vi "Volume Sievert_auto_RLC-CRZPhi.vi"() -> ()   [LabVIEW 2011]
uses:
  <vilib>/Utility/error.llb/DialogType.ctl
  <vilib>/DAQmx/write.llb/DAQmx Write (Digital Bool 1Line 1Point).vi
  <vilib>/DAQmx/create/channels.llb/DAQmx Create Channel (DO-Digital Output).vi
  <vilib>/DAQmx/miscellaneous.llb/DAQmx Fill In Error Info.vi
  <vilib>/Analysis/Matrix/Numeric/Conversions/Array To Matrix - RA.vi
  <vilib>/Analysis/Matrix/Numeric/Conversions/Matrix To Array - RM.vi
  <vilib>/Analysis/NI_AALPro.lvlib
  <vilib>/Analysis/Matrix/NI_Matrix.lvlib
  <vilib>/Analysis/NI_AALBase.lvlib
panel:
  out "S#1_auto":dbl
  out "S#01":dbl
  out "output array 3":u32[](array[numeric])
  out "PCh1 2":dbl[](array[numeric])
  out "tempo carga 2":dbl[](array[numeric])
  out "path RLC_mean 2":path
  out "MEASURE R [Ohm ]":dbl
  out "tempo carga":dbl[](array[numeric])
  out "PCh1":dbl[](array[numeric])
  out "output array 2":u32[](array[numeric])
  out "MEASURE C [F ]":dbl
  out "Automatico 2":dynamicdata(graph)
  out "termopar K 2":dbl format="%.3g"
  out "termopar K":string
  out "output NTC":dbl
  out "termopar K":dbl format="%.3g"
  out "path RLC_mean":path
  out "estagio 5":i32
  out "FIM":bool=TRUE
  out "limpo":i32
  in  "N fit":i32=5
  in  "ATM wait":u32
  in  "SET":i32
  in  "time subarray":dbl[](array[numeric])
  out "P cinetica mean 2":dbl format="%0.2f"
  out "T cinetica mean 3":dbl format="%0.2f"
  out "Time cinetica":dbl format="%0.2f"
  in  "T subarray 3":dbl[](array[numeric])
  in  "P T  index 2":i32
  in  "P subarray 2":dbl[](array[numeric])
  in  "Numeric":dbl=4.0
  in  "T subarray 2":dbl[](array[numeric])
  out "T cinetica mean 2":dbl format="%0.2f"
  out "P cinetica mean":dbl format="%0.2f"
  in  "P subarray":dbl[](array[numeric])
  in  "P T  index":i32
  out "T string":string
  out "P string":string
  out "path 2_cinetica":path
  out "Polynomial Coefficients 2":dbl[](array[numeric])
  out "Polynomial Coefficients":dbl[](array[numeric])
  in  "Count SET":i32=-1
  out "Set atual":i32
  out "mean pressure":dbl format="%.4p"
  out "Set number":i32
  in  "Tab Control":T1(tab)
  out "T":bool
  out "ZPf2":bool
  out "Pf2":bool
  out "Pit":bool
  out "ZPit":bool
  out "Camara":dbl(slide) scale=0.0..59.5 scale format="%#_3g"
  in  "Save manual":bool
  in  "Open Button":bool
  out "String 2":string
  in  "ATM":bool
  in  "Câmara":bool
  in  "Vácuo":bool
  in  "Entrada Gás":bool
  in  "Manual Ctrl":bool
  in  "stop":bool
  out "P-manual":dynamicdata(graph)
  in  "Clear":bool
  out "path":path
  in  "Nota":string
  in  "Sample name":string
  in  "File name":string
  out "Linear Model Graph":dbl[][](graph)
  out "Linear Model Graph 2":dbl[][](graph)
  in  "N to fit":i32=60
  out "N":i32
  out "Vácuo":bool
  out "Atm":bool
  out "Câmara":bool
  out "String_cinetica":string
  out "Vol Ref":dbl(slide) scale=0.0..60.0 scale format="%#_4f"
  out "Entrada gás":bool
  in  "Guardar\nCinetica":bool
  out "p fit":dbl format="%#_4g"
  out "T fit":dbl format="%#_4g"
  in  "Open Button 2":bool
  out "x >= y?":bool
  in  "seconds":dbl
  out "Elapsed Time (sec)":dbl format="%.1f"
  out "bar/N":dbl format="%#_4p"
  in  "correção NTC":dbl
  out "mean H2 sensor (V)":dbl format="%#_4p"
  out "Boolean 3":bool
  out "String 3":string
  out "T 2":bool
  out "ZPit 2":bool
  out "Pit 2":bool
  out "Pf2 2":bool
  out "ZPf2 2":bool
  out "Camara 2":dbl(slide) scale=0.0..18.0 scale format="%#_3g"
  out "Vácuo 2":bool
  out "Atm 2":bool
  out "Câmara 2":bool
  out "Vol Ref 3":dbl(slide) scale=0.0..50.0 scale format="%#_4f"
  out "Entrada gás 2":bool
  in  "Auto Ctrl":bool
  in  "Play Button":bool
  out "time stamp":timestamp format="%<%.2X>T"
  out "Time (sec)":dbl format="%.1f"
  in  "clear":bool
  out "Automatico":dynamicdata(graph)
  out "Linear P":T2(graph)
  out "Linear T":T2(graph)
  out "Contador":i32
  in  "STOP (bar/s)":dbl format="%#_5p"
  out "P (bar/s)":dbl format="%#_5p"
  out "bar/s":dbl format="%#_4p"
  out "P fit":dbl format="%#_4g"
  out "T fit":dbl format="%#_4g"
  out "x = y?":bool
  out "teste slope":i32
  in  "Set P auto":dbl
  in  "Step P":dbl=2.0
  in  "P_max":dbl=2.0
  in  "P_max camara":dbl=2.0
  out "Carga":bool=TRUE
  out "Descarga":bool
  out "String":string
  in  "P_min descarga":dbl
  in  "Boolean":bool
  in  "Array":dbl[](array[numeric])
  out "Boolean 2":bool
  out "Desc SET":i32
  in  "ZPf2 time":dbl=24.0
  in  "Ciclos":dbl
  out "Efetuados":dbl
  in  "patamar milliseconds to wait":u32=500
  in  "N fit patamar":i32=100
  in  "Step ZPit":dbl
  out "Read ZPit":bool
  in  "Estagio auto":i32
  out "mean H2 sensor":dbl format="%#_4p"
  in  "Ntest":i32=5
  in  "N fit 2":i32=100
  out "mean 18":dbl format="%.3p"
  out "mean 17":dbl format="%.3p"
  in  "C50L":bool
  in  "C50N":bool
  in  "C100L":bool
  in  "C100N":bool
  in  "C1KL":bool
  in  "C1KN":bool
  in  "C10KL":bool
  in  "C10KN":bool
  out "String 4":string
  in  "Combo Box":string(combo)
  in  "Refresh Button":bool
  in  "Close RLC 2":bool
  in  "RLC on/off":bool
  out "mean 16":dbl format="%.3p"
  out "mean 15":dbl format="%.3p"
  out "mean 14":dbl format="%.3p"
  out "mean 13":dbl format="%.3p"
  out "mean 12":dbl format="%.3p"
  out "mean 11":dbl format="%.3p"
  out "mean 10":dbl format="%.3p"
  out "mean 9":dbl format="%.3p"
  out "mean 8":dbl format="%.3p"
  out "mean 7":dbl format="%.3p"
  out "mean 6":dbl format="%.3p"
  out "mean 5":dbl format="%.3p"
  out "mean 4":dbl format="%.3p"
  out "mean 3":dbl format="%.3p"
  out "mean 2":dbl format="%.3p"
  out "mean":dbl format="%.3p"
  out "SET 2":dbl
  out "C-50-L":bool
  out "MEASURE B":dbl
  out "MEASURE A":dbl
  out "C-50-N":bool
  out "MEASURE B 2":dbl
  out "MEASURE A 2":dbl
  out "C-100-L":bool
  out "MEASURE B 3":dbl
  out "MEASURE A 3":dbl
  out "C-100-N":bool
  out "MEASURE B 4":dbl
  out "MEASURE A 4":dbl
  out "C-1K-L":bool
  out "MEASURE B 5":dbl
  out "MEASURE A 5":dbl
  out "C-1K-N":bool
  out "MEASURE B 6":dbl
  out "MEASURE A 6":dbl
  out "C-10K-L":bool
  out "MEASURE B 7":dbl
  out "MEASURE A 7":dbl
  out "C-10K-N":bool
  out "MEASURE B 8":dbl
  out "MEASURE A 8":dbl
  out "Z-50-L":bool
  out "MEASURE B 9":dbl
  out "MEASURE A 9":dbl
  out "Z-50-N":bool
  out "MEASURE B 10":dbl
  out "MEASURE A 10":dbl
  out "Z-100-L":bool
  out "MEASURE B 11":dbl
  out "MEASURE A 11":dbl
  out "Z-100-N":bool
  out "MEASURE B 12":dbl
  out "MEASURE A 12":dbl
  out "Z-1K-L":bool
  out "MEASURE B 13":dbl
  out "MEASURE A 13":dbl
  out "Z-1K-N":bool
  out "MEASURE B 14":dbl
  out "MEASURE A 14":dbl
  out "Z-10K-L":bool
  out "MEASURE B 15":dbl
  out "MEASURE A 15":dbl
  out "Z-10K-N":bool
  out "MEASURE B 16":dbl
  out "MEASURE A 16":dbl
  out "RLC300 - digimess":string
  in  "Time RLC":u32=5000
  in  "Ligar RLC":bool
  out "path RLC_completo":path
  out "Waveform Chart P 2":dbl[][](graph)
  out "Waveform Chart":dynamicdata(graph)
  in  "graph RLC":bool
  in  "Refresh Button 2":bool
  in  "Z50L":bool
  in  "Z50N":bool
  in  "Z100L":bool
  in  "Z100N":bool
  in  "Z1KL":bool
  in  "Z1KN":bool
  in  "Z10KL":bool
  in  "Z10KN":bool
  out "T(º) FIT":dbl
  out "Waveform Chart 2":dynamicdata(graph)
  out "XY Graph 2":cluster{"Value":dbl[], "Value":dbl[]}[](graph)
  in  "t-sivert01(s)":dbl
  out "dP/dt (bar/s)":dbl format="%#_5p"
  in  "Save - Sievert 01":bool
  in  "File name 2":string
  in  "Nota 01":string
  in  "Sample name 2":string
  in  "Save S#1":bool
  out "path 2":path
  out "Boolean 4":bool
  out "P(bar) FIT":dbl
  in  "ON/OFF":bool
  in  "Refresh Button 3":bool
  # "P vol ref"
  # "P Câmara"
  # "P vol ref"
  # "P Câmara"
  # "C ( F )"
  # "R ( Ohm )"
  # "Z ( Ohm )"
  # "Phase ( deg)"
types:
  T1 = enum32{"Manual", "Automatico", "RLC - CDH2", "Sievert 01"}
  T2 = cluster{"Real 2D Array":dbl[], "Best Linear Fit":dbl[]}[]
  T3 = enum16{"open", "replace", "create", "open or create", "replace or create", "replace or create with confirmation"}
  T4 = typedef "DialogType.ctl" = u16
  T5 = cluster{"Value":dbl[], "Best Polynomial Fit":dbl[]}
  T6 = cluster{"Value":dbl[], "Best Polynomial Fit":dbl[]}[]
  T7 = typedef "NI_Matrix.lvlib/RealMatrix.ctl" = dbl[][]
  T8 = cluster{"Real 2D Array":dbl[], "Real 2D Array":dbl[]}
  T9 = cluster{"Real 2D Array":dbl[], "Best Linear Fit":dbl[]}
  T10 = cluster{"Real 2D Array":dbl[], "Best Polynomial Fit":dbl[]}
  T11 = cluster{"Real 2D Array":dbl[], "Best Polynomial Fit":dbl[]}[]
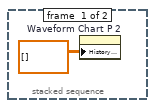
[diagram p7: hidden frame]
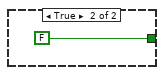
[diagram p12: hidden frame]
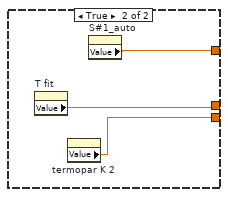
[diagram p15: hidden frame]
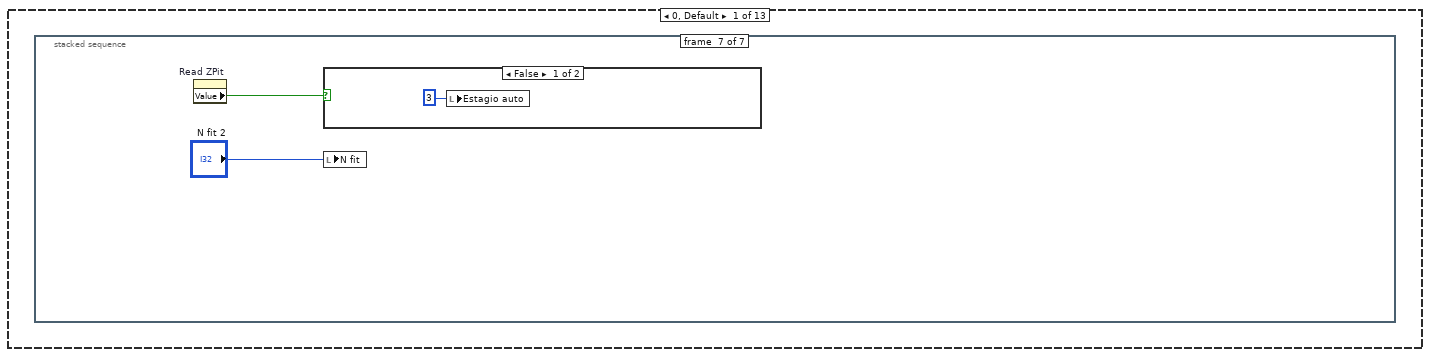
[diagram p20: hidden frame]
diagram:
  w2 = TRUE ("C1KN")
  (unwired) dbl[] [0.5, 1.0, 2.0, 3.0, 4.0, 5.0, 6.0, 7.0, 8.0, 9.0, 10.0, 11.0, 12.0, 13.0, 14.0, 15.0, 16.0, 17.0, 18.0, 19.0, 20.0, 30.0, 40.0, 50.0, 60.0, 70.0] ("Array")
  n1 = local write "N to fit"(5 ("Numeric")) -> ()
  n2 = local write "Step ZPit"(5.0 ("Step ZPit")) -> ()
  n3 = local write "Time RLC"(u32 5 ("Time RLC")) -> ()
  n4 = local write "Ciclos"(0.0 ("Ciclos")) -> ()
  n5 = local write "Desc SET"(0 ("Desc SET")) -> ()
  n6 = local write "Efetuados"(0.0 ("Efetuados")) -> ()
  n7 = local write "estagio 5"(0 ("estagio 5")) -> ()
  n8 = local write "teste slope"(0 ("teste slope")) -> ()
  n9 = local write "SET"(0 ("SET auto")) -> ()
  n10 = local write "limpo"(0 ("limpo")) -> ()
  n11 = local write "N fit"(5 ("N fit")) -> ()
  n12 = local write "ATM wait"(u32 4 ("ATM wait")) -> ()
  n13 = local write "Estagio auto"(0 ("Estagio auto")) -> ()
  n14 = local write "P T  index"(0 ("index")) -> ()
  n15 = local write "seconds"(2.0 ("seconds")) -> ()
  n16 = local write "C1KN"(w2) -> ()
  n17 = local write "Z1KN"(w2) -> ()
  n18 = local write "Read ZPit"(TRUE ("Read ZPit")) -> ()
  n19 = local write "Descarga"(FALSE ("Descarga")) -> ()
  n20 = local write "Carga"(TRUE ("Carga")) -> ()
  n21 = local write "FIM"(FALSE ("FIM")) -> ()
  n22 = local write "t-sivert01(s)"(10.0 ("t-sivert01(s)")) -> ()
  n23 = local write "P_max"(50.0 ("P_max")) -> ()
  n24 = local write "P_max camara"(25.0 ("P_max camara")) -> ()
  n25 = local write "correção NTC"(0.5 ("correção NTC")) -> ()
  n26 = local write "Set P auto"(0.5 ("Set P auto")) -> ()
  n27 = local write "P_min descarga"(0.025 ("P_min descarga")) -> ()
  n28 = local write "Array"(dbl[] [0.5, 1.0, 2.0, 3.0, 4.0, 4.0, 4.0, 4.0, 4.0, 4.0, 4.0, 5.0, 5.0, 5.0, 7.0, 10.0, 15.0, 20.0, 25.0, 25.0, 25.0, 30.0, 40.0, 50.0, 60.0, 70.0] ("Array")) -> ()
  n29 = local write "P subarray"(dbl[] [0.0, 1.0] ("subarray")) -> ()
  n30 = local write "T subarray 2"(dbl[] [0.0, 1.0] ("subarray")) -> ()
  n31 = local write "Combo Box"("rlc_read_cCN.py" ("Combo Box")) -> ()
  n32 = while {
    tunnel: path "C:/H2_Painel/painel_auto/RLC_CDH" ("Path") -> [w40]
    stop <- w52 stop-if-true
    n33 = property on="FIM" class="Bool (strict)"() -> ("Value"=w50:bool)  [unwired: 2 in, 2 out]
    n34 = property on="path" class="Path"() -> ("Value"=w47:path)  [unwired: 2 in, 2 out]
    n35 = case shown="True" "Ligar RLC" {
      tunnel: w40 -> [_ w231]
      frame False {
      }
      frame True {
        n36 = call "RLC_open.vi"("Path"=w231) -> ("String 2"=w232:string)  [unwired: 9 in, 1 out]
        n37 = local write "RLC300 - digimess"(w232) -> ()
      }
    }
    n38 = case shown="True" "RLC on/off" {
      tunnel: w40 -> [_ _]
      frame False {
      }
      frame True {
        n39 = call "RLC READ DINAMICO.vi"("Boolean"="graph RLC") -> ("MEASURE R [Ohm ]"=w66:dbl, "MEASURE C [F ]"=w65:dbl)  [unwired: 9 in]
        "MEASURE C [F ]" <- w65
        "MEASURE R [Ohm ]" <- w66
        n40 = Merge Signals(w65, w66) -> (→"Waveform Chart":dynamicdata)
        "String 4" <- "Combo Box"
      }
    }
    n41 = case shown="True" "Manual Ctrl" {
      tunnel: w40 -> [_ w1841]
      tunnel: "RLC on/off" -> [_ w1840]
      tunnel: [FALSE w1843] -> w42
      frame False {
      }
      frame True {
        w1855 = 0 ("polynomial order")
        n42 = case shown="True" "Save manual" {
          selector: "Save manual" -> [_ w2457]
          frame False {
          }
          frame True {
            n43 = feedback #1() -> (w2453:dbl)  [unwired: 1 in]
            n44 = Equal To 0?(x=w2453) -> (x = 0?=w2459:bool)
            n45 = stacked-sequence {
              tunnel: w2459 -> [_ w2475 _]
              tunnel: [_ w2474 _] -> w2455
              frame #0 {
                w2468 = i16 3 ("precision (6)")
                n46 = property on="T fit" class="DigNum (strict)"() -> ("Value"=w2470:dbl)  [unwired: 2 in, 2 out]
                n47 = property on="p fit" class="DigNum (strict)"() -> ("Value"=w2471:dbl)  [unwired: 2 in, 2 out]
                n48 = property on="termopar K" class="DigNum (strict)"() -> ("Value"=w2469:dbl)  [unwired: 2 in, 2 out]
                n49 = Number To Fractional String(number=w2470, precision (6)=w2468) -> (F-format string=→"T string":string)  [unwired: 2 in]
                n50 = Number To Fractional String(number=w2471, precision (6)=w2468) -> (F-format string=→"P string":string)  [unwired: 2 in]
                n51 = Number To Fractional String(number=w2469, precision (6)=w2468) -> (F-format string=→"termopar K":string)  [unwired: 2 in]
              }
              frame #1 {
                n52 = case shown="True" w2475 {
                  tunnel: [TRUE ("y") FALSE ("y")] -> w2474
                  frame False {
                    n53 = property on="path" class="Path"() -> ("Value"=w2479:path)  [unwired: 2 in, 2 out]
                    n54 = property on="P string" class="Str"() -> ("Value"=w2478:string)  [unwired: 2 in, 2 out]
                    n55 = Concatenate Strings(w2478, "\t") -> (w2476:string)
                    n56 = Open/Create/Replace File(file path (use dialog)=w2479, operation (0:open)=T3."open") -> (refnum out=w2483:refnum<file>, error out=w2482:errorcluster)  [unwired: 2 in, 3 out]
                    n57 = Set File Position(refnum=w2483, from (0:start)=enum16{"start", "end", "current"}."end", error in=w2482) -> (refnum out=w2485:refnum<file>, error out=w2486:errorcluster)  [unwired: 1 in]
                    n58 = Write to Text File(file (use dialog)=w2485, text=w2476, error in=w2486) -> (refnum out=w2481:refnum<file>, error out=w2480:errorcluster)  [unwired: 2 out]
                    n59 = Close File(refnum=w2481, error in=w2480) -> (error out=w2488:errorcluster)  [unwired: 1 out]
                    n60 = call <vilib>:"Simple Error Handler.vi"("error in (no error)"=w2488) -> ()  [unwired: 1 in, 8 out]
                  }
                  frame True {
                    w2491 = "\t"
                    n61 = property on="path" class="Path"() -> ("Value"=w2498:path)  [unwired: 2 in, 2 out]
                    n62 = property on="Count SET" class="DigNum (strict)"() -> ("Value"=w2494:i32)  [unwired: 2 in, 2 out]
                    n63 = Open/Create/Replace File(file path (use dialog)=w2498, operation (0:open)=T3."open") -> (refnum out=w2497:refnum<file>, error out=w2496:errorcluster)  [unwired: 2 in, 3 out]
                    n64 = Increment(x=w2494) -> (x+1=w2495:i32)
                    "Set atual" <- w2495
                    n65 = Set File Position(refnum=w2497, from (0:start)=enum16{"start", "end", "current"}."end", error in=w2496) -> (refnum out=w2506:refnum<file>, error out=w2507:errorcluster)  [unwired: 1 in]
                    n66 = Number To Decimal String(number=w2495) -> (decimal integer string=w2499:string)  [unwired: 1 in]
                    n67 = property on="termopar K" class="Str"() -> ("Value"=w2490:string)  [unwired: 2 in, 2 out]
                    n68 = property on="T string" class="Str"() -> ("Value"=w2492:string)  [unwired: 2 in, 2 out]
                    n69 = Concatenate Strings(w2492, w2491, w2490, "\r\n", w2499, w2491) -> (w2501:string)
                    n70 = Write to Text File(file (use dialog)=w2506, text=w2501, error in=w2507) -> (refnum out=w2504:refnum<file>, error out=w2503:errorcluster)  [unwired: 2 out]
                    n71 = Close File(refnum=w2504, error in=w2503) -> (error out=w2509:errorcluster)  [unwired: 1 out]
                    n72 = call <vilib>:"Simple Error Handler.vi"("error in (no error)"=w2509) -> ()  [unwired: 1 in, 8 out]
                    "T" <- TRUE ("T")
                  }
                }
              }
              frame #2 {
                n73 = property on="path" class="Path"() -> ("Value"=w2511:path)  [unwired: 2 in, 2 out]
                n74 = property on="Set atual" class="DigNum (strict)"() -> ("Value"=w2510:i32)  [unwired: 2 in, 2 out]
                n75 = local write "Count SET"(w2510) -> ()
                n76 = Read from Text File(file (use dialog)=w2511, count=-1 ("Count  3")) -> (refnum out=w2513:refnum<file>, text=w2512:string, error out=w2514:errorcluster)  [unwired: 2 in, 1 out]
                n77 = property on="String 2" class="Str"("Value"=w2512) -> ()  [unwired: 2 in, 2 out]
                n78 = Close File(refnum=w2513, error in=w2514) -> (error out=w2516:errorcluster)  [unwired: 1 out]
                n79 = call <vilib>:"Simple Error Handler.vi"("error in (no error)"=w2516) -> ()  [unwired: 1 in, 8 out]
              }
            }
            n80 = Implies(1:w2455, 2:w2457) -> (0:w2456:bool)
            n81 = Select(t=w2453, s=w2456, f=5.0 ("t")) -> (s? t:f=w2454:dbl)
            n82 = case shown="1" w2454 {
              frame 0, Default {
              }
              frame 1 {
                "ZPf2" <- TRUE ("ZPf2")
              }
              frame 2 {
                "Pf2" <- TRUE ("Pf2")
              }
              frame 3 {
                "Pit" <- TRUE ("Pit")
              }
              frame 4 {
                n83 = local write "T"(FALSE ("T")) -> ()
                "ZPit" <- TRUE ("ZPit")
              }
              frame 5 {
                w2466 = FALSE
                n84 = local write "Pit"(w2466) -> ()
                n85 = local write "ZPf2"(w2466) -> ()
                n86 = local write "ZPit"(w2466) -> ()
                n87 = local write "Pf2"(w2466) -> ()
              }
            }
            n88 = Decrement(x=w2454) -> (x-1=w2460:dbl)
            n89 = feedback-in #1(w2460) -> ()
          }
        }
        n90 = case shown="True" w1840 {
          tunnel: [FALSE ("Save manual") w2452] -> w1842
          tunnel: "Save manual" -> [_ w2452]
          frame False {
          }
          frame True {
          }
        }
        n91 = case shown="True" w1840 {
          tunnel: [FALSE w1860] -> w1843
          tunnel: w1842 -> [_ w1859]
          tunnel: w1841 -> [_ w1858]
          frame False {
          }
          frame True {
            n92 = flat-sequence {
              tunnel: w1858 -> [w1881]
              tunnel: w1859 -> [w1882]
              tunnel: [w1882] -> w1879
              tunnel: [w1881] -> w1878
              tunnel: [w1889] -> w1877
              tunnel: [w1890] -> w1876
              tunnel: [w1891] -> w1875
              tunnel: [w1892] -> w1874
              tunnel: [w1893] -> w1873
              tunnel: [w1894] -> w1872
              tunnel: [w1895] -> w1871
              tunnel: [w1897] -> w1870
              tunnel: [w1898] -> w1869
              tunnel: [w1899] -> w1868
              tunnel: [w1900] -> w1867
              tunnel: [w1901] -> w1866
              tunnel: [w1896] -> w1865
              tunnel: [w1888] -> w1864
              tunnel: [w1887] -> w1863
              tunnel: [w1886] -> w1862
              tunnel: [w1885] -> w1861
              tunnel: w1879 -> [w1884]
              tunnel: w1878 -> [w1883]
              tunnel: w1877 -> [w2399]
              tunnel: w1876 -> [w2398]
              tunnel: w1875 -> [w2397]
              tunnel: w1874 -> [w2396]
              tunnel: w1873 -> [w2395]
              tunnel: w1872 -> [w2394]
              tunnel: w1871 -> [w2393]
              tunnel: w1870 -> [w2392]
              tunnel: w1869 -> [w2391]
              tunnel: w1868 -> [w2390]
              tunnel: w1867 -> [w2389]
              tunnel: w1866 -> [w2388]
              tunnel: w1865 -> [w2387]
              tunnel: w1864 -> [w2400]
              tunnel: w1863 -> [w2401]
              tunnel: w1862 -> [w2402]
              tunnel: [w2385] -> w1860
              tunnel: w1861 -> [w2385]
              tunnel: [TRUE] -> w1857
              frame #0 {
                n93 = local write "graph RLC"(FALSE) -> ()
              }
              frame #1 {
                n94 = case shown="True" w1884 {
                  tunnel: [_ w1936] -> w1885
                  tunnel: w1883 -> [_ w1918]
                  tunnel: [_ w1917] -> w1886
                  tunnel: [_ w1916] -> w1887
                  tunnel: [_ w1915] -> w1888
                  tunnel: [_ w1914] -> w1889
                  tunnel: [_ w1913] -> w1890
                  tunnel: [_ w1912] -> w1891
                  tunnel: [_ w1911] -> w1892
                  tunnel: [_ w1910] -> w1893
                  tunnel: [_ w1909] -> w1894
                  tunnel: [_ w1908] -> w1895
                  tunnel: [_ w1907] -> w1896
                  tunnel: [_ w1906] -> w1897
                  tunnel: [_ w1905] -> w1898
                  tunnel: [_ w1904] -> w1899
                  tunnel: [_ w1903] -> w1900
                  tunnel: [_ w1902] -> w1901
                  frame False {
                  }
                  frame True {
                    n95 = for {
                      N: 5 -> [_]
                      tunnel: TRUE -> [w1959]
                      tunnel: FALSE -> [w1958]
                      tunnel: [w1957] -> w1936
                      tunnel: [w1956] -> w1934 mode=indexing
                      tunnel: [w1955] -> w1933 mode=indexing
                      tunnel: [w1954] -> w1932 mode=indexing
                      tunnel: [w1953] -> w1931 mode=indexing
                      tunnel: [w1952] -> w1930 mode=indexing
                      tunnel: [w1951] -> w1929 mode=indexing
                      tunnel: [w1950] -> w1928 mode=indexing
                      tunnel: [w1949] -> w1927 mode=indexing
                      tunnel: [w1948] -> w1926 mode=indexing
                      tunnel: [w1947] -> w1925 mode=indexing
                      tunnel: [w1946] -> w1924 mode=indexing
                      tunnel: [w1945] -> w1923 mode=indexing
                      tunnel: [w1944] -> w1922 mode=indexing
                      tunnel: [w1943] -> w1921 mode=indexing
                      tunnel: [w1942] -> w1920 mode=indexing
                      tunnel: [w1941] -> w1919 mode=indexing
                      tunnel: w1918 -> [w1940]
                      n96 = property on="path RLC_completo" class="Path"() -> ("Value"=w1939:path)  [unwired: 2 in, 2 out]
                      n97 = stacked-sequence {
                        tunnel: w1959 -> [_ w1984 w2009 w2034 w2059 w2084 w2109 w2134 w2157 w2182 w2209 w2232 w2259 w2284 w2309 w2332 w2359 _]
                        tunnel: w1958 -> [w1960 _ _ _ _ _ _ _ _ _ _ _ _ _ _ _ _ w2383]
                        tunnel: [_ _ _ _ _ _ _ _ _ _ _ _ _ _ _ _ _ TRUE] -> w1957
                        tunnel: [_ w1983 _ _ _ _ _ _ _ _ _ _ _ _ _ _ _ _] -> w1956
                        tunnel: [_ _ w2008 _ _ _ _ _ _ _ _ _ _ _ _ _ _ _] -> w1955
                        tunnel: [_ _ _ w2033 _ _ _ _ _ _ _ _ _ _ _ _ _ _] -> w1954
                        tunnel: [_ _ _ _ w2058 _ _ _ _ _ _ _ _ _ _ _ _ _] -> w1953
                        tunnel: [_ _ _ _ _ w2083 _ _ _ _ _ _ _ _ _ _ _ _] -> w1952
                        tunnel: [_ _ _ _ _ _ w2108 _ _ _ _ _ _ _ _ _ _ _] -> w1951
                        tunnel: [_ _ _ _ _ _ _ w2133 _ _ _ _ _ _ _ _ _ _] -> w1950
                        tunnel: [_ _ _ _ _ _ _ _ w2159 _ _ _ _ _ _ _ _ _] -> w1949
                        tunnel: [_ _ _ _ _ _ _ _ _ w2184 _ _ _ _ _ _ _ _] -> w1948
                        tunnel: [_ _ _ _ _ _ _ _ _ _ w2208 _ _ _ _ _ _ _] -> w1947
                        tunnel: [_ _ _ _ _ _ _ _ _ _ _ w2234 _ _ _ _ _ _] -> w1946
                        tunnel: [_ _ _ _ _ _ _ _ _ _ _ _ w2258 _ _ _ _ _] -> w1945
                        tunnel: [_ _ _ _ _ _ _ _ _ _ _ _ _ w2283 _ _ _ _] -> w1944
                        tunnel: [_ _ _ _ _ _ _ _ _ _ _ _ _ _ w2308 _ _ _] -> w1943
                        tunnel: [_ _ _ _ _ _ _ _ _ _ _ _ _ _ _ w2334 _ _] -> w1942
                        tunnel: [_ _ _ _ _ _ _ _ _ _ _ _ _ _ _ _ w2358 _] -> w1941
                        tunnel: w1940 -> [_ w1986 w2012 w2036 w2061 w2086 w2111 w2136 w2161 w2186 w2211 w2236 w2261 w2286 w2311 w2336 w2361 _]
                        tunnel: w1939 -> [w1962 w1985 w2011 w2035 w2060 w2085 w2110 w2135 w2160 w2185 w2210 w2235 w2260 w2285 w2310 w2335 w2360 _]
                        frame #0 {
                          w1963 = "\t"
                          n98 = local write "C-50-L"(w1960) -> ()
                          n99 = local write "C-50-N"(w1960) -> ()
                          n100 = local write "Z-50-L"(w1960) -> ()
                          n101 = local write "Z-50-N"(w1960) -> ()
                          n102 = local write "C-1K-L"(w1960) -> ()
                          n103 = local write "C-1K-N"(w1960) -> ()
                          n104 = local write "Z-1K-N"(w1960) -> ()
                          n105 = local write "Z-1K-L"(w1960) -> ()
                          n106 = local write "Z-100-L"(w1960) -> ()
                          n107 = local write "C-10K-L"(w1960) -> ()
                          n108 = local write "C-100-N"(w1960) -> ()
                          n109 = local write "C-10K-N"(w1960) -> ()
                          n110 = local write "Z-10K-N"(w1960) -> ()
                          n111 = local write "Z-10K-L"(w1960) -> ()
                          n112 = local write "Z-100-N"(w1960) -> ()
                          n113 = local write "C-100-L"(w1960) -> ()
                          n114 = Open/Create/Replace File(file path (use dialog)=w1962, operation (0:open)=T3."open") -> (refnum out=w1976:refnum<file>, error out=w1975:errorcluster)  [unwired: 2 in, 3 out]
                          n115 = Get Date/Time String(date format (0)=enum16{"short", "long", "abbreviated"}."short", want seconds? (F)=TRUE) -> (date string=w1968:string, time string=w1967:string)  [unwired: 1 in]
                          n116 = feedback #2() -> (w1961:dbl)  [unwired: 1 in]
                          n117 = local write "SET 2"(w1961) -> ()
                          n118 = Set File Position(refnum=w1976, from (0:start)=enum16{"start", "end", "current"}."end", error in=w1975) -> (refnum out=w1978:refnum<file>, error out=w1979:errorcluster)  [unwired: 1 in]
                          n119 = Number To Fractional String(number=w1961, precision (6)=i16 2) -> (F-format string=w1966:string)  [unwired: 2 in]
                          n120 = Add(x=w1961, y=0.2) -> (x+y=w1972:dbl)
                          n121 = feedback-in #2(w1972) -> ()
                          n122 = Concatenate Strings(w1966, w1963, w1968, w1963, w1967, w1963) -> (w1965:string)
                          n123 = Write to Text File(file (use dialog)=w1978, text=w1965, error in=w1979) -> (refnum out=w1974:refnum<file>, error out=w1973:errorcluster)  [unwired: 1 in, 1 out]
                          n124 = Close File(refnum=w1974, error in=w1973) -> (error out=w1981:errorcluster)  [unwired: 1 out]
                          n125 = call <vilib>:"Simple Error Handler.vi"("error in (no error)"=w1981) -> ()  [unwired: 1 in, 8 out]
                        }
                        frame #1 {
                          w1987 = "\t"
                          w2004 = i16 4 ("width (-)")
                          n126 = local write "C-50-L"(w1984) -> ()
                          n127 = Wait (ms)(milliseconds to wait=u32 5000) -> ()  [unwired: 1 out]
                          n128 = Open/Create/Replace File(file path (use dialog)=w1985, operation (0:open)=T3."open") -> (refnum out=w1996:refnum<file>, error out=w1995:errorcluster)  [unwired: 2 in, 3 out]
                          n129 = Set File Position(refnum=w1996, from (0:start)=enum16{"start", "end", "current"}."end", error in=w1995) -> (refnum out=w1998:refnum<file>, error out=w1999:errorcluster)  [unwired: 1 in]
                          n130 = call "RLC_read.vi"("Path"=w1986, "String"="cmd /c rlc_read_cAL.py") -> ("MEASURE A"=w1983:dbl, "MEASURE V [V]"=w2003:dbl, "MEASURE B"=w1982:dbl, "MEASURE I [A]"=w2002:dbl)  [unwired: 2 out]
                          n131 = Number To Engineering String(2:w2004, 4:w2002) -> (0:w1988:string)  [unwired: 2 in]
                          n132 = local write "MEASURE A"(w1983) -> ()
                          n133 = local write "MEASURE B"(w1982) -> ()
                          n134 = Number To Engineering String(2:w2004, 4:w2003) -> (0:w1989:string)  [unwired: 2 in]
                          n135 = Number To Engineering String(2:w2004, 4:w1983) -> (0:w1991:string)  [unwired: 2 in]
                          n136 = Number To Engineering String(2:w2004, 4:w1982) -> (0:w1990:string)  [unwired: 2 in]
                          n137 = Concatenate Strings(w1991, w1987, w1990, w1987, w1989, w1987, w1988, w1987) -> (w1992:string)
                          n138 = Write to Text File(file (use dialog)=w1998, text=w1992, error in=w1999) -> (refnum out=w1994:refnum<file>, error out=w1993:errorcluster)  [unwired: 1 in, 1 out]
                          n139 = Close File(refnum=w1994, error in=w1993) -> (error out=w2001:errorcluster)  [unwired: 1 out]
                          n140 = call <vilib>:"Simple Error Handler.vi"("error in (no error)"=w2001) -> ()  [unwired: 1 in, 8 out]
                        }
                        frame #2 {
                          w2015 = "\t"
                          w2029 = i16 4 ("width (-)")
                          n141 = local write "C-50-N"(w2009) -> ()
                          n142 = Wait (ms)(milliseconds to wait=u32 5000) -> ()  [unwired: 1 out]
                          n143 = Open/Create/Replace File(file path (use dialog)=w2011, operation (0:open)=T3."open") -> (refnum out=w2023:refnum<file>, error out=w2022:errorcluster)  [unwired: 2 in, 3 out]
                          n144 = Set File Position(refnum=w2023, from (0:start)=enum16{"start", "end", "current"}."end", error in=w2022) -> (refnum out=w2025:refnum<file>, error out=w2026:errorcluster)  [unwired: 1 in]
                          n145 = call "RLC_read.vi"("Path"=w2012, "String"="cmd /c rlc_read_cAN.py") -> ("MEASURE A"=w2008:dbl, "MEASURE V [V]"=w2014:dbl, "MEASURE B"=w2007:dbl, "MEASURE I [A]"=w2013:dbl)  [unwired: 2 out]
                          n146 = Number To Engineering String(2:w2029, 4:w2013) -> (0:w2016:string)  [unwired: 2 in]
                          n147 = local write "MEASURE A 2"(w2008) -> ()
                          n148 = local write "MEASURE B 2"(w2007) -> ()
                          n149 = Number To Engineering String(2:w2029, 4:w2014) -> (0:w2017:string)  [unwired: 2 in]
                          n150 = Number To Engineering String(2:w2029, 4:w2008) -> (0:w2019:string)  [unwired: 2 in]
                          n151 = Number To Engineering String(2:w2029, 4:w2007) -> (0:w2018:string)  [unwired: 2 in]
                          n152 = Concatenate Strings(w2019, w2015, w2018, w2015, w2017, w2015, w2016, w2015) -> (w2010:string)
                          n153 = Write to Text File(file (use dialog)=w2025, text=w2010, error in=w2026) -> (refnum out=w2021:refnum<file>, error out=w2020:errorcluster)  [unwired: 1 in, 1 out]
                          n154 = Close File(refnum=w2021, error in=w2020) -> (error out=w2028:errorcluster)  [unwired: 1 out]
                          n155 = call <vilib>:"Simple Error Handler.vi"("error in (no error)"=w2028) -> ()  [unwired: 1 in, 8 out]
                        }
                        frame #3 {
                          w2039 = "\t"
                          w2054 = i16 4 ("width (-)")
                          n156 = Wait (ms)(milliseconds to wait=u32 5000) -> ()  [unwired: 1 out]
                          n157 = local write "C-100-L"(w2034) -> ()
                          n158 = Open/Create/Replace File(file path (use dialog)=w2035, operation (0:open)=T3."open") -> (refnum out=w2048:refnum<file>, error out=w2047:errorcluster)  [unwired: 2 in, 3 out]
                          n159 = Set File Position(refnum=w2048, from (0:start)=enum16{"start", "end", "current"}."end", error in=w2047) -> (refnum out=w2050:refnum<file>, error out=w2051:errorcluster)  [unwired: 1 in]
                          n160 = call "RLC_read.vi"("Path"=w2036, "String"="cmd /c rlc_read_cBL.py") -> ("MEASURE A"=w2033:dbl, "MEASURE V [V]"=w2038:dbl, "MEASURE B"=w2032:dbl, "MEASURE I [A]"=w2037:dbl)  [unwired: 2 out]
                          n161 = Number To Engineering String(2:w2054, 4:w2037) -> (0:w2040:string)  [unwired: 2 in]
                          n162 = local write "MEASURE A 3"(w2033) -> ()
                          n163 = local write "MEASURE B 3"(w2032) -> ()
                          n164 = Number To Engineering String(2:w2054, 4:w2038) -> (0:w2041:string)  [unwired: 2 in]
                          n165 = Number To Engineering String(2:w2054, 4:w2033) -> (0:w2043:string)  [unwired: 2 in]
                          n166 = Number To Engineering String(2:w2054, 4:w2032) -> (0:w2042:string)  [unwired: 2 in]
                          n167 = Concatenate Strings(w2043, w2039, w2042, w2039, w2041, w2039, w2040, w2039) -> (w2044:string)
                          n168 = Write to Text File(file (use dialog)=w2050, text=w2044, error in=w2051) -> (refnum out=w2046:refnum<file>, error out=w2045:errorcluster)  [unwired: 1 in, 1 out]
                          n169 = Close File(refnum=w2046, error in=w2045) -> (error out=w2053:errorcluster)  [unwired: 1 out]
                          n170 = call <vilib>:"Simple Error Handler.vi"("error in (no error)"=w2053) -> ()  [unwired: 1 in, 8 out]
                        }
                        frame #4 {
                          w2064 = "\t"
                          w2079 = i16 4 ("width (-)")
                          n171 = Wait (ms)(milliseconds to wait=u32 5000) -> ()  [unwired: 1 out]
                          n172 = local write "C-100-N"(w2059) -> ()
                          n173 = Open/Create/Replace File(file path (use dialog)=w2060, operation (0:open)=T3."open") -> (refnum out=w2073:refnum<file>, error out=w2072:errorcluster)  [unwired: 2 in, 3 out]
                          n174 = Set File Position(refnum=w2073, from (0:start)=enum16{"start", "end", "current"}."end", error in=w2072) -> (refnum out=w2075:refnum<file>, error out=w2076:errorcluster)  [unwired: 1 in]
                          n175 = call "RLC_read.vi"("Path"=w2061, "String"="cmd /c rlc_read_cBN.py") -> ("MEASURE A"=w2058:dbl, "MEASURE V [V]"=w2063:dbl, "MEASURE B"=w2057:dbl, "MEASURE I [A]"=w2062:dbl)  [unwired: 2 out]
                          n176 = Number To Engineering String(2:w2079, 4:w2062) -> (0:w2065:string)  [unwired: 2 in]
                          n177 = local write "MEASURE A 4"(w2058) -> ()
                          n178 = local write "MEASURE B 4"(w2057) -> ()
                          n179 = Number To Engineering String(2:w2079, 4:w2063) -> (0:w2066:string)  [unwired: 2 in]
                          n180 = Number To Engineering String(2:w2079, 4:w2058) -> (0:w2068:string)  [unwired: 2 in]
                          n181 = Number To Engineering String(2:w2079, 4:w2057) -> (0:w2067:string)  [unwired: 2 in]
                          n182 = Concatenate Strings(w2068, w2064, w2067, w2064, w2066, w2064, w2065, w2064) -> (w2069:string)
                          n183 = Write to Text File(file (use dialog)=w2075, text=w2069, error in=w2076) -> (refnum out=w2071:refnum<file>, error out=w2070:errorcluster)  [unwired: 1 in, 1 out]
                          n184 = Close File(refnum=w2071, error in=w2070) -> (error out=w2078:errorcluster)  [unwired: 1 out]
                          n185 = call <vilib>:"Simple Error Handler.vi"("error in (no error)"=w2078) -> ()  [unwired: 1 in, 8 out]
                        }
                        frame #5 {
                          w2104 = "\t"
                          w2089 = i16 4 ("width (-)")
                          n186 = local write "C-1K-L"(w2084) -> ()
                          n187 = Wait (ms)(milliseconds to wait=u32 5000) -> ()  [unwired: 1 out]
                          n188 = Open/Create/Replace File(file path (use dialog)=w2085, operation (0:open)=T3."open") -> (refnum out=w2095:refnum<file>, error out=w2096:errorcluster)  [unwired: 2 in, 3 out]
                          n189 = Set File Position(refnum=w2095, from (0:start)=enum16{"start", "end", "current"}."end", error in=w2096) -> (refnum out=w2093:refnum<file>, error out=w2092:errorcluster)  [unwired: 1 in]
                          n190 = call "RLC_read.vi"("Path"=w2086, "String"="cmd /c rlc_read_cCL.py") -> ("MEASURE A"=w2083:dbl, "MEASURE V [V]"=w2088:dbl, "MEASURE B"=w2082:dbl, "MEASURE I [A]"=w2087:dbl)  [unwired: 2 out]
                          n191 = Number To Engineering String(2:w2089, 4:w2087) -> (0:w2103:string)  [unwired: 2 in]
                          n192 = local write "MEASURE A 5"(w2083) -> ()
                          n193 = local write "MEASURE B 5"(w2082) -> ()
                          n194 = Number To Engineering String(2:w2089, 4:w2088) -> (0:w2102:string)  [unwired: 2 in]
                          n195 = Number To Engineering String(2:w2089, 4:w2083) -> (0:w2100:string)  [unwired: 2 in]
                          n196 = Number To Engineering String(2:w2089, 4:w2082) -> (0:w2101:string)  [unwired: 2 in]
                          n197 = Concatenate Strings(w2100, w2104, w2101, w2104, w2102, w2104, w2103, w2104) -> (w2099:string)
                          n198 = Write to Text File(file (use dialog)=w2093, text=w2099, error in=w2092) -> (refnum out=w2097:refnum<file>, error out=w2098:errorcluster)  [unwired: 1 in, 1 out]
                          n199 = Close File(refnum=w2097, error in=w2098) -> (error out=w2090:errorcluster)  [unwired: 1 out]
                          n200 = call <vilib>:"Simple Error Handler.vi"("error in (no error)"=w2090) -> ()  [unwired: 1 in, 8 out]
                        }
                        frame #6 {
                          w2129 = "\t"
                          w2114 = i16 4 ("width (-)")
                          n201 = local write "C-1K-N"(w2109) -> ()
                          n202 = Wait (ms)(milliseconds to wait=u32 5000) -> ()  [unwired: 1 out]
                          n203 = Open/Create/Replace File(file path (use dialog)=w2110, operation (0:open)=T3."open") -> (refnum out=w2120:refnum<file>, error out=w2121:errorcluster)  [unwired: 2 in, 3 out]
                          n204 = Set File Position(refnum=w2120, from (0:start)=enum16{"start", "end", "current"}."end", error in=w2121) -> (refnum out=w2118:refnum<file>, error out=w2117:errorcluster)  [unwired: 1 in]
                          n205 = call "RLC_read.vi"("Path"=w2111, "String"="cmd /c rlc_read_cCN.py") -> ("MEASURE A"=w2108:dbl, "MEASURE V [V]"=w2113:dbl, "MEASURE B"=w2107:dbl, "MEASURE I [A]"=w2112:dbl)  [unwired: 2 out]
                          n206 = Number To Engineering String(2:w2114, 4:w2112) -> (0:w2128:string)  [unwired: 2 in]
                          n207 = local write "MEASURE A 6"(w2108) -> ()
                          n208 = local write "MEASURE B 6"(w2107) -> ()
                          n209 = Number To Engineering String(2:w2114, 4:w2113) -> (0:w2127:string)  [unwired: 2 in]
                          n210 = Number To Engineering String(2:w2114, 4:w2108) -> (0:w2125:string)  [unwired: 2 in]
                          n211 = Number To Engineering String(2:w2114, 4:w2107) -> (0:w2126:string)  [unwired: 2 in]
                          n212 = Concatenate Strings(w2125, w2129, w2126, w2129, w2127, w2129, w2128, w2129) -> (w2124:string)
                          n213 = Write to Text File(file (use dialog)=w2118, text=w2124, error in=w2117) -> (refnum out=w2122:refnum<file>, error out=w2123:errorcluster)  [unwired: 1 in, 1 out]
                          n214 = Close File(refnum=w2122, error in=w2123) -> (error out=w2115:errorcluster)  [unwired: 1 out]
                          n215 = call <vilib>:"Simple Error Handler.vi"("error in (no error)"=w2115) -> ()  [unwired: 1 in, 8 out]
                        }
                        frame #7 {
                          w2139 = "\t"
                          w2154 = i16 4 ("width (-)")
                          n216 = Wait (ms)(milliseconds to wait=u32 5000) -> ()  [unwired: 1 out]
                          n217 = local write "C-10K-L"(w2134) -> ()
                          n218 = Open/Create/Replace File(file path (use dialog)=w2135, operation (0:open)=T3."open") -> (refnum out=w2148:refnum<file>, error out=w2147:errorcluster)  [unwired: 2 in, 3 out]
                          n219 = Set File Position(refnum=w2148, from (0:start)=enum16{"start", "end", "current"}."end", error in=w2147) -> (refnum out=w2150:refnum<file>, error out=w2151:errorcluster)  [unwired: 1 in]
                          n220 = call "RLC_read.vi"("Path"=w2136, "String"="cmd /c rlc_read_cDL.py") -> ("MEASURE A"=w2133:dbl, "MEASURE V [V]"=w2138:dbl, "MEASURE B"=w2132:dbl, "MEASURE I [A]"=w2137:dbl)  [unwired: 2 out]
                          n221 = Number To Engineering String(2:w2154, 4:w2137) -> (0:w2140:string)  [unwired: 2 in]
                          n222 = local write "MEASURE A 7"(w2133) -> ()
                          n223 = local write "MEASURE B 7"(w2132) -> ()
                          n224 = Number To Engineering String(2:w2154, 4:w2138) -> (0:w2141:string)  [unwired: 2 in]
                          n225 = Number To Engineering String(2:w2154, 4:w2133) -> (0:w2143:string)  [unwired: 2 in]
                          n226 = Number To Engineering String(2:w2154, 4:w2132) -> (0:w2142:string)  [unwired: 2 in]
                          n227 = Concatenate Strings(w2143, w2139, w2142, w2139, w2141, w2139, w2140, w2139) -> (w2144:string)
                          n228 = Write to Text File(file (use dialog)=w2150, text=w2144, error in=w2151) -> (refnum out=w2146:refnum<file>, error out=w2145:errorcluster)  [unwired: 1 in, 1 out]
                          n229 = Close File(refnum=w2146, error in=w2145) -> (error out=w2153:errorcluster)  [unwired: 1 out]
                          n230 = call <vilib>:"Simple Error Handler.vi"("error in (no error)"=w2153) -> ()  [unwired: 1 in, 8 out]
                        }
                        frame #8 {
                          w2164 = "\t"
                          w2179 = i16 4 ("width (-)")
                          n231 = Wait (ms)(milliseconds to wait=u32 5000) -> ()  [unwired: 1 out]
                          n232 = local write "C-10K-N"(w2157) -> ()
                          n233 = Open/Create/Replace File(file path (use dialog)=w2160, operation (0:open)=T3."open") -> (refnum out=w2173:refnum<file>, error out=w2172:errorcluster)  [unwired: 2 in, 3 out]
                          n234 = Set File Position(refnum=w2173, from (0:start)=enum16{"start", "end", "current"}."end", error in=w2172) -> (refnum out=w2175:refnum<file>, error out=w2176:errorcluster)  [unwired: 1 in]
                          n235 = call "RLC_read.vi"("Path"=w2161, "String"="cmd /c rlc_read_cDN.py") -> ("MEASURE A"=w2159:dbl, "MEASURE V [V]"=w2163:dbl, "MEASURE B"=w2158:dbl, "MEASURE I [A]"=w2162:dbl)  [unwired: 2 out]
                          n236 = Number To Engineering String(2:w2179, 4:w2162) -> (0:w2165:string)  [unwired: 2 in]
                          n237 = local write "MEASURE A 8"(w2159) -> ()
                          n238 = local write "MEASURE B 8"(w2158) -> ()
                          n239 = Number To Engineering String(2:w2179, 4:w2163) -> (0:w2166:string)  [unwired: 2 in]
                          n240 = Number To Engineering String(2:w2179, 4:w2159) -> (0:w2168:string)  [unwired: 2 in]
                          n241 = Number To Engineering String(2:w2179, 4:w2158) -> (0:w2167:string)  [unwired: 2 in]
                          n242 = Concatenate Strings(w2168, w2164, w2167, w2164, w2166, w2164, w2165, w2164) -> (w2169:string)
                          n243 = Write to Text File(file (use dialog)=w2175, text=w2169, error in=w2176) -> (refnum out=w2171:refnum<file>, error out=w2170:errorcluster)  [unwired: 1 in, 1 out]
                          n244 = Close File(refnum=w2171, error in=w2170) -> (error out=w2178:errorcluster)  [unwired: 1 out]
                          n245 = call <vilib>:"Simple Error Handler.vi"("error in (no error)"=w2178) -> ()  [unwired: 1 in, 8 out]
                        }
                        frame #9 {
                          w2189 = "\t"
                          w2204 = i16 4 ("width (-)")
                          n246 = local write "Z-50-L"(w2182) -> ()
                          n247 = Wait (ms)(milliseconds to wait=u32 5000) -> ()  [unwired: 1 out]
                          n248 = Open/Create/Replace File(file path (use dialog)=w2185, operation (0:open)=T3."open") -> (refnum out=w2198:refnum<file>, error out=w2197:errorcluster)  [unwired: 2 in, 3 out]
                          n249 = Set File Position(refnum=w2198, from (0:start)=enum16{"start", "end", "current"}."end", error in=w2197) -> (refnum out=w2200:refnum<file>, error out=w2201:errorcluster)  [unwired: 1 in]
                          n250 = call "RLC_read.vi"("Path"=w2186, "String"="cmd /c rlc_read_ZAL.py") -> ("MEASURE A"=w2184:dbl, "MEASURE V [V]"=w2188:dbl, "MEASURE B"=w2183:dbl, "MEASURE I [A]"=w2187:dbl)  [unwired: 2 out]
                          n251 = Number To Engineering String(2:w2204, 4:w2187) -> (0:w2190:string)  [unwired: 2 in]
                          n252 = local write "MEASURE A 9"(w2184) -> ()
                          n253 = local write "MEASURE B 9"(w2183) -> ()
                          n254 = Number To Engineering String(2:w2204, 4:w2188) -> (0:w2191:string)  [unwired: 2 in]
                          n255 = Number To Engineering String(2:w2204, 4:w2184) -> (0:w2193:string)  [unwired: 2 in]
                          n256 = Number To Engineering String(2:w2204, 4:w2183) -> (0:w2192:string)  [unwired: 2 in]
                          n257 = Concatenate Strings(w2193, w2189, w2192, w2189, w2191, w2189, w2190, w2189) -> (w2194:string)
                          n258 = Write to Text File(file (use dialog)=w2200, text=w2194, error in=w2201) -> (refnum out=w2196:refnum<file>, error out=w2195:errorcluster)  [unwired: 1 in, 1 out]
                          n259 = Close File(refnum=w2196, error in=w2195) -> (error out=w2203:errorcluster)  [unwired: 1 out]
                          n260 = call <vilib>:"Simple Error Handler.vi"("error in (no error)"=w2203) -> ()  [unwired: 1 in, 8 out]
                        }
                        frame #10 {
                          w2214 = "\t"
                          w2229 = i16 4 ("width (-)")
                          n261 = local write "Z-50-N"(w2209) -> ()
                          n262 = Wait (ms)(milliseconds to wait=u32 5000) -> ()  [unwired: 1 out]
                          n263 = Open/Create/Replace File(file path (use dialog)=w2210, operation (0:open)=T3."open") -> (refnum out=w2223:refnum<file>, error out=w2222:errorcluster)  [unwired: 2 in, 3 out]
                          n264 = Set File Position(refnum=w2223, from (0:start)=enum16{"start", "end", "current"}."end", error in=w2222) -> (refnum out=w2225:refnum<file>, error out=w2226:errorcluster)  [unwired: 1 in]
                          n265 = call "RLC_read.vi"("Path"=w2211, "String"="cmd /c rlc_read_ZAN.py") -> ("MEASURE A"=w2208:dbl, "MEASURE V [V]"=w2213:dbl, "MEASURE B"=w2207:dbl, "MEASURE I [A]"=w2212:dbl)  [unwired: 2 out]
                          n266 = Number To Engineering String(2:w2229, 4:w2212) -> (0:w2215:string)  [unwired: 2 in]
                          n267 = local write "MEASURE A 10"(w2208) -> ()
                          n268 = local write "MEASURE B 10"(w2207) -> ()
                          n269 = Number To Engineering String(2:w2229, 4:w2213) -> (0:w2216:string)  [unwired: 2 in]
                          n270 = Number To Engineering String(2:w2229, 4:w2208) -> (0:w2218:string)  [unwired: 2 in]
                          n271 = Number To Engineering String(2:w2229, 4:w2207) -> (0:w2217:string)  [unwired: 2 in]
                          n272 = Concatenate Strings(w2218, w2214, w2217, w2214, w2216, w2214, w2215, w2214) -> (w2219:string)
                          n273 = Write to Text File(file (use dialog)=w2225, text=w2219, error in=w2226) -> (refnum out=w2221:refnum<file>, error out=w2220:errorcluster)  [unwired: 1 in, 1 out]
                          n274 = Close File(refnum=w2221, error in=w2220) -> (error out=w2228:errorcluster)  [unwired: 1 out]
                          n275 = call <vilib>:"Simple Error Handler.vi"("error in (no error)"=w2228) -> ()  [unwired: 1 in, 8 out]
                        }
                        frame #11 {
                          w2239 = "\t"
                          w2254 = i16 4 ("width (-)")
                          n276 = Wait (ms)(milliseconds to wait=u32 5000) -> ()  [unwired: 1 out]
                          n277 = local write "Z-100-L"(w2232) -> ()
                          n278 = Open/Create/Replace File(file path (use dialog)=w2235, operation (0:open)=T3."open") -> (refnum out=w2248:refnum<file>, error out=w2247:errorcluster)  [unwired: 2 in, 3 out]
                          n279 = Set File Position(refnum=w2248, from (0:start)=enum16{"start", "end", "current"}."end", error in=w2247) -> (refnum out=w2250:refnum<file>, error out=w2251:errorcluster)  [unwired: 1 in]
                          n280 = call "RLC_read.vi"("Path"=w2236, "String"="cmd /c rlc_read_ZBL.py") -> ("MEASURE A"=w2234:dbl, "MEASURE V [V]"=w2238:dbl, "MEASURE B"=w2233:dbl, "MEASURE I [A]"=w2237:dbl)  [unwired: 2 out]
                          n281 = Number To Engineering String(2:w2254, 4:w2237) -> (0:w2240:string)  [unwired: 2 in]
                          n282 = local write "MEASURE A 11"(w2234) -> ()
                          n283 = local write "MEASURE B 11"(w2233) -> ()
                          n284 = Number To Engineering String(2:w2254, 4:w2238) -> (0:w2241:string)  [unwired: 2 in]
                          n285 = Number To Engineering String(2:w2254, 4:w2234) -> (0:w2243:string)  [unwired: 2 in]
                          n286 = Number To Engineering String(2:w2254, 4:w2233) -> (0:w2242:string)  [unwired: 2 in]
                          n287 = Concatenate Strings(w2243, w2239, w2242, w2239, w2241, w2239, w2240, w2239) -> (w2244:string)
                          n288 = Write to Text File(file (use dialog)=w2250, text=w2244, error in=w2251) -> (refnum out=w2246:refnum<file>, error out=w2245:errorcluster)  [unwired: 1 in, 1 out]
                          n289 = Close File(refnum=w2246, error in=w2245) -> (error out=w2253:errorcluster)  [unwired: 1 out]
                          n290 = call <vilib>:"Simple Error Handler.vi"("error in (no error)"=w2253) -> ()  [unwired: 1 in, 8 out]
                        }
                        frame #12 {
                          w2264 = "\t"
                          w2279 = i16 4 ("width (-)")
                          n291 = Wait (ms)(milliseconds to wait=u32 5000) -> ()  [unwired: 1 out]
                          n292 = local write "Z-100-N"(w2259) -> ()
                          n293 = Open/Create/Replace File(file path (use dialog)=w2260, operation (0:open)=T3."open") -> (refnum out=w2273:refnum<file>, error out=w2272:errorcluster)  [unwired: 2 in, 3 out]
                          n294 = Set File Position(refnum=w2273, from (0:start)=enum16{"start", "end", "current"}."end", error in=w2272) -> (refnum out=w2275:refnum<file>, error out=w2276:errorcluster)  [unwired: 1 in]
                          n295 = call "RLC_read.vi"("Path"=w2261, "String"="cmd /c rlc_read_ZBN.py") -> ("MEASURE A"=w2258:dbl, "MEASURE V [V]"=w2263:dbl, "MEASURE B"=w2257:dbl, "MEASURE I [A]"=w2262:dbl)  [unwired: 2 out]
                          n296 = Number To Engineering String(2:w2279, 4:w2262) -> (0:w2265:string)  [unwired: 2 in]
                          n297 = local write "MEASURE A 12"(w2258) -> ()
                          n298 = local write "MEASURE B 12"(w2257) -> ()
                          n299 = Number To Engineering String(2:w2279, 4:w2263) -> (0:w2266:string)  [unwired: 2 in]
                          n300 = Number To Engineering String(2:w2279, 4:w2258) -> (0:w2268:string)  [unwired: 2 in]
                          n301 = Number To Engineering String(2:w2279, 4:w2257) -> (0:w2267:string)  [unwired: 2 in]
                          n302 = Concatenate Strings(w2268, w2264, w2267, w2264, w2266, w2264, w2265, w2264) -> (w2269:string)
                          n303 = Write to Text File(file (use dialog)=w2275, text=w2269, error in=w2276) -> (refnum out=w2271:refnum<file>, error out=w2270:errorcluster)  [unwired: 1 in, 1 out]
                          n304 = Close File(refnum=w2271, error in=w2270) -> (error out=w2278:errorcluster)  [unwired: 1 out]
                          n305 = call <vilib>:"Simple Error Handler.vi"("error in (no error)"=w2278) -> ()  [unwired: 1 in, 8 out]
                        }
                        frame #13 {
                          w2289 = "\t"
                          w2304 = i16 4 ("width (-)")
                          n306 = local write "Z-1K-L"(w2284) -> ()
                          n307 = Wait (ms)(milliseconds to wait=u32 5000) -> ()  [unwired: 1 out]
                          n308 = Open/Create/Replace File(file path (use dialog)=w2285, operation (0:open)=T3."open") -> (refnum out=w2298:refnum<file>, error out=w2297:errorcluster)  [unwired: 2 in, 3 out]
                          n309 = Set File Position(refnum=w2298, from (0:start)=enum16{"start", "end", "current"}."end", error in=w2297) -> (refnum out=w2300:refnum<file>, error out=w2301:errorcluster)  [unwired: 1 in]
                          n310 = call "RLC_read.vi"("Path"=w2286, "String"="cmd /c rlc_read_ZCL.py") -> ("MEASURE A"=w2283:dbl, "MEASURE V [V]"=w2288:dbl, "MEASURE B"=w2282:dbl, "MEASURE I [A]"=w2287:dbl)  [unwired: 2 out]
                          n311 = Number To Engineering String(2:w2304, 4:w2287) -> (0:w2290:string)  [unwired: 2 in]
                          n312 = local write "MEASURE A 13"(w2283) -> ()
                          n313 = local write "MEASURE B 13"(w2282) -> ()
                          n314 = Number To Engineering String(2:w2304, 4:w2288) -> (0:w2291:string)  [unwired: 2 in]
                          n315 = Number To Engineering String(2:w2304, 4:w2283) -> (0:w2293:string)  [unwired: 2 in]
                          n316 = Number To Engineering String(2:w2304, 4:w2282) -> (0:w2292:string)  [unwired: 2 in]
                          n317 = Concatenate Strings(w2293, w2289, w2292, w2289, w2291, w2289, w2290, w2289) -> (w2294:string)
                          n318 = Write to Text File(file (use dialog)=w2300, text=w2294, error in=w2301) -> (refnum out=w2296:refnum<file>, error out=w2295:errorcluster)  [unwired: 1 in, 1 out]
                          n319 = Close File(refnum=w2296, error in=w2295) -> (error out=w2303:errorcluster)  [unwired: 1 out]
                          n320 = call <vilib>:"Simple Error Handler.vi"("error in (no error)"=w2303) -> ()  [unwired: 1 in, 8 out]
                        }
                        frame #14 {
                          w2314 = "\t"
                          w2329 = i16 4 ("width (-)")
                          n321 = local write "Z-1K-N"(w2309) -> ()
                          n322 = Wait (ms)(milliseconds to wait=u32 5000) -> ()  [unwired: 1 out]
                          n323 = Open/Create/Replace File(file path (use dialog)=w2310, operation (0:open)=T3."open") -> (refnum out=w2323:refnum<file>, error out=w2322:errorcluster)  [unwired: 2 in, 3 out]
                          n324 = Set File Position(refnum=w2323, from (0:start)=enum16{"start", "end", "current"}."end", error in=w2322) -> (refnum out=w2325:refnum<file>, error out=w2326:errorcluster)  [unwired: 1 in]
                          n325 = call "RLC_read.vi"("Path"=w2311, "String"="cmd /c rlc_read_ZCN.py") -> ("MEASURE A"=w2308:dbl, "MEASURE V [V]"=w2313:dbl, "MEASURE B"=w2307:dbl, "MEASURE I [A]"=w2312:dbl)  [unwired: 2 out]
                          n326 = Number To Engineering String(2:w2329, 4:w2312) -> (0:w2315:string)  [unwired: 2 in]
                          n327 = local write "MEASURE A 14"(w2308) -> ()
                          n328 = local write "MEASURE B 14"(w2307) -> ()
                          n329 = Number To Engineering String(2:w2329, 4:w2313) -> (0:w2316:string)  [unwired: 2 in]
                          n330 = Number To Engineering String(2:w2329, 4:w2308) -> (0:w2318:string)  [unwired: 2 in]
                          n331 = Number To Engineering String(2:w2329, 4:w2307) -> (0:w2317:string)  [unwired: 2 in]
                          n332 = Concatenate Strings(w2318, w2314, w2317, w2314, w2316, w2314, w2315, w2314) -> (w2319:string)
                          n333 = Write to Text File(file (use dialog)=w2325, text=w2319, error in=w2326) -> (refnum out=w2321:refnum<file>, error out=w2320:errorcluster)  [unwired: 1 in, 1 out]
                          n334 = Close File(refnum=w2321, error in=w2320) -> (error out=w2328:errorcluster)  [unwired: 1 out]
                          n335 = call <vilib>:"Simple Error Handler.vi"("error in (no error)"=w2328) -> ()  [unwired: 1 in, 8 out]
                        }
                        frame #15 {
                          w2339 = "\t"
                          w2354 = i16 4 ("width (-)")
                          n336 = Wait (ms)(milliseconds to wait=u32 5000) -> ()  [unwired: 1 out]
                          n337 = local write "Z-10K-L"(w2332) -> ()
                          n338 = Open/Create/Replace File(file path (use dialog)=w2335, operation (0:open)=T3."open") -> (refnum out=w2348:refnum<file>, error out=w2347:errorcluster)  [unwired: 2 in, 3 out]
                          n339 = Set File Position(refnum=w2348, from (0:start)=enum16{"start", "end", "current"}."end", error in=w2347) -> (refnum out=w2350:refnum<file>, error out=w2351:errorcluster)  [unwired: 1 in]
                          n340 = call "RLC_read.vi"("Path"=w2336, "String"="cmd /c rlc_read_ZDL.py") -> ("MEASURE A"=w2334:dbl, "MEASURE V [V]"=w2338:dbl, "MEASURE B"=w2333:dbl, "MEASURE I [A]"=w2337:dbl)  [unwired: 2 out]
                          n341 = Number To Engineering String(2:w2354, 4:w2337) -> (0:w2340:string)  [unwired: 2 in]
                          n342 = local write "MEASURE A 15"(w2334) -> ()
                          n343 = local write "MEASURE B 15"(w2333) -> ()
                          n344 = Number To Engineering String(2:w2354, 4:w2338) -> (0:w2341:string)  [unwired: 2 in]
                          n345 = Number To Engineering String(2:w2354, 4:w2334) -> (0:w2343:string)  [unwired: 2 in]
                          n346 = Number To Engineering String(2:w2354, 4:w2333) -> (0:w2342:string)  [unwired: 2 in]
                          n347 = Concatenate Strings(w2343, w2339, w2342, w2339, w2341, w2339, w2340, w2339) -> (w2344:string)
                          n348 = Write to Text File(file (use dialog)=w2350, text=w2344, error in=w2351) -> (refnum out=w2346:refnum<file>, error out=w2345:errorcluster)  [unwired: 1 in, 1 out]
                          n349 = Close File(refnum=w2346, error in=w2345) -> (error out=w2353:errorcluster)  [unwired: 1 out]
                          n350 = call <vilib>:"Simple Error Handler.vi"("error in (no error)"=w2353) -> ()  [unwired: 1 in, 8 out]
                        }
                        frame #16 {
                          w2365 = "\t"
                          w2380 = i16 4 ("width (-)")
                          n351 = Wait (ms)(milliseconds to wait=u32 5000) -> ()  [unwired: 1 out]
                          n352 = local write "Z-10K-N"(w2359) -> ()
                          n353 = Open/Create/Replace File(file path (use dialog)=w2360, operation (0:open)=T3."open") -> (refnum out=w2374:refnum<file>, error out=w2373:errorcluster)  [unwired: 2 in, 3 out]
                          n354 = Set File Position(refnum=w2374, from (0:start)=enum16{"start", "end", "current"}."end", error in=w2373) -> (refnum out=w2376:refnum<file>, error out=w2377:errorcluster)  [unwired: 1 in]
                          n355 = call "RLC_read.vi"("Path"=w2361, "String"="cmd /c rlc_read_ZDN.py") -> ("MEASURE A"=w2358:dbl, "MEASURE V [V]"=w2364:dbl, "MEASURE B"=w2357:dbl, "MEASURE I [A]"=w2363:dbl)  [unwired: 2 out]
                          n356 = Number To Engineering String(2:w2380, 4:w2363) -> (0:w2366:string)  [unwired: 2 in]
                          n357 = local write "MEASURE A 16"(w2358) -> ()
                          n358 = local write "MEASURE B 16"(w2357) -> ()
                          n359 = Number To Engineering String(2:w2380, 4:w2364) -> (0:w2367:string)  [unwired: 2 in]
                          n360 = Number To Engineering String(2:w2380, 4:w2358) -> (0:w2369:string)  [unwired: 2 in]
                          n361 = Number To Engineering String(2:w2380, 4:w2357) -> (0:w2368:string)  [unwired: 2 in]
                          n362 = Concatenate Strings(w2369, w2365, w2368, w2365, w2367, w2365, w2366, w2365, "\r\n") -> (w2370:string)
                          n363 = Write to Text File(file (use dialog)=w2376, text=w2370, error in=w2377) -> (refnum out=w2372:refnum<file>, error out=w2371:errorcluster)  [unwired: 1 in, 1 out]
                          n364 = Close File(refnum=w2372, error in=w2371) -> (error out=w2379:errorcluster)  [unwired: 1 out]
                          n365 = call <vilib>:"Simple Error Handler.vi"("error in (no error)"=w2379) -> ()  [unwired: 1 in, 8 out]
                        }
                        frame #17 {
                          n366 = local write "Z-50-N"(w2383) -> ()
                          n367 = local write "Z-50-L"(w2383) -> ()
                          n368 = local write "C-1K-N"(w2383) -> ()
                          n369 = local write "C-50-N"(w2383) -> ()
                          n370 = local write "C-50-L"(w2383) -> ()
                          n371 = local write "Z-1K-N"(w2383) -> ()
                          n372 = local write "C-1K-L"(w2383) -> ()
                          n373 = local write "Z-1K-L"(w2383) -> ()
                          n374 = local write "Z-100-L"(w2383) -> ()
                          n375 = local write "C-10K-L"(w2383) -> ()
                          n376 = local write "Z-10K-L"(w2383) -> ()
                          n377 = local write "C-10K-N"(w2383) -> ()
                          n378 = local write "Z-10K-N"(w2383) -> ()
                          n379 = local write "C-100-N"(w2383) -> ()
                          n380 = local write "C-100-L"(w2383) -> ()
                          n381 = local write "Z-100-N"(w2383) -> ()
                        }
                      }
                    }
                    n382 = call <vilib>:"Mean.vi"("X"=w1934) -> ("mean"=w1917:dbl)  [unwired: 1 out]
                    n383 = call <vilib>:"Mean.vi"("X"=w1933) -> ("mean"=w1916:dbl)  [unwired: 1 out]
                    n384 = call <vilib>:"Mean.vi"("X"=w1932) -> ("mean"=w1915:dbl)  [unwired: 1 out]
                    n385 = call <vilib>:"Mean.vi"("X"=w1931) -> ("mean"=w1914:dbl)  [unwired: 1 out]
                    n386 = call <vilib>:"Mean.vi"("X"=w1930) -> ("mean"=w1913:dbl)  [unwired: 1 out]
                    n387 = call <vilib>:"Mean.vi"("X"=w1929) -> ("mean"=w1912:dbl)  [unwired: 1 out]
                    n388 = call <vilib>:"Mean.vi"("X"=w1928) -> ("mean"=w1911:dbl)  [unwired: 1 out]
                    n389 = call <vilib>:"Mean.vi"("X"=w1927) -> ("mean"=w1910:dbl)  [unwired: 1 out]
                    n390 = call <vilib>:"Mean.vi"("X"=w1926) -> ("mean"=w1909:dbl)  [unwired: 1 out]
                    n391 = call <vilib>:"Mean.vi"("X"=w1925) -> ("mean"=w1908:dbl)  [unwired: 1 out]
                    n392 = call <vilib>:"Mean.vi"("X"=w1924) -> ("mean"=w1907:dbl)  [unwired: 1 out]
                    n393 = call <vilib>:"Mean.vi"("X"=w1923) -> ("mean"=w1906:dbl)  [unwired: 1 out]
                    n394 = call <vilib>:"Mean.vi"("X"=w1922) -> ("mean"=w1905:dbl)  [unwired: 1 out]
                    n395 = call <vilib>:"Mean.vi"("X"=w1921) -> ("mean"=w1904:dbl)  [unwired: 1 out]
                    n396 = call <vilib>:"Mean.vi"("X"=w1920) -> ("mean"=w1903:dbl)  [unwired: 1 out]
                    n397 = call <vilib>:"Mean.vi"("X"=w1919) -> ("mean"=w1902:dbl)  [unwired: 1 out]
                    n398 = local write "mean"(w1917) -> ()
                    n399 = local write "mean 2"(w1916) -> ()
                    n400 = local write "mean 3"(w1915) -> ()
                    n401 = local write "mean 4"(w1914) -> ()
                    n402 = local write "mean 5"(w1913) -> ()
                    n403 = local write "mean 6"(w1912) -> ()
                    n404 = local write "mean 7"(w1911) -> ()
                    n405 = local write "mean 8"(w1910) -> ()
                    n406 = local write "mean 9"(w1909) -> ()
                    n407 = local write "mean 10"(w1908) -> ()
                    n408 = local write "mean 11"(w1907) -> ()
                    n409 = local write "mean 12"(w1906) -> ()
                    n410 = local write "mean 13"(w1905) -> ()
                    n411 = local write "mean 14"(w1904) -> ()
                    n412 = local write "mean 15"(w1903) -> ()
                    n413 = local write "mean 16"(w1902) -> ()
                  }
                }
              }
              frame #2 {
                n414 = case shown="True" w2385 {
                  tunnel: w2402 -> [_ w2418]
                  tunnel: w2401 -> [_ w2417]
                  tunnel: w2400 -> [_ w2416]
                  tunnel: w2399 -> [_ w2415]
                  tunnel: w2398 -> [_ w2414]
                  tunnel: w2397 -> [_ w2413]
                  tunnel: w2396 -> [_ w2412]
                  tunnel: w2395 -> [_ w2411]
                  tunnel: w2394 -> [_ w2410]
                  tunnel: w2393 -> [_ w2409]
                  tunnel: w2392 -> [_ w2408]
                  tunnel: w2391 -> [_ w2407]
                  tunnel: w2390 -> [_ w2406]
                  tunnel: w2389 -> [_ w2405]
                  tunnel: w2388 -> [_ w2404]
                  tunnel: w2387 -> [_ w2403]
                  frame False {
                  }
                  frame True {
                    w2433 = "\t"
                    w2450 = i16 4 ("precision (6)")
                    n415 = property on="SET" class="DigNum (strict)"() -> ("Value"=w2419:i32)  [unwired: 2 in, 2 out]
                    n416 = Number To Engineering String(2:w2450, 4:w2418) -> (0:w2448:string)  [unwired: 2 in]
                    n417 = Number To Engineering String(2:w2450, 4:w2417) -> (0:w2447:string)  [unwired: 2 in]
                    n418 = Number To Engineering String(2:w2450, 4:w2416) -> (0:w2446:string)  [unwired: 2 in]
                    n419 = Number To Engineering String(2:w2450, 4:w2415) -> (0:w2445:string)  [unwired: 2 in]
                    n420 = Number To Engineering String(2:w2450, 4:w2414) -> (0:w2444:string)  [unwired: 2 in]
                    n421 = Number To Engineering String(2:w2450, 4:w2413) -> (0:w2443:string)  [unwired: 2 in]
                    n422 = Number To Engineering String(2:w2450, 4:w2412) -> (0:w2442:string)  [unwired: 2 in]
                    n423 = Number To Engineering String(2:w2450, 4:w2411) -> (0:w2441:string)  [unwired: 2 in]
                    n424 = Number To Engineering String(2:w2450, 4:w2410) -> (0:w2440:string)  [unwired: 2 in]
                    n425 = Number To Engineering String(2:w2450, 4:w2409) -> (0:w2439:string)  [unwired: 2 in]
                    n426 = Number To Engineering String(2:w2450, 4:w2403) -> (0:w2438:string)  [unwired: 2 in]
                    n427 = Number To Engineering String(2:w2450, 4:w2408) -> (0:w2437:string)  [unwired: 2 in]
                    n428 = Number To Engineering String(2:w2450, 4:w2407) -> (0:w2436:string)  [unwired: 2 in]
                    n429 = Number To Engineering String(2:w2450, 4:w2406) -> (0:w2435:string)  [unwired: 2 in]
                    n430 = Number To Engineering String(2:w2450, 4:w2405) -> (0:w2434:string)  [unwired: 2 in]
                    n431 = Number To Engineering String(2:w2450, 4:w2404) -> (0:w2432:string)  [unwired: 2 in]
                    n432 = Number To Decimal String(number=w2419) -> (decimal integer string=w2449:string)  [unwired: 1 in]
                    n433 = property on="path RLC_mean" class="Path"() -> ("Value"=w2420:path)  [unwired: 2 in, 2 out]
                    n434 = Open/Create/Replace File(file path (use dialog)=w2420, operation (0:open)=T3."open") -> (refnum out=w2425:refnum<file>, error out=w2424:errorcluster)  [unwired: 2 in, 3 out]
                    n435 = Concatenate Strings(w2449, w2433, w2448, w2433, w2447, w2433, w2446, w2433, w2445, w2433, w2444, w2433, w2443, w2433, w2442, w2433, w2441, w2433, w2440, w2433, w2439, w2433, w2438, w2433, w2437, w2433, w2436, w2433, w2435, w2433, w2434, w2433, w2432, "\r\n") -> (w2421:string)
                    n436 = Set File Position(refnum=w2425, from (0:start)=enum16{"start", "end", "current"}."end", error in=w2424) -> (refnum out=w2427:refnum<file>, error out=w2428:errorcluster)  [unwired: 1 in]
                    n437 = Write to Text File(file (use dialog)=w2427, text=w2421, error in=w2428) -> (refnum out=w2423:refnum<file>, error out=w2422:errorcluster)  [unwired: 1 in, 1 out]
                    n438 = Close File(refnum=w2423, error in=w2422) -> (error out=w2430:errorcluster)  [unwired: 1 out]
                    n439 = call <vilib>:"Simple Error Handler.vi"("error in (no error)"=w2430) -> ()  [unwired: 1 in, 8 out]
                  }
                }
              }
            }
            n440 = local write "graph RLC"(w1857) -> ()
          }
        }
        n441 = for {
          N: "N to fit" -> [_]
          tunnel: [w2533] -> w1830 mode=indexing
          tunnel: [w2538] -> w1848 mode=indexing
          tunnel: [w2538] -> w1834 mode=indexing
          tunnel: [w2526] -> w1839 mode=indexing
          i -> [w2538]
          n442 = property on="ON/OFF" class="Bool (strict)"() -> ("Value"=w2517:bool)  [unwired: 2 in, 2 out]
          n443 = property on="Manual Ctrl" class="Bool (strict)"() -> ("Value"=w2520:bool)  [unwired: 2 in, 2 out]
          n444 = property on="Save - Sievert 01" class="Bool (strict)"() -> ("Value"=w2521:bool)  [unwired: 2 in, 2 out]
          n445 = And(x=w2520, y=w2521) -> (x .and. y?=w2519:bool)
          n446 = case shown="True" "Câmara" {
            frame False {
            }
            frame True {
              n447 = property on="Vol Ref" class="Slide (strict)"() -> ("Value"=w2656:dbl)  [unwired: 2 in, 2 out]
              n448 = local write "Camara"(w2656) -> ()
            }
          }
          n449 = case shown="False" "Clear" {
            frame False {
            }
            frame True {
              n450 = property on="P-manual" class="WFChart (strict)"("History Data"=dynamicdata[] []) -> ()  [unwired: 2 in, 2 out]
            }
          }
          n451 = stacked-sequence {
            tunnel: "Entrada Gás" -> [w2687 _ _ _]
            tunnel: "Vácuo" -> [_ w2699 _ _]
            tunnel: "Câmara" -> [_ _ w2711 _]
            tunnel: "ATM" -> [_ _ _ w2723]
            frame #0 {
              w2692 = T4 3 items=["no dialog", "OK message", "continue or stop message", "OK message + warnings", "continue/stop + warnings"] ("type of dialog (OK msg:1)")
              n452 = property on="Entrada gás" class="Bool (strict)"("Value"=w2687) -> ()  [unwired: 2 in, 2 out]
              n453 = call-poly <vilib>:"DAQmx Create Virtual Channel.vi"("lines"=tag "Dev1/port0/line1") -> ("task out"=w2690:refnum<k21>, "error out"=w2691:errorcluster)  [unwired: 13 in]
              n454 = call <vilib>:"DAQmx Start Task.vi"("task/channels in"=w2690, "error in"=w2691) -> ("task out"=w2693:refnum<k21>, "error out"=w2694:errorcluster)  [unwired: 12 in]
              n455 = call-poly <vilib>:"DAQmx Write.vi"("task/channels in"=w2693, "data"=w2687, "error in"=w2694) -> ("task out"=w2698:refnum<k21>, "error out"=w2695:errorcluster)  [unwired: 10 in, 1 out]
              n456 = call <vilib>:"DAQmx Stop Task.vi"("task/channels in"=w2698, "error in"=w2695) -> ("task out"=w2697:refnum<k21>, "error out"=w2696:errorcluster)  [unwired: 12 in]
              n457 = call <vilib>:"DAQmx Clear Task.vi"("task in"=w2697, "error in"=w2696) -> ("error out"=w2689:errorcluster)  [unwired: 13 in]
              n458 = call <vilib>:"Simple Error Handler.vi"("type of dialog (OK msg:1)"=w2692, "error in (no error)"=w2689) -> ()  [unwired: 3 in, 5 out]
            }
            frame #1 {
              w2704 = T4 3 items=["no dialog", "OK message", "continue or stop message", "OK message + warnings", "continue/stop + warnings"] ("type of dialog (OK msg:1)")
              n459 = property on="Vácuo" class="Bool (strict)"("Value"=w2699) -> ()  [unwired: 2 in, 2 out]
              n460 = call-poly <vilib>:"DAQmx Create Virtual Channel.vi"("lines"=tag "Dev1/port0/line2") -> ("task out"=w2702:refnum<k21>, "error out"=w2703:errorcluster)  [unwired: 13 in]
              n461 = call <vilib>:"DAQmx Start Task.vi"("task/channels in"=w2702, "error in"=w2703) -> ("task out"=w2705:refnum<k21>, "error out"=w2706:errorcluster)  [unwired: 12 in]
              n462 = call-poly <vilib>:"DAQmx Write.vi"("task/channels in"=w2705, "data"=w2699, "error in"=w2706) -> ("task out"=w2710:refnum<k21>, "error out"=w2707:errorcluster)  [unwired: 10 in, 1 out]
              n463 = call <vilib>:"DAQmx Stop Task.vi"("task/channels in"=w2710, "error in"=w2707) -> ("task out"=w2709:refnum<k21>, "error out"=w2708:errorcluster)  [unwired: 12 in]
              n464 = call <vilib>:"DAQmx Clear Task.vi"("task in"=w2709, "error in"=w2708) -> ("error out"=w2701:errorcluster)  [unwired: 13 in]
              n465 = call <vilib>:"Simple Error Handler.vi"("type of dialog (OK msg:1)"=w2704, "error in (no error)"=w2701) -> ()  [unwired: 3 in, 5 out]
            }
            frame #2 {
              w2716 = T4 3 items=["no dialog", "OK message", "continue or stop message", "OK message + warnings", "continue/stop + warnings"] ("type of dialog (OK msg:1)")
              n466 = property on="Câmara" class="Bool (strict)"("Value"=w2711) -> ()  [unwired: 2 in, 2 out]
              n467 = call-poly <vilib>:"DAQmx Create Virtual Channel.vi"("lines"=tag "Dev1/port0/line3") -> ("task out"=w2714:refnum<k21>, "error out"=w2715:errorcluster)  [unwired: 13 in]
              n468 = call <vilib>:"DAQmx Start Task.vi"("task/channels in"=w2714, "error in"=w2715) -> ("task out"=w2717:refnum<k21>, "error out"=w2718:errorcluster)  [unwired: 12 in]
              n469 = call-poly <vilib>:"DAQmx Write.vi"("task/channels in"=w2717, "data"=w2711, "error in"=w2718) -> ("task out"=w2722:refnum<k21>, "error out"=w2719:errorcluster)  [unwired: 10 in, 1 out]
              n470 = call <vilib>:"DAQmx Stop Task.vi"("task/channels in"=w2722, "error in"=w2719) -> ("task out"=w2721:refnum<k21>, "error out"=w2720:errorcluster)  [unwired: 12 in]
              n471 = call <vilib>:"DAQmx Clear Task.vi"("task in"=w2721, "error in"=w2720) -> ("error out"=w2713:errorcluster)  [unwired: 13 in]
              n472 = call <vilib>:"Simple Error Handler.vi"("type of dialog (OK msg:1)"=w2716, "error in (no error)"=w2713) -> ()  [unwired: 3 in, 5 out]
            }
            frame #3 {
              w2728 = T4 3 items=["no dialog", "OK message", "continue or stop message", "OK message + warnings", "continue/stop + warnings"] ("type of dialog (OK msg:1)")
              n473 = property on="Atm" class="Bool (strict)"("Value"=w2723) -> ()  [unwired: 2 in, 2 out]
              n474 = call-poly <vilib>:"DAQmx Create Virtual Channel.vi"("lines"=tag "Dev1/port0/line4") -> ("task out"=w2726:refnum<k21>, "error out"=w2727:errorcluster)  [unwired: 13 in]
              n475 = call <vilib>:"DAQmx Start Task.vi"("task/channels in"=w2726, "error in"=w2727) -> ("task out"=w2729:refnum<k21>, "error out"=w2730:errorcluster)  [unwired: 12 in]
              n476 = call-poly <vilib>:"DAQmx Write.vi"("task/channels in"=w2729, "data"=w2723, "error in"=w2730) -> ("task out"=w2734:refnum<k21>, "error out"=w2731:errorcluster)  [unwired: 10 in, 1 out]
              n477 = call <vilib>:"DAQmx Stop Task.vi"("task/channels in"=w2734, "error in"=w2731) -> ("task out"=w2733:refnum<k21>, "error out"=w2732:errorcluster)  [unwired: 12 in]
              n478 = call <vilib>:"DAQmx Clear Task.vi"("task in"=w2733, "error in"=w2732) -> ("error out"=w2725:errorcluster)  [unwired: 13 in]
              n479 = call <vilib>:"Simple Error Handler.vi"("type of dialog (OK msg:1)"=w2728, "error in (no error)"=w2725) -> ()  [unwired: 3 in, 5 out]
            }
          }
          n480 = case shown="True" w2517 {
            frame False {
            }
            frame True {
              n481 = property on="Auto Ctrl" class="Bool (strict)"() -> ("Value"=w2544:bool)  [unwired: 2 in, 2 out]
              n482 = case shown="True" w2544 {
                tunnel: [w2545 w2550] -> w2542
                tunnel: [w2546 w2549] -> w2543
                tunnel: [w2547 w2548] -> w2541
                frame False {
                  n483 = property on="S#01" class="DigNum (strict)"() -> ("Value"=w2547:dbl)  [unwired: 2 in, 2 out]
                  n484 = property on="T fit" class="DigNum (strict)"() -> ("Value"=w2545:dbl)  [unwired: 2 in, 2 out]
                  n485 = property on="termopar K" class="DigNum (strict)"() -> ("Value"=w2546:dbl)  [unwired: 2 in, 2 out]
                }
                frame True {
                  n486 = property on="termopar K 2" class="DigNum (strict)"() -> ("Value"=w2549:dbl)  [unwired: 2 in, 2 out]
                  n487 = property on="S#1_auto" class="DigNum (strict)"() -> ("Value"=w2548:dbl)  [unwired: 2 in, 2 out]
                  n488 = property on="T fit" class="DigNum (strict)"() -> ("Value"=w2550:dbl)  [unwired: 2 in, 2 out]
                }
              }
              n489 = Merge Signals(w2541, w2542, w2543) -> (w2540:dynamicdata)
              n490 = property on="Waveform Chart 2" class="WFChart (strict)"("Value"=w2540) -> ()  [unwired: 2 in, 2 out]
            }
          }
          n491 = case shown="True" "Guardar\nCinetica" {
            frame False {
            }
            frame True {
              n492 = feedback #3() -> (w2609:bool)  [unwired: 1 in]
              "x >= y?" <- w2609
              n493 = call "Elapsed Time"("Reset"=w2609) -> ("Elapsed Time (s)"=w2611:dbl)  [unwired: 11 in, 7 out]
              "Elapsed Time (sec)" <- w2611
              n494 = case shown="True" w2609 {
                frame False {
                }
                frame True {
                  n495 = flat-sequence {
                    tunnel: [w2628] -> w2614
                    tunnel: [w2627] -> w2613
                    tunnel: w2614 -> [w2646]
                    tunnel: w2613 -> [w2645]
                    frame #0 {
                      w2616 = "\t"
                      w2619 = i16 6 ("precision (6)")
                      n496 = property on="P cinetica mean" class="DigNum (strict)"() -> ("Value"=w2625:dbl)  [unwired: 2 in, 2 out]
                      n497 = property on="MEASURE R [Ohm ]" class="DigNum (strict)"() -> ("Value"=w2618:dbl)  [unwired: 2 in, 2 out]
                      n498 = property on="T cinetica mean 2" class="DigNum (strict)"() -> ("Value"=w2624:dbl)  [unwired: 2 in, 2 out]
                      n499 = property on="termopar K" class="DigNum (strict)"() -> ("Value"=w2622:dbl)  [unwired: 2 in, 2 out]
                      n500 = property on="MEASURE C [F ]" class="DigNum (strict)"() -> ("Value"=w2620:dbl)  [unwired: 2 in, 2 out]
                      n501 = property on="path 2_cinetica" class="Path"() -> ("Value"=w2626:path)  [unwired: 2 in, 2 out]
                      n502 = Number To Fractional String(number=w2625, precision (6)=w2619) -> (F-format string=w2640:string)  [unwired: 2 in]
                      n503 = Number To Fractional String(number=w2624, precision (6)=w2619) -> (F-format string=w2639:string)  [unwired: 2 in]
                      n504 = Number To Fractional String(number=w2622, precision (6)=w2619) -> (F-format string=w2623:string)  [unwired: 2 in]
                      n505 = Number To Exponential String(number=w2620, precision (6)=w2619) -> (E-format string=w2621:string)  [unwired: 2 in]
                      n506 = Number To Exponential String(number=w2618, precision (6)=w2619) -> (E-format string=w2617:string)  [unwired: 2 in]
                      n507 = Get Date/Time String(date format (0)=enum16{"short", "long", "abbreviated"}."short", want seconds? (F)=TRUE) -> (date string=w2642:string, time string=w2641:string)  [unwired: 1 in]
                      n508 = Open/Create/Replace File(file path (use dialog)=w2626, operation (0:open)=T3."open") -> (refnum out=w2635:refnum<file>, error out=w2636:errorcluster)  [unwired: 2 in, 3 out]
                      n509 = Concatenate Strings(w2642, w2616, w2641, w2616, w2640, w2616, w2639, w2616, w2623, w2616, w2621, w2616, w2617, w2616, "\r\n") -> (w2629:string)
                      n510 = Set File Position(refnum=w2635, from (0:start)=enum16{"start", "end", "current"}."end", error in=w2636) -> (refnum out=w2633:refnum<file>, error out=w2632:errorcluster)  [unwired: 1 in]
                      n511 = Write to Text File(file (use dialog)=w2633, text=w2629, error in=w2632) -> (refnum out=w2637:refnum<file>, error out=w2638:errorcluster)  [unwired: 2 out]
                      n512 = Close File(refnum=w2637, error in=w2638) -> (path=w2628:path, error out=w2630:errorcluster)
                      n513 = call <vilib>:"Simple Error Handler.vi"("error in (no error)"=w2630) -> ("error out"=w2627:errorcluster)  [unwired: 1 in, 7 out]
                    }
                    frame #1 {
                      n514 = Read from Text File(file (use dialog)=w2646, count=-1 ("Count  3"), error in=w2645) -> (refnum out=w2647:refnum<file>, text=w2651:string, error out=w2648:errorcluster)  [unwired: 1 in, 1 out]
                      n515 = local write "String_cinetica"(w2651) -> ()
                      n516 = Close File(refnum=w2647, error in=w2648) -> (error out=w2649:errorcluster)  [unwired: 1 out]
                      n517 = call <vilib>:"Simple Error Handler.vi"("error in (no error)"=w2649) -> ()  [unwired: 1 in, 8 out]
                    }
                    frame #2 {
                      n518 = local write "P T  index"(0 ("P T  index")) -> ()
                      n519 = local write "T subarray 2"(dbl[] [0.0, 1.0] ("subarray")) -> ()
                      n520 = local write "P subarray"(dbl[] [0.0, 1.0] ("subarray")) -> ()
                    }
                  }
                }
              }
              n521 = Greater Or Equal?(x=w2611, y="seconds") -> (x >= y?=w2612:bool)
              n522 = feedback-in #3(w2612) -> ()
            }
          }
          n523 = property on="S#01" class="DigNum (strict)"() -> ("Value"=w2518:dbl)  [unwired: 2 in, 2 out]
          n524 = case shown="True" w2519 {
            tunnel: w2518 -> [_ w2553]
            frame False {
            }
            frame True {
              n525 = flat-sequence {
                tunnel: w2553 -> [w2596]
                tunnel: [w2595] -> w2552
                frame #0 {
                  n526 = property on="Boolean 4" class="Bool (strict)"() -> ("Value"=w2577:bool)  [unwired: 2 in, 2 out]
                  n527 = case shown="True" w2577 {
                    frame False {
                    }
                    frame True {
                      n528 = local write "PCh1 2"(dbl[] [] ("PCh1")) -> ()
                      n529 = local write "tempo carga 2"(dbl[] [] ("tempo carga")) -> ()
                      n530 = local write "output array 3"(u32[] [] ("output array 2")) -> ()
                    }
                  }
                }
                frame #1 {
                  n531 = Tick Count (ms)() -> (millisecond timer value=w2607:u32)
                  n532 = property on="output array 3" class="Arr (strict)"() -> ("Value"=w2608:u32[])  [unwired: 2 in, 2 out]
                  n533 = Build Array(w2607) -> (w2601:u32[])
                  n534 = Insert Into Array(array=w2608, new element=w2601) -> (w2602:u32[])  [unwired: 1 in]
                  "output array 3" <- w2602
                  n535 = Array Max & Min(array=w2602) -> (max value=w2606:u32, min value=w2605:u32)  [unwired: 2 out]
                  n536 = Subtract(x=w2606, y=w2605) -> (x-y=w2603:u32)
                  n537 = Divide(x=w2603, y=1000.0) -> (x/y=w2594:dbl)
                  n538 = property on="t-sivert01(s)" class="DigNum (strict)"() -> ("Value"=w2582:dbl)  [unwired: 2 in, 2 out]
                  n539 = Build Array(w2596) -> (w2597:dbl[])
                  n540 = Greater?(x=w2594, y=w2582) -> (0:w2595:bool)
                  n541 = Build Array(w2594) -> (w2600:dbl[])
                  n542 = property on="tempo carga 2" class="Arr (strict)"() -> ("Value"=w2599:dbl[])  [unwired: 2 in, 2 out]
                  n543 = property on="PCh1 2" class="Arr (strict)"() -> ("Value"=w2598:dbl[])  [unwired: 2 in, 2 out]
                  n544 = Insert Into Array(array=w2599, new element=w2600) -> (w2587:dbl[])  [unwired: 1 in]
                  "tempo carga 2" <- w2587
                  n545 = Insert Into Array(array=w2598, new element=w2597) -> (w2590:dbl[])  [unwired: 1 in]
                  "PCh1 2" <- w2590
                  n546 = call <vilib>:"General Polynomial Fit.vi"("Y"=w2590, "polynomial order"=0, "X"=w2587) -> ("Best Polynomial Fit"=w2586:dbl[], "Polynomial Coefficients"=w2585:dbl[])  [unwired: 9 in, 2 out]
                  n547 = call <vilib>:"Linear Fit.vi"("Y"=w2590, "X"=w2587) -> ("Best Linear Fit"=w2591:dbl[], "slope"=w2583:dbl)  [unwired: 9 in, 3 out]
                  n548 = local write "dP/dt (bar/s)"(w2583) -> ()
                  n549 = Index Array(array=w2585) -> (element=w2584:dbl)  [unwired: 1 in]
                  n550 = Bundle("Value"=w2587, "Best Polynomial Fit"=w2586) -> (w2588:T5)  [unwired: 1 in]
                  n551 = Bundle("Value"=w2587, "Best Linear Fit"=w2591) -> (w2592:cluster{"Value":dbl[], "Best Linear Fit":dbl[]})  [unwired: 1 in]
                  n552 = Bundle("Value"=w2587, "Value"=w2590) -> (w2593:cluster{"Value":dbl[], "Value":dbl[]})  [unwired: 1 in]
                  n553 = local write "P(bar) FIT"(w2584) -> ()
                  n554 = Build Array(w2593, w2592, w2588) -> (w2581:T6)
                  n555 = property on="XY Graph 2" class="XYGraph (strict)"("Value"=w2581) -> ()  [unwired: 2 in, 2 out]
                }
              }
              n556 = property on="T fit" class="DigNum (strict)"() -> ("Value"=w2551:dbl)  [unwired: 2 in, 2 out]
              n557 = local write "T(º) FIT"(w2551) -> ()
              n558 = local write "Boolean 4"(w2552) -> ()
              n559 = case shown="True" w2552 {
                frame False {
                }
                frame True {
                  w2561 = "\t"
                  w2559 = i16 6 ("precision (6)")
                  n560 = property on="P(bar) FIT" class="DigNum (strict)"() -> ("Value"=w2557:dbl)  [unwired: 2 in, 2 out]
                  n561 = property on="T fit" class="DigNum (strict)"() -> ("Value"=w2555:dbl)  [unwired: 2 in, 2 out]
                  n562 = property on="termopar K" class="DigNum (strict)"() -> ("Value"=w2554:dbl)  [unwired: 2 in, 2 out]
                  n563 = Number To Engineering String(2:w2559, 4:w2557) -> (0:w2563:string)  [unwired: 2 in]
                  n564 = Number To Engineering String(2:w2559, 4:w2555) -> (0:w2562:string)  [unwired: 2 in]
                  n565 = Number To Engineering String(2:w2559, 4:w2554) -> (0:w2560:string)  [unwired: 2 in]
                  n566 = property on="path 2" class="Path"() -> ("Value"=w2556:path)  [unwired: 2 in, 2 out]
                  n567 = Get Date/Time String(date format (0)=enum16{"short", "long", "abbreviated"}."short", want seconds? (F)=TRUE) -> (date string=w2565:string, time string=w2564:string)  [unwired: 1 in]
                  n568 = Open/Create/Replace File(file path (use dialog)=w2556) -> (refnum out=w2573:refnum<file>, error out=w2574:errorcluster)  [unwired: 3 in, 3 out]
                  n569 = Concatenate Strings(w2565, w2561, w2564, w2561, w2563, w2561, w2562, w2561, w2560, "\r\n") -> (w2568:string)
                  n570 = Set File Position(refnum=w2573, from (0:start)=enum16{"start", "end", "current"}."end", error in=w2574) -> (refnum out=w2571:refnum<file>, error out=w2570:errorcluster)  [unwired: 1 in]
                  n571 = Write to Text File(file (use dialog)=w2571, text=w2568, error in=w2570) -> (refnum out=w2575:refnum<file>, error out=w2576:errorcluster)  [unwired: 1 in, 1 out]
                  n572 = Close File(refnum=w2575, error in=w2576) -> (error out=w2569:errorcluster)  [unwired: 1 out]
                  n573 = call <vilib>:"Simple Error Handler.vi"("error in (no error)"=w2569) -> ()  [unwired: 1 in, 8 out]
                }
              }
            }
          }
          n574 = property on="correção NTC" class="DigNum (strict)"() -> ("Value"=w2529:dbl)  [unwired: 2 in, 2 out]
          n575 = call "Read P T.vi"("correção NTC"=w2529) -> ("Sievert01"=w2522:dbl, "mean H2 sensor"=→"mean H2 sensor (V)":dbl, "termopar K"=w2527:dbl, "output NTC"=w2526:dbl, "P Set 2 Output 2"=w2525:dbl)  [unwired: 3 in, 7 out]
          "termopar K" <- w2527
          "output NTC" <- w2526
          n576 = Multiply(x=w2522, y=10.0) -> (x*y=w2523:dbl)
          "S#01" <- w2523
          n577 = Multiply(x=w2525, y=10.0) -> (x*y=w2533:dbl)
          n578 = local write "Vol Ref"(w2533) -> ()
          n579 = Merge Signals(w2533, w2526, w2527, w2523) -> (→"P-manual":dynamicdata)
          n580 = stacked-sequence {
            tunnel: w2533 -> [w2679 _]
            tunnel: w2526 -> [w2658 _]
            frame #0 {
              w2657 = 2 ("y")
              n581 = property on="P subarray" class="Arr (strict)"() -> ("Value"=w2681:dbl[])  [unwired: 2 in, 2 out]
              n582 = property on="P T  index" class="DigNum (strict)"() -> ("Value"=w2659:i32)  [unwired: 2 in, 2 out]
              n583 = property on="T subarray 2" class="Arr (strict)"() -> ("Value"=w2668:dbl[])  [unwired: 2 in, 2 out]
              n584 = Replace Array Subset(array=w2681, new element=w2679, index=w2659) -> (w2677:dbl[])
              n585 = Replace Array Subset(array=w2668, new element=w2658, index=w2659) -> (w2665:dbl[])
              n586 = call-poly <vilib>:"Array To Matrix.vi"("Real 1D Array"=w2677) -> ("Real Matrix (Column Vector)"=w2684:T7)
              n587 = call-poly <vilib>:"Array To Matrix.vi"("Real 1D Array"=w2665) -> ("Real Matrix (Column Vector)"=w2671:T7)
              n588 = Matrix Size(0:w2684) -> (1:w2683:i32, 2:w2682:i32)
              n589 = Matrix Size(0:w2671) -> (1:w2670:i32, 2:w2669:i32)
              n590 = Increment(x=w2683) -> (x+1=w2672:i32)
              n591 = Increment(x=w2670) -> (x+1=w2660:i32)
              n592 = Resize Matrix(1:w2682, 2:w2672, 4:w2684) -> (0:w2680:T7)
              n593 = Resize Matrix(1:w2669, 2:w2660, 4:w2671) -> (0:w2667:T7)
              n594 = call-poly <vilib>:"Matrix To Array.vi"("Real Matrix"=w2680) -> ("Real 2D Array"=w2675:dbl[][])
              n595 = call-poly <vilib>:"Matrix To Array.vi"("Real Matrix"=w2667) -> ("Real 2D Array"=w2663:dbl[][])
              n596 = Subtract(x=w2672, y=w2657) -> (x-y=w2673:i32)
              n597 = Subtract(x=w2660, y=w2657) -> (x-y=w2661:i32)
              n598 = Reshape Array(w2675, w2672) -> (w2674:dbl[])
              n599 = Reshape Array(w2663, w2660) -> (w2662:dbl[])
              n600 = local write "P subarray"(w2674) -> ()
              n601 = Reshape Array(w2674, w2673) -> (w2676:dbl[])
              n602 = local write "T subarray 2"(w2662) -> ()
              n603 = Reshape Array(w2662, w2661) -> (w2664:dbl[])
              n604 = call <vilib>:"Mean.vi"("X"=w2676) -> ("mean"=→"P cinetica mean":dbl)  [unwired: 1 out]
              n605 = call <vilib>:"Mean.vi"("X"=w2664) -> ("mean"=→"T cinetica mean 2":dbl)  [unwired: 1 out]
            }
            frame #1 {
              n606 = property on="P T  index" class="DigNum (strict)"() -> ("Value"=w2686:i32)  [unwired: 2 in, 2 out]
              n607 = Increment(x=w2686) -> (x+1=w2685:i32)
              n608 = local write "P T  index"(w2685) -> ()
            }
          }
          "N" <- w2538
        }
        n609 = call <vilib>:"Linear Fit.vi"("Y"=w1830, "X"=w1834) -> ("Best Linear Fit"=w1832:dbl[], "slope"=→"bar/N":dbl)  [unwired: 9 in, 3 out]
        n610 = Bundle(w1834, w1830) -> (w1837:cluster{i32[], dbl[]})  [unwired: 1 in]
        n611 = call <vilib>:"General Polynomial Fit.vi"("Y"=w1839, "polynomial order"=w1855, "X"=w1834) -> ("Best Polynomial Fit"=w1851:dbl[], "Polynomial Coefficients"=w1852:dbl[])  [unwired: 9 in, 2 out]
        "Polynomial Coefficients 2" <- w1852
        n612 = call <vilib>:"General Polynomial Fit.vi"("Y"=w1830, "polynomial order"=w1855, "X"=w1848) -> ("Best Polynomial Fit"=w1833:dbl[], "Polynomial Coefficients"=w1846:dbl[])  [unwired: 9 in, 2 out]
        "Polynomial Coefficients" <- w1846
        n613 = Bundle(w1834, "Best Polynomial Fit"=w1833) -> (w1836:cluster{i32[], "Best Polynomial Fit":dbl[]})  [unwired: 1 in]
        n614 = Build Array(w1839, w1851) -> (→"Linear Model Graph 2":dbl[][])
        n615 = Index Array(array=w1846, index=0) -> (element=→"p fit":dbl)
        n616 = Index Array(array=w1852, index=0) -> (element=→"T fit":dbl)
        n617 = Build Array(w1830, w1833, w1832) -> (→"Linear Model Graph":dbl[][])
        n618 = Bundle(w1834, "Best Linear Fit"=w1832) -> (w1835:cluster{i32[], "Best Linear Fit":dbl[]})  [unwired: 1 in]
        n619 = Build Array(w1837, w1836, w1835) -> ()  [unwired: 1 out]
      }
    }
    n620 = case shown="True" "Ligar RLC" {
      tunnel: w47 -> [_ w176]
      frame False {
      }
      frame True {
        w184 = "\t"
        w205 = "\t"
        w188 = "\r"
        w181 = "\r\n"
        w221 = "\r"
        w211 = "\t"
        n621 = Strip Path(path=w176) -> (stripped path=w177:path, name=w180:string)
        n622 = Get Date/Time String(date format (0)=enum16{"short", "long", "abbreviated"}."short", want seconds? (F)=TRUE) -> (date string=w228:string, time string=w227:string)  [unwired: 1 in]
        n623 = Concatenate Strings("SET" ("Nota 4"), w184, "DATE" ("Nota 4"), w184, "TIME" ("Nota 4"), w184, w205, "P (BAR)" ("Nota 4"), w205, "T (ºC)" ("Nota 4"), w205, "C-50-L" ("Nota 4"), w205, "C-50-N" ("Nota 4"), w205, "C-100-L" ("Nota 4"), w205, "C-100-N" ("Nota 4"), w205, "C-1K-L" ("Nota 4"), w205, "C-1K-N" ("Nota 4"), w205, "C-10K-L" ("Nota 4"), w205, "C-10K-N" ("Nota 4"), w205, "Z-50-L" ("Nota 4"), w205, "Z-50-N" ("Nota 4"), w205, "Z-100-L" ("Nota 4"), w205, "Z-100-N" ("Nota 4"), w205, "Z-1K-L" ("Nota 4"), w205, "Z-1K-N" ("Nota 4"), w205, "Z-10K-L" ("Nota 4"), w205, "Z-10K-N" ("Nota 4")) -> (w189:string)
        n624 = Concatenate Strings(w228, w211, w227) -> (w223:string)
        n625 = Concatenate Strings(w180, "_RLC_CDH completo" ("string")) -> (w178:string)
        n626 = Concatenate Strings("Sievert RLC - CDH:" ("string"), w211, w181, w181) -> (w209:string)
        n627 = Concatenate Strings("Data Table" ("string"), w188, "==========" ("string"), w188, w189, w188) -> (w222:string)
        n628 = File Dialog(6:".txt" ("pattern label"), 9:w178, 11:w177) -> (0:w219:errorcluster, 3:w220:path)  [unwired: 2 in, 4 out]
        n629 = Open/Create/Replace File(file path (use dialog)=w220, error in=w219, operation (0:open)=T3."replace or create with confirmation", access (0:read/write)=enum16{"read/write", "read-only", "write-only"}."read/write") -> (refnum out=w216:refnum<file>, error out=w215:errorcluster)  [unwired: 3 out]
        n630 = Concatenate Strings(w223, w221, w221, w209, w221, w221, "Nota 01: MEDIDAS COM RLC 300 - MULTILEITURA" ("Nota 4"), w221, w221, w222) -> (w226:string)
        n631 = Write to Text File(file (use dialog)=w216, text=w226, error in=w215) -> (refnum out=w214:refnum<file>, error out=w212:errorcluster)  [unwired: 1 in, 1 out]
        n632 = Close File(refnum=w214, error in=w212) -> (path=w208:path)  [unwired: 1 out]
        n633 = local write "path RLC_completo"(w208) -> ()
      }
    }
    n634 = case shown="True" "Ligar RLC" {
      tunnel: w47 -> [_ w119]
      frame False {
      }
      frame True {
        w128 = "\t"
        w149 = "\t"
        w132 = "\r"
        w125 = "\r\n"
        w164 = "\r"
        w154 = "\t"
        n635 = Strip Path(path=w119) -> (stripped path=w121:path, name=w124:string)
        n636 = Get Date/Time String(date format (0)=enum16{"short", "long", "abbreviated"}."short", want seconds? (F)=TRUE) -> (date string=w171:string, time string=w170:string)  [unwired: 1 in]
        n637 = Concatenate Strings("SET" ("Nota 4"), w128, "DATE" ("Nota 4"), w128, "TIME" ("Nota 4"), w128, w149, "P (BAR)" ("Nota 4"), w149, "T (ºC)" ("Nota 4"), w149, "C-50-L" ("Nota 4"), w149, "C-50-N" ("Nota 4"), w149, "C-100-L" ("Nota 4"), w149, "C-100-N" ("Nota 4"), w149, "C-1K-L" ("Nota 4"), w149, "C-1K-N" ("Nota 4"), w149, "C-10K-L" ("Nota 4"), w149, "C-10K-N" ("Nota 4"), w149, "Z-50-L" ("Nota 4"), w149, "Z-50-N" ("Nota 4"), w149, "Z-100-L" ("Nota 4"), w149, "Z-100-N" ("Nota 4"), w149, "Z-1K-L" ("Nota 4"), w149, "Z-1K-N" ("Nota 4"), w149, "Z-10K-L" ("Nota 4"), w149, "Z-10K-N" ("Nota 4")) -> (w133:string)
        n638 = Concatenate Strings(w171, w154, w170) -> (w166:string)
        n639 = Concatenate Strings(w124, "_RLC_CDH mean" ("string")) -> (w122:string)
        n640 = Concatenate Strings("Sievert RLC - CDH:" ("string"), w154, w125, w125) -> (w152:string)
        n641 = Concatenate Strings("Data Table" ("string"), w132, "==========" ("string"), w132, w133, w132) -> (w165:string)
        n642 = File Dialog(6:".txt" ("pattern label"), 9:w122, 11:w121) -> (0:w162:errorcluster, 3:w163:path)  [unwired: 2 in, 4 out]
        n643 = Open/Create/Replace File(file path (use dialog)=w163, error in=w162, operation (0:open)=T3."replace or create with confirmation", access (0:read/write)=enum16{"read/write", "read-only", "write-only"}."read/write") -> (refnum out=w159:refnum<file>, error out=w158:errorcluster)  [unwired: 3 out]
        n644 = Concatenate Strings(w166, w164, w164, w152, w164, w164, "Nota 01: MEDIDAS COM RLC 300 - MULTILEITURA" ("Nota 4"), w164, w164, w165) -> (w169:string)
        n645 = Write to Text File(file (use dialog)=w159, text=w169, error in=w158) -> (refnum out=w157:refnum<file>, error out=w155:errorcluster)  [unwired: 1 in, 1 out]
        n646 = Close File(refnum=w157, error in=w155) -> (path=w120:path)  [unwired: 1 out]
        n647 = local write "path RLC_mean"(w120) -> ()
      }
    }
    n648 = case shown="False" "Auto Ctrl" {
      tunnel: [TRUE ("Auto Ctrl") FALSE ("Auto Ctrl")] -> w53
      frame False {
      }
      frame True {
      }
    }
    n649 = case shown="True" "Save S#1" {
      frame False {
      }
      frame True {
        n650 = call "File_data_cineticaS1.vi"("Nota 01"="Nota 01", "Sample name"="Sample name 2", "File name"="File name 2") -> ("path"=→"path 2":path)  [unwired: 8 in]
      }
    }
    n651 = Exclusive Or(1:w50, 2:"stop") -> (0:w52:bool)
    n652 = case shown="True" "Close RLC 2" {
      tunnel: w40 -> [_ w174]
      frame False {
      }
      frame True {
        n653 = call "RLC_close.vi"("Path"=w174) -> ("String"=w175:string)  [unwired: 10 in]
        n654 = local write "RLC300 - digimess"(w175) -> ()
      }
    }
    n655 = case shown="True" "Open Button 2" {
      frame False {
      }
      frame True {
        n656 = property on="Sample name" class="Str"() -> ("Value"=w1809:string)  [unwired: 2 in, 2 out]
        n657 = property on="File name" class="Str"() -> ("Value"=w1810:string)  [unwired: 2 in, 2 out]
        n658 = property on="Nota" class="Str"() -> ("Value"=w1808:string)  [unwired: 2 in, 2 out]
        n659 = call "Open file.vi"("Nota 01"=w1808, "Sample name"=w1809, "File name"=w1810) -> ("path open old"=w1807:path)  [unwired: 8 in]
        n660 = local write "path"(w1807) -> ()
      }
    }
    n661 = case shown="True" "Refresh Button 2" {
      frame False {
      }
      frame True {
        n662 = property on="Waveform Chart" class="WFChart (strict)"("History Data"=dynamicdata[] []) -> ()  [unwired: 2 in, 2 out]
      }
    }
    n663 = case shown="True" "Refresh Button 3" {
      frame False {
      }
      frame True {
        n664 = property on="Waveform Chart 2" class="WFChart (strict)"("History Data"=dynamicdata[] []) -> ()  [unwired: 2 in, 2 out]
      }
    }
    n665 = case shown="True" "Open Button" {
      frame False {
      }
      frame True {
        n666 = flat-sequence {
          tunnel: ["Sample name"] -> w1813
          tunnel: ["Nota"] -> w1812
          tunnel: [w1815] -> w1811
          tunnel: w1813 -> [w1828]
          tunnel: w1812 -> [w1827]
          tunnel: w1811 -> [w1822]
          frame #0 {
            n667 = local write "Count SET"(0 ("Count SET")) -> ()
            n668 = local write "Set atual"(0 ("Count  3")) -> ()
            n669 = call "File_data_new.vi"("Nota 01"="Nota", "Sample name"="Sample name", "File name"="File name") -> ("path"=w1815:path)  [unwired: 8 in]
            "path" <- w1815
          }
          frame #1 {
            w1823 = FALSE
            n670 = Strip Path(path=w1822) -> (stripped path=w1821:path, name=w1820:string)
            n671 = local write "Pf2"(w1823) -> ()
            n672 = local write "ZPit"(w1823) -> ()
            n673 = local write "Pit"(w1823) -> ()
            n674 = local write "ZPf2"(w1823) -> ()
            n675 = local write "T"(w1823) -> ()
            n676 = Concatenate Strings(w1820, "_cinetica" ("string")) -> (w1825:string)
            n677 = call "File_data_cinetica.vi"("path in"=w1821, "Nota 01"=w1827, "Sample name"=w1828, "File name"=w1825) -> ("path"=→"path 2_cinetica":path)  [unwired: 7 in]
          }
        }
      }
    }
    n678 = local write "Manual Ctrl"(w53) -> ()
    n679 = case shown="True" "Auto Ctrl" {
      tunnel: w40 -> [_ w237]
      tunnel: "RLC on/off" -> [_ w236]
      tunnel: [_ w235] -> w43
      frame False {
      }
      frame True {
        n680 = local write "P T  index 2"(0 ("P T  index")) -> ()
        n681 = local write "time subarray"(dbl[] [0.0, 1.0] ("subarray")) -> ()
        n682 = for {
          N: "N fit" -> [w265]
          tunnel: w237 -> [w256]
          tunnel: w236 -> [w255]
          tunnel: [w254] -> w235
          i -> [w267]
          w271 = 0 ("polynomial order")
          w262 = 0 ("polynomial order")
          n683 = case shown="True" "clear" {
            frame False {
            }
            frame True {
              n684 = property on="Linear P" class="XYGraph (strict)"("Value"=T2 [] ("Linear P")) -> ()  [unwired: 2 in, 2 out]
              n685 = property on="Linear T" class="XYGraph (strict)"("Value"=T2 [] ("Linear T")) -> ()  [unwired: 2 in, 2 out]
              n686 = property on="Automatico" class="WFChart (strict)"("History Data"=dynamicdata[] []) -> ()  [unwired: 2 in, 2 out]
              n687 = property on="Automatico 2" class="WFChart (strict)"("History Data"=dynamicdata[] []) -> ()  [unwired: 2 in, 2 out]
            }
          }
          n688 = property on="path 2_cinetica" class="Path"() -> ("Value"=w259:path)  [unwired: 2 in, 2 out]
          n689 = Increment(x=w267) -> (x+1=w266:i32)
          n690 = call "Read P T.vi"("correção NTC"="correção NTC") -> ("Sievert01"=w248:dbl, "mean H2 sensor"=w251:dbl, "termopar K"=w246:dbl, "output NTC"=w245:dbl, "P Set 2 Output 2"=w250:dbl)  [unwired: 3 in, 7 out]
          "termopar K 2" <- w246
          "mean H2 sensor" <- w251
          n691 = Equal?(x=w266, y=w265) -> (x = y?=w268:bool)
          "x = y?" <- w268
          n692 = Merge Signals(w251) -> (→"Automatico 2":dynamicdata)
          n693 = Multiply(x=w248, y=10.0) -> (x*y=w244:dbl)
          "S#1_auto" <- w244
          n694 = Multiply(x=w250, y=10.0) -> (x*y=w261:dbl)
          n695 = local write "Vol Ref 3"(w261) -> ()
          n696 = case shown="True" "Save - Sievert 01" {
            tunnel: w244 -> [_ w307]
            frame False {
            }
            frame True {
              n697 = flat-sequence {
                tunnel: w307 -> [w350]
                tunnel: [w348] -> w306
                frame #0 {
                  n698 = property on="Boolean 4" class="Bool (strict)"() -> ("Value"=w331:bool)  [unwired: 2 in, 2 out]
                  n699 = case shown="True" w331 {
                    frame False {
                    }
                    frame True {
                      n700 = local write "PCh1"(dbl[] [] ("PCh1")) -> ()
                      n701 = local write "tempo carga"(dbl[] [] ("tempo carga")) -> ()
                      n702 = local write "output array 2"(u32[] [] ("output array 2")) -> ()
                    }
                  }
                }
                frame #1 {
                  n703 = property on="PCh1" class="Arr (strict)"() -> ("Value"=w352:dbl[])  [unwired: 2 in, 2 out]
                  n704 = Build Array(w350) -> (w351:dbl[])
                  n705 = Tick Count (ms)() -> (millisecond timer value=w361:u32)
                  n706 = Insert Into Array(array=w352, new element=w351) -> (w341:dbl[])  [unwired: 1 in]
                  "PCh1" <- w341
                  n707 = Build Array(w361) -> (w355:u32[])
                  n708 = property on="tempo carga" class="Arr (strict)"() -> ("Value"=w353:dbl[])  [unwired: 2 in, 2 out]
                  n709 = property on="output array 2" class="Arr (strict)"() -> ("Value"=w362:u32[])  [unwired: 2 in, 2 out]
                  n710 = Insert Into Array(array=w362, new element=w355) -> (w356:u32[])  [unwired: 1 in]
                  "output array 2" <- w356
                  n711 = Array Max & Min(array=w356) -> (max value=w360:u32, min value=w359:u32)  [unwired: 2 out]
                  n712 = Subtract(x=w360, y=w359) -> (x-y=w357:u32)
                  n713 = Divide(x=w357, y=1000.0) -> (x/y=w347:dbl)
                  n714 = Greater?(x=w347, y="t-sivert01(s)") -> (0:w348:bool)
                  n715 = Build Array(w347) -> (w354:dbl[])
                  n716 = Insert Into Array(array=w353, new element=w354) -> (w338:dbl[])  [unwired: 1 in]
                  "tempo carga" <- w338
                  n717 = call <vilib>:"General Polynomial Fit.vi"("Y"=w341, "polynomial order"=0, "X"=w338) -> ("Best Polynomial Fit"=w337:dbl[], "Polynomial Coefficients"=w336:dbl[])  [unwired: 9 in, 2 out]
                  n718 = Bundle("Value"=w338, "Value"=w341) -> (w345:cluster{"Value":dbl[], "Value":dbl[]})  [unwired: 1 in]
                  n719 = call <vilib>:"Linear Fit.vi"("Y"=w341, "X"=w338) -> ("Best Linear Fit"=w342:dbl[], "slope"=→"dP/dt (bar/s)":dbl)  [unwired: 9 in, 3 out]
                  n720 = Index Array(array=w336) -> (element=→"P(bar) FIT":dbl)  [unwired: 1 in]
                  n721 = Bundle("Value"=w338, "Best Polynomial Fit"=w337) -> (w339:T5)  [unwired: 1 in]
                  n722 = Bundle("Value"=w338, "Best Linear Fit"=w342) -> (w344:cluster{"Value":dbl[], "Best Linear Fit":dbl[]})  [unwired: 1 in]
                  n723 = Build Array(w345, w344, w339) -> (→"XY Graph 2":T6)
                }
              }
              n724 = property on="T fit" class="DigNum (strict)"() -> ("Value"=→"T(º) FIT":dbl)  [unwired: 2 in, 2 out]
              n725 = case shown="True" w306 {
                frame False {
                }
                frame True {
                  w313 = "\t"
                  w311 = i16 6 ("precision (6)")
                  n726 = property on="T fit" class="DigNum (strict)"() -> ("Value"=w314:dbl)  [unwired: 2 in, 2 out]
                  n727 = property on="path 2" class="Path"() -> ("Value"=w308:path)  [unwired: 2 in, 2 out]
                  n728 = property on="P(bar) FIT" class="DigNum (strict)"() -> ("Value"=w322:dbl)  [unwired: 2 in, 2 out]
                  n729 = Number To Engineering String(2:w311, 4:w322) -> (0:w316:string)  [unwired: 2 in]
                  n730 = Number To Engineering String(2:w311, 4:w314) -> (0:w315:string)  [unwired: 2 in]
                  n731 = Open/Create/Replace File(file path (use dialog)=w308) -> (refnum out=w327:refnum<file>, error out=w328:errorcluster)  [unwired: 3 in, 3 out]
                  n732 = Get Date/Time String(date format (0)=enum16{"short", "long", "abbreviated"}."short", want seconds? (F)=TRUE) -> (date string=w318:string, time string=w317:string)  [unwired: 1 in]
                  n733 = property on="termopar K 2" class="DigNum (strict)"() -> ("Value"=w309:dbl)  [unwired: 2 in, 2 out]
                  n734 = Number To Engineering String(2:w311, 4:w309) -> (0:w312:string)  [unwired: 2 in]
                  n735 = Set File Position(refnum=w327, from (0:start)=enum16{"start", "end", "current"}."end", error in=w328) -> (refnum out=w325:refnum<file>, error out=w324:errorcluster)  [unwired: 1 in]
                  n736 = Concatenate Strings(w318, w313, w317, w313, w316, w313, w315, w313, w312, "\r\n") -> (w321:string)
                  n737 = Write to Text File(file (use dialog)=w325, text=w321, error in=w324) -> (refnum out=w329:refnum<file>, error out=w330:errorcluster)  [unwired: 1 in, 1 out]
                  n738 = Close File(refnum=w329, error in=w330) -> (error out=w323:errorcluster)  [unwired: 1 out]
                  n739 = call <vilib>:"Simple Error Handler.vi"("error in (no error)"=w323) -> ()  [unwired: 1 in, 8 out]
                }
              }
              "Boolean 4" <- w306
            }
          }
          n740 = call "Elapsed Time2"("Reset"=w268) -> ("Elapsed Time (s)"=w282:dbl)  [unwired: 11 in, 7 out]
          "Time (sec)" <- w282
          n741 = Merge Signals(w261, w245, w246, w244) -> (→"Automatico":dynamicdata)
          n742 = stacked-sequence {
            tunnel: w261 -> [w1795 _]
            tunnel: w245 -> [w1781 _]
            tunnel: [w1762 _] -> w280
            tunnel: [w1778 _] -> w279
            tunnel: w282 -> [w1765 _]
            tunnel: [w1763 _] -> w276
            tunnel: [w1761 _] -> w258
            tunnel: [w1760 _] -> w257
            frame #0 {
              w1764 = 2 ("y")
              n743 = property on="P subarray 2" class="Arr (strict)"() -> ("Value"=w1797:dbl[])  [unwired: 2 in, 2 out]
              n744 = property on="T subarray 3" class="Arr (strict)"() -> ("Value"=w1787:dbl[])  [unwired: 2 in, 2 out]
              n745 = property on="time subarray" class="Arr (strict)"() -> ("Value"=w1774:dbl[])  [unwired: 2 in, 2 out]
              n746 = property on="P T  index 2" class="DigNum (strict)"() -> ("Value"=w1766:i32)  [unwired: 2 in, 2 out]
              n747 = Replace Array Subset(array=w1774, new element=w1765, index=w1766) -> (w1767:dbl[])
              n748 = Replace Array Subset(array=w1797, new element=w1795, index=w1766) -> (w1780:dbl[])
              n749 = Replace Array Subset(array=w1787, new element=w1781, index=w1766) -> (w1779:dbl[])
              n750 = call-poly <vilib>:"Array To Matrix.vi"("Real 1D Array"=w1767) -> ("Real Matrix (Column Vector)"=w1777:T7)
              n751 = call-poly <vilib>:"Array To Matrix.vi"("Real 1D Array"=w1780) -> ("Real Matrix (Column Vector)"=w1800:T7)
              n752 = call-poly <vilib>:"Array To Matrix.vi"("Real 1D Array"=w1779) -> ("Real Matrix (Column Vector)"=w1790:T7)
              n753 = Matrix Size(0:w1777) -> (1:w1776:i32, 2:w1775:i32)
              n754 = Matrix Size(0:w1800) -> (1:w1799:i32, 2:w1798:i32)
              n755 = Matrix Size(0:w1790) -> (1:w1789:i32, 2:w1788:i32)
              n756 = Increment(x=w1776) -> (x+1=w1768:i32)
              n757 = Increment(x=w1799) -> (x+1=w1791:i32)
              n758 = Increment(x=w1789) -> (x+1=w1782:i32)
              n759 = Subtract(x=w1768, y=w1764) -> (x-y=w1769:i32)
              n760 = Subtract(x=w1791, y=w1764) -> (x-y=w1792:i32)
              n761 = Subtract(x=w1782, y=w1764) -> (x-y=w1783:i32)
              n762 = Resize Matrix(1:w1775, 2:w1768, 4:w1777) -> (0:w1773:T7)
              n763 = Resize Matrix(1:w1798, 2:w1791, 4:w1800) -> (0:w1796:T7)
              n764 = Resize Matrix(1:w1788, 2:w1782, 4:w1790) -> (0:w1786:T7)
              n765 = call-poly <vilib>:"Matrix To Array.vi"("Real Matrix"=w1773) -> ("Real 2D Array"=w1771:dbl[][])
              n766 = call-poly <vilib>:"Matrix To Array.vi"("Real Matrix"=w1796) -> ("Real 2D Array"=w1794:dbl[][])
              n767 = call-poly <vilib>:"Matrix To Array.vi"("Real Matrix"=w1786) -> ("Real 2D Array"=w1785:dbl[][])
              n768 = Reshape Array(w1771, w1768) -> (w1770:dbl[])
              n769 = Reshape Array(w1794, w1791) -> (w1793:dbl[])
              n770 = Reshape Array(w1785, w1782) -> (w1784:dbl[])
              n771 = local write "time subarray"(w1770) -> ()
              n772 = local write "P subarray 2"(w1793) -> ()
              n773 = local write "T subarray 3"(w1784) -> ()
              n774 = Reshape Array(w1770, w1769) -> (w1763:dbl[])
              n775 = Reshape Array(w1793, w1792) -> (w1762:dbl[])
              n776 = Reshape Array(w1784, w1783) -> (w1778:dbl[])
              n777 = call <vilib>:"Mean.vi"("X"=w1763) -> ("mean"=→"Time cinetica":dbl)  [unwired: 1 out]
              n778 = call <vilib>:"Mean.vi"("X"=w1762) -> ("mean"=w1761:dbl)  [unwired: 1 out]
              "P cinetica mean 2" <- w1761
              n779 = call <vilib>:"Mean.vi"("X"=w1778) -> ("mean"=w1760:dbl)  [unwired: 1 out]
              "T cinetica mean 3" <- w1760
            }
            frame #1 {
              n780 = property on="P T  index 2" class="DigNum (strict)"() -> ("Value"=w1802:i32)  [unwired: 2 in, 2 out]
              n781 = Increment(x=w1802) -> (x+1=w1801:i32)
              n782 = local write "P T  index 2"(w1801) -> ()
            }
          }
          n783 = To Time Stamp(1:w282) -> (0:→"time stamp":timestamp)
          n784 = call <vilib>:"Linear Fit.vi"("Y"=w279, "X"=w276) -> ("Best Linear Fit"=w288:dbl[])  [unwired: 9 in, 4 out]
          n785 = Bundle("Real 2D Array"=w276, "Real 2D Array"=w279) -> (w286:T8)  [unwired: 1 in]
          n786 = Bundle("Real 2D Array"=w276, "Real 2D Array"=w280) -> (w285:T8)  [unwired: 1 in]
          n787 = call <vilib>:"General Polynomial Fit.vi"("Y"=w279, "polynomial order"=w262, "X"=w276) -> ("Best Polynomial Fit"=w277:dbl[], "Polynomial Coefficients"=w272:dbl[])  [unwired: 9 in, 2 out]
          n788 = call <vilib>:"General Polynomial Fit.vi"("Y"=w280, "polynomial order"=w262, "X"=w276) -> ("Best Polynomial Fit"=w278:dbl[], "Polynomial Coefficients"=w273:dbl[])  [unwired: 9 in, 2 out]
          n789 = call <vilib>:"Linear Fit.vi"("Y"=w280, "X"=w276) -> ("Best Linear Fit"=w283:dbl[], "slope"=w263:dbl)  [unwired: 9 in, 3 out]
          "bar/s" <- w263
          n790 = property on="path" class="Path"() -> ("Value"=w260:path)  [unwired: 2 in, 2 out]
          n791 = case shown="True" "Play Button" {
            tunnel: w260 -> [_ w371]
            tunnel: w261 -> [_ w370]
            tunnel: w259 -> [_ w369]
            tunnel: w258 -> [_ w368]
            tunnel: w257 -> [_ w367]
            tunnel: w256 -> [_ w366]
            tunnel: w255 -> [_ w365]
            tunnel: [_ w364] -> w254
            tunnel: w246 -> [_ w363]
            frame False {
            }
            frame True {
              n792 = case shown="8" "Estagio auto" {
                tunnel: w371 -> [_ _ _ w463 _ _ w616 _ w774 _ _ w1601 w1670]
                tunnel: w370 -> [_ w437 _ _ w512 w563 _ _ _ w1519 _ _ _]
                tunnel: w369 -> [_ _ _ _ _ _ _ w658 _ _ _ _ _]
                tunnel: w368 -> [_ _ _ _ _ _ _ w657 _ _ _ _ _]
                tunnel: w367 -> [_ _ _ _ _ _ _ w656 _ _ _ _ _]
                tunnel: w366 -> [_ _ _ _ _ _ _ _ w753 _ _ _ _]
                tunnel: w365 -> [_ _ _ _ _ _ _ _ w770 _ _ _ _]
                tunnel: [_ _ _ _ _ _ _ _ w752 _ _ _ _] -> w364
                tunnel: w363 -> [_ _ _ _ _ _ _ _ _ _ _ w1597 _]
                frame 0, Default {
                  n793 = stacked-sequence {
                    frame #0 {
                      w373 = FALSE ("Pit")
                      n794 = local write "String"("Verificar e fechar todas as valvulas" ("String")) -> ()
                      "ZPf2 2" <- w373
                      "Pf2 2" <- w373
                      "Pit 2" <- w373
                      "ZPit 2" <- w373
                      "T 2" <- w373
                    }
                    frame #1 {
                      w376 = FALSE ("Boolean 4")
                      w381 = T4 3 items=["no dialog", "OK message", "continue or stop message", "OK message + warnings", "continue/stop + warnings"] ("type of dialog (OK msg:1)")
                      n795 = Wait (ms)(milliseconds to wait=u32 500) -> ()  [unwired: 1 out]
                      n796 = local write "Entrada gás 2"(w376) -> ()
                      n797 = call-poly <vilib>:"DAQmx Create Virtual Channel.vi"("lines"=tag "Dev1/port0/line1") -> ("task out"=w379:refnum<k21>, "error out"=w380:errorcluster)  [unwired: 13 in]
                      n798 = call <vilib>:"DAQmx Start Task.vi"("task/channels in"=w379, "error in"=w380) -> ("task out"=w382:refnum<k21>, "error out"=w383:errorcluster)  [unwired: 12 in]
                      n799 = call-poly <vilib>:"DAQmx Write.vi"("task/channels in"=w382, "data"=w376, "error in"=w383) -> ("task out"=w387:refnum<k21>, "error out"=w384:errorcluster)  [unwired: 10 in, 1 out]
                      n800 = call <vilib>:"DAQmx Stop Task.vi"("task/channels in"=w387, "error in"=w384) -> ("task out"=w386:refnum<k21>, "error out"=w385:errorcluster)  [unwired: 12 in]
                      n801 = call <vilib>:"DAQmx Clear Task.vi"("task in"=w386, "error in"=w385) -> ("error out"=w378:errorcluster)  [unwired: 13 in]
                      n802 = call <vilib>:"Simple Error Handler.vi"("type of dialog (OK msg:1)"=w381, "error in (no error)"=w378) -> ()  [unwired: 3 in, 5 out]
                    }
                    frame #2 {
                      w389 = FALSE ("Boolean 4")
                      w394 = T4 3 items=["no dialog", "OK message", "continue or stop message", "OK message + warnings", "continue/stop + warnings"] ("type of dialog (OK msg:1)")
                      n803 = Wait (ms)(milliseconds to wait=u32 500) -> ()  [unwired: 1 out]
                      n804 = local write "Vácuo 2"(w389) -> ()
                      n805 = call-poly <vilib>:"DAQmx Create Virtual Channel.vi"("lines"=tag "Dev1/port0/line2") -> ("task out"=w392:refnum<k21>, "error out"=w393:errorcluster)  [unwired: 13 in]
                      n806 = call <vilib>:"DAQmx Start Task.vi"("task/channels in"=w392, "error in"=w393) -> ("task out"=w395:refnum<k21>, "error out"=w396:errorcluster)  [unwired: 12 in]
                      n807 = call-poly <vilib>:"DAQmx Write.vi"("task/channels in"=w395, "data"=w389, "error in"=w396) -> ("task out"=w400:refnum<k21>, "error out"=w397:errorcluster)  [unwired: 10 in, 1 out]
                      n808 = call <vilib>:"DAQmx Stop Task.vi"("task/channels in"=w400, "error in"=w397) -> ("task out"=w399:refnum<k21>, "error out"=w398:errorcluster)  [unwired: 12 in]
                      n809 = call <vilib>:"DAQmx Clear Task.vi"("task in"=w399, "error in"=w398) -> ("error out"=w391:errorcluster)  [unwired: 13 in]
                      n810 = call <vilib>:"Simple Error Handler.vi"("type of dialog (OK msg:1)"=w394, "error in (no error)"=w391) -> ()  [unwired: 3 in, 5 out]
                    }
                    frame #3 {
                      w402 = FALSE ("Boolean 4")
                      w407 = T4 3 items=["no dialog", "OK message", "continue or stop message", "OK message + warnings", "continue/stop + warnings"] ("type of dialog (OK msg:1)")
                      n811 = Wait (ms)(milliseconds to wait=u32 500) -> ()  [unwired: 1 out]
                      n812 = local write "Câmara 2"(w402) -> ()
                      n813 = call-poly <vilib>:"DAQmx Create Virtual Channel.vi"("lines"=tag "Dev1/port0/line3") -> ("task out"=w405:refnum<k21>, "error out"=w406:errorcluster)  [unwired: 13 in]
                      n814 = call <vilib>:"DAQmx Start Task.vi"("task/channels in"=w405, "error in"=w406) -> ("task out"=w408:refnum<k21>, "error out"=w409:errorcluster)  [unwired: 12 in]
                      n815 = call-poly <vilib>:"DAQmx Write.vi"("task/channels in"=w408, "data"=w402, "error in"=w409) -> ("task out"=w413:refnum<k21>, "error out"=w410:errorcluster)  [unwired: 10 in, 1 out]
                      n816 = call <vilib>:"DAQmx Stop Task.vi"("task/channels in"=w413, "error in"=w410) -> ("task out"=w412:refnum<k21>, "error out"=w411:errorcluster)  [unwired: 12 in]
                      n817 = call <vilib>:"DAQmx Clear Task.vi"("task in"=w412, "error in"=w411) -> ("error out"=w404:errorcluster)  [unwired: 13 in]
                      n818 = call <vilib>:"Simple Error Handler.vi"("type of dialog (OK msg:1)"=w407, "error in (no error)"=w404) -> ()  [unwired: 3 in, 5 out]
                    }
                    frame #4 {
                      w415 = FALSE ("Boolean 4")
                      w420 = T4 3 items=["no dialog", "OK message", "continue or stop message", "OK message + warnings", "continue/stop + warnings"] ("type of dialog (OK msg:1)")
                      n819 = Wait (ms)(milliseconds to wait=u32 500) -> ()  [unwired: 1 out]
                      n820 = local write "Atm 2"(w415) -> ()
                      n821 = call-poly <vilib>:"DAQmx Create Virtual Channel.vi"("lines"=tag "Dev1/port0/line4") -> ("task out"=w418:refnum<k21>, "error out"=w419:errorcluster)  [unwired: 13 in]
                      n822 = call <vilib>:"DAQmx Start Task.vi"("task/channels in"=w418, "error in"=w419) -> ("task out"=w421:refnum<k21>, "error out"=w422:errorcluster)  [unwired: 12 in]
                      n823 = call-poly <vilib>:"DAQmx Write.vi"("task/channels in"=w421, "data"=w415, "error in"=w422) -> ("task out"=w426:refnum<k21>, "error out"=w423:errorcluster)  [unwired: 10 in, 1 out]
                      n824 = call <vilib>:"DAQmx Stop Task.vi"("task/channels in"=w426, "error in"=w423) -> ("task out"=w425:refnum<k21>, "error out"=w424:errorcluster)  [unwired: 12 in]
                      n825 = call <vilib>:"DAQmx Clear Task.vi"("task in"=w425, "error in"=w424) -> ("error out"=w417:errorcluster)  [unwired: 13 in]
                      n826 = call <vilib>:"Simple Error Handler.vi"("type of dialog (OK msg:1)"=w420, "error in (no error)"=w417) -> ()  [unwired: 3 in, 5 out]
                    }
                    frame #5 {
                      n827 = Wait (ms)(milliseconds to wait=u32 500) -> ()  [unwired: 1 out]
                    }
                    frame #6 {
                      n828 = property on="Read ZPit" class="Bool (strict)"() -> ("Value"=w429:bool)  [unwired: 2 in, 2 out]
                      n829 = case shown="False" w429 {
                        frame False {
                          n830 = local write "Estagio auto"(3 ("Estagio auto")) -> ()
                        }
                        frame True {
                          n831 = local write "Estagio auto"(1 ("Estagio auto")) -> ()
                        }
                      }
                      n832 = local write "N fit"("N fit 2") -> ()
                    }
                  }
                }
                frame 1 {
                  n833 = Greater?(x=w437, y=1.0) -> (0:w436:bool)
                  n834 = case shown="True" w436 {
                    tunnel: [FALSE ("Boolean") TRUE ("Boolean")] -> w433
                    frame False {
                      w449 = TRUE ("Boolean")
                      n835 = local write "Vácuo 2"(w449) -> ()
                      n836 = call "Controle_vacuo.vi"("time (s) to wait vacuo"=u32 5, "Boolean"=w449) -> ("Vacuo"=w450:bool)  [unwired: 9 in]
                      n837 = local write "Vácuo 2"(w450) -> ()
                      n838 = local write "String"("Limpar volume referencia" ("String")) -> ()
                    }
                    frame True {
                      n839 = call "Controle_ATM.vi"("seconds to wait"="ATM wait") -> ("String 2"=w454:string, "Atm"=w453:bool)  [unwired: 9 in]
                      n840 = local write "Atm 2"(w453) -> ()
                      n841 = local write "String"(w454) -> ()
                    }
                  }
                  n842 = for {
                    N: 1 -> [_]
                    tunnel: [w439] -> w434
                    tunnel: w433 -> [w439]
                    n843 = Wait (ms)(milliseconds to wait=u32 500 ("x")) -> ()  [unwired: 1 out]
                  }
                  n844 = case shown="True" w434 {
                    frame False {
                      n845 = local write "Estagio auto"(2 ("Estagio auto")) -> ()
                    }
                    frame True {
                      w444 = TRUE ("Boolean")
                      n846 = local write "Estagio auto"(2 ("Estagio auto")) -> ()
                      n847 = local write "Vácuo 2"(w444) -> ()
                      n848 = call "Controle_vacuo.vi"("time (s) to wait vacuo"=u32 5, "Boolean"=w444) -> ("Vacuo"=w445:bool)  [unwired: 9 in]
                      n849 = local write "Vácuo 2"(w445) -> ()
                      n850 = local write "String"("Limpar volume referencia" ("String")) -> ()
                    }
                  }
                }
                frame 2 {
                  n851 = property on="Contador" class="DigNum (strict)"() -> ("Value"=w458:i32)  [unwired: 2 in, 2 out]
                  n852 = local write "String"("Ler ZPit" ("String")) -> ()
                  n853 = Increment(x=w458) -> (x+1=w457:i32)
                  n854 = property on="N fit 2" class="DigNum (strict)"() -> ("Value"=w455:i32)  [unwired: 2 in, 2 out]
                  n855 = Equal?(x=w457, y=w455) -> (x = y?=w456:bool)
                  n856 = case shown="True" w456 {
                    frame False {
                    }
                    frame True {
                      n857 = local write "Estagio auto"(3 ("Estagio auto")) -> ()
                    }
                  }
                }
                frame 3 {
                  w466 = "\t"
                  n858 = property on="SET" class="DigNum (strict)"() -> ("Value"=w462:i32)  [unwired: 2 in, 2 out]
                  n859 = property on="Read ZPit" class="Bool (strict)"() -> ("Value"=w461:bool)  [unwired: 2 in, 2 out]
                  n860 = case shown="False" w461 {
                    tunnel: ["  ==>" w473] -> w467
                    frame False {
                    }
                    frame True {
                      n861 = property on="P fit" class="DigNum (strict)"() -> ("Value"=w472:dbl)  [unwired: 2 in, 2 out]
                      n862 = Number To Fractional String(number=w472, precision (6)=i16 3) -> (F-format string=w473:string)  [unwired: 2 in]
                    }
                  }
                  n863 = Number To Decimal String(number=w462) -> (decimal integer string=w465:string)  [unwired: 1 in]
                  n864 = Concatenate Strings(w465, w466, w467, w466) -> (w464:string)
                  n865 = flat-sequence {
                    tunnel: [w477] -> w469
                    tunnel: [w476] -> w468
                    tunnel: w464 -> [w475]
                    tunnel: w463 -> [w474]
                    tunnel: w469 -> [w493]
                    tunnel: w468 -> [w492]
                    frame #0 {
                      n866 = Open/Create/Replace File(file path (use dialog)=w474, operation (0:open)=T3."open") -> (refnum out=w483:refnum<file>, error out=w484:errorcluster)  [unwired: 2 in, 3 out]
                      n867 = Set File Position(refnum=w483, from (0:start)=enum16{"start", "end", "current"}."end", error in=w484) -> (refnum out=w481:refnum<file>, error out=w480:errorcluster)  [unwired: 1 in]
                      n868 = Write to Text File(file (use dialog)=w481, text=w475, error in=w480) -> (refnum out=w485:refnum<file>, error out=w486:errorcluster)  [unwired: 2 out]
                      n869 = Close File(refnum=w485, error in=w486) -> (path=w477:path, error out=w478:errorcluster)
                      n870 = call <vilib>:"Simple Error Handler.vi"("error in (no error)"=w478) -> ("error out"=w476:errorcluster)  [unwired: 1 in, 7 out]
                    }
                    frame #1 {
                      w487 = 0 ("limpo")
                      n871 = local write "Estagio auto"(4 ("Estagio auto")) -> ()
                      n872 = local write "ZPit 2"(TRUE ("ZPit")) -> ()
                      n873 = Wait (ms)(milliseconds to wait=u32 500) -> ()  [unwired: 1 out]
                      n874 = local write "limpo"(w487) -> ()
                      n875 = Read from Text File(file (use dialog)=w493, count=-1 ("Count  3"), error in=w492) -> (refnum out=w494:refnum<file>, text=w498:string, error out=w495:errorcluster)  [unwired: 1 in, 1 out]
                      n876 = local write "String 3"(w498) -> ()
                      n877 = local write "estagio 5"(w487) -> ()
                      n878 = Close File(refnum=w494, error in=w495) -> (error out=w496:errorcluster)  [unwired: 1 out]
                      n879 = local write "String"("abrir valvula entrada gas" ("String")) -> ()
                      n880 = call <vilib>:"Simple Error Handler.vi"("error in (no error)"=w496) -> ()  [unwired: 1 in, 8 out]
                    }
                    frame #2 {
                      w499 = T4 3 items=["no dialog", "OK message", "continue or stop message", "OK message + warnings", "continue/stop + warnings"] ("type of dialog (OK msg:1)")
                      w505 = TRUE ("Boolean 4")
                      n881 = local write "Entrada gás 2"(w505) -> ()
                      n882 = call-poly <vilib>:"DAQmx Create Virtual Channel.vi"("lines"=tag "Dev1/port0/line1") -> ("task out"=w507:refnum<k21>, "error out"=w508:errorcluster)  [unwired: 13 in]
                      n883 = call <vilib>:"DAQmx Start Task.vi"("task/channels in"=w507, "error in"=w508) -> ("task out"=w509:refnum<k21>, "error out"=w510:errorcluster)  [unwired: 12 in]
                      n884 = call-poly <vilib>:"DAQmx Write.vi"("task/channels in"=w509, "data"=w505, "error in"=w510) -> ("task out"=w502:refnum<k21>, "error out"=w501:errorcluster)  [unwired: 10 in, 1 out]
                      n885 = call <vilib>:"DAQmx Stop Task.vi"("task/channels in"=w502, "error in"=w501) -> ("task out"=w503:refnum<k21>, "error out"=w504:errorcluster)  [unwired: 12 in]
                      n886 = call <vilib>:"DAQmx Clear Task.vi"("task in"=w503, "error in"=w504) -> ("error out"=w500:errorcluster)  [unwired: 13 in]
                      n887 = call <vilib>:"Simple Error Handler.vi"("type of dialog (OK msg:1)"=w499, "error in (no error)"=w500) -> ()  [unwired: 3 in, 5 out]
                    }
                  }
                }
                frame 4 {
                  n888 = Greater Or Equal?(x=w512, y="Set P auto") -> (x >= y?=w513:bool)
                  n889 = case shown="True" w513 {
                    tunnel: "Set P auto" -> [_ w528]
                    frame False {
                      w521 = T4 3 items=["no dialog", "OK message", "continue or stop message", "OK message + warnings", "continue/stop + warnings"] ("type of dialog (OK msg:1)")
                      w527 = TRUE ("data")
                      n890 = local write "Estagio auto"(5 ("Estagio auto")) -> ()
                      n891 = Wait (ms)(milliseconds to wait=u32 500) -> ()  [unwired: 1 out]
                      n892 = local write "Entrada gás 2"(w527) -> ()
                      n893 = call-poly <vilib>:"DAQmx Create Virtual Channel.vi"("lines"=tag "Dev1/port0/line1") -> ("task out"=w518:refnum<k21>, "error out"=w517:errorcluster)  [unwired: 13 in]
                      n894 = call <vilib>:"DAQmx Start Task.vi"("task/channels in"=w518, "error in"=w517) -> ("task out"=w516:refnum<k21>, "error out"=w515:errorcluster)  [unwired: 12 in]
                      n895 = call-poly <vilib>:"DAQmx Write.vi"("task/channels in"=w516, "data"=w527, "error in"=w515) -> ("task out"=w524:refnum<k21>, "error out"=w523:errorcluster)  [unwired: 10 in, 1 out]
                      n896 = call <vilib>:"DAQmx Stop Task.vi"("task/channels in"=w524, "error in"=w523) -> ("task out"=w526:refnum<k21>, "error out"=w525:errorcluster)  [unwired: 12 in]
                      n897 = call <vilib>:"DAQmx Clear Task.vi"("task in"=w526, "error in"=w525) -> ("error out"=w522:errorcluster)  [unwired: 13 in]
                      n898 = call <vilib>:"Simple Error Handler.vi"("type of dialog (OK msg:1)"=w521, "error in (no error)"=w522) -> ()  [unwired: 3 in, 5 out]
                    }
                    frame True {
                      n899 = flat-sequence {
                        tunnel: [w531] -> w529
                        tunnel: w528 -> [w531]
                        tunnel: [w546] -> w530
                        tunnel: w529 -> [w545]
                        tunnel: w530 -> [w560]
                        frame #0 {
                          w537 = T4 3 items=["no dialog", "OK message", "continue or stop message", "OK message + warnings", "continue/stop + warnings"] ("type of dialog (OK msg:1)")
                          w544 = FALSE ("data")
                          n900 = Wait (ms)(milliseconds to wait=u32 500) -> ()  [unwired: 1 out]
                          n901 = local write "Entrada gás 2"(w544) -> ()
                          n902 = call-poly <vilib>:"DAQmx Create Virtual Channel.vi"("lines"=tag "Dev1/port0/line1") -> ("task out"=w535:refnum<k21>, "error out"=w536:errorcluster)  [unwired: 13 in]
                          n903 = call <vilib>:"DAQmx Start Task.vi"("task/channels in"=w535, "error in"=w536) -> ("task out"=w533:refnum<k21>, "error out"=w532:errorcluster)  [unwired: 12 in]
                          n904 = call-poly <vilib>:"DAQmx Write.vi"("task/channels in"=w533, "data"=w544, "error in"=w532) -> ("task out"=w541:refnum<k21>, "error out"=w540:errorcluster)  [unwired: 10 in, 1 out]
                          n905 = call <vilib>:"DAQmx Stop Task.vi"("task/channels in"=w541, "error in"=w540) -> ("task out"=w543:refnum<k21>, "error out"=w542:errorcluster)  [unwired: 12 in]
                          n906 = call <vilib>:"DAQmx Clear Task.vi"("task in"=w543, "error in"=w542) -> ("error out"=w538:errorcluster)  [unwired: 13 in]
                          n907 = call <vilib>:"Simple Error Handler.vi"("type of dialog (OK msg:1)"=w537, "error in (no error)"=w538) -> ()  [unwired: 3 in, 5 out]
                        }
                        frame #1 {
                          n908 = stacked-sequence {
                            tunnel: [_ _ _ w557] -> w546
                            tunnel: w545 -> [_ _ w550 _]
                            frame #0 {
                              n909 = call "Controle_ATM.vi"("seconds to wait"=2.0) -> ("Atm"=w548:bool)  [unwired: 9 in, 1 out]
                              n910 = local write "Atm 2"(w548) -> ()
                            }
                            frame #1 {
                              n911 = Wait (ms)(milliseconds to wait=u32 1000) -> ()  [unwired: 1 out]
                            }
                            frame #2 {
                              n912 = Less Or Equal?(x=w550, y=1.5) -> (x <= y?=w552:bool)
                              n913 = case shown="True" w552 {
                                frame False {
                                n914 = call "Controle_ATM.vi"("seconds to wait"=2.0) -> ()  [unwired: 9 in, 2 out]
                                }
                                frame True {
                                w555 = TRUE ("Vácuo")
                                n915 = local write "Vácuo 2"(w555) -> ()
                                n916 = call "Controle_vacuo.vi"("time (s) to wait vacuo"=3.0, "Boolean"=w555) -> ("Vacuo"=w556:bool)  [unwired: 9 in]
                                n917 = local write "Vácuo 2"(w556) -> ()
                                }
                              }
                            }
                            frame #3 {
                              n918 = property on="limpo" class="DigNum (strict)"() -> ("Value"=w558:i32)  [unwired: 2 in, 2 out]
                              n919 = Wait (ms)(milliseconds to wait=u32 1000) -> ()  [unwired: 1 out]
                              n920 = Increment(x=w558) -> (x+1=w557:i32)
                            }
                          }
                        }
                        frame #2 {
                          "limpo" <- w560
                        }
                      }
                    }
                  }
                }
                frame 5 {
                  n921 = property on="Set P auto" class="DigNum (strict)"() -> ("Value"=w562:dbl)  [unwired: 2 in, 2 out]
                  n922 = Greater Or Equal?(x=w563, y=w562) -> (x >= y?=w561:bool)
                  n923 = case shown="True" w561 {
                    selector: w561 -> [_ w585]
                    frame False {
                      n924 = flat-sequence {
                        tunnel: [w565] -> w564
                        tunnel: w564 -> [w581]
                        frame #0 {
                          w568 = T4 3 items=["no dialog", "OK message", "continue or stop message", "OK message + warnings", "continue/stop + warnings"] ("type of dialog (OK msg:1)")
                          w578 = TRUE ("Boolean 4")
                          n925 = property on="estagio 5" class="DigNum (strict)"() -> ("Value"=w566:i32)  [unwired: 2 in, 2 out]
                          n926 = local write "Entrada gás 2"(w578) -> ()
                          n927 = Increment(x=w566) -> (x+1=w565:i32)
                          n928 = call-poly <vilib>:"DAQmx Create Virtual Channel.vi"("lines"=tag "Dev1/port0/line1") -> ("task out"=w572:refnum<k21>, "error out"=w571:errorcluster)  [unwired: 13 in]
                          n929 = call <vilib>:"DAQmx Start Task.vi"("task/channels in"=w572, "error in"=w571) -> ("task out"=w570:refnum<k21>, "error out"=w569:errorcluster)  [unwired: 12 in]
                          n930 = call-poly <vilib>:"DAQmx Write.vi"("task/channels in"=w570, "data"=w578, "error in"=w569) -> ("task out"=w575:refnum<k21>, "error out"=w574:errorcluster)  [unwired: 10 in, 1 out]
                          n931 = call <vilib>:"DAQmx Stop Task.vi"("task/channels in"=w575, "error in"=w574) -> ("task out"=w576:refnum<k21>, "error out"=w577:errorcluster)  [unwired: 12 in]
                          n932 = call <vilib>:"DAQmx Clear Task.vi"("task in"=w576, "error in"=w577) -> ("error out"=w567:errorcluster)  [unwired: 13 in]
                          n933 = call <vilib>:"Simple Error Handler.vi"("type of dialog (OK msg:1)"=w568, "error in (no error)"=w567) -> ()  [unwired: 3 in, 5 out]
                        }
                        frame #1 {
                          n934 = Less?(x=w581, y=6) -> (x < y?=w579:bool)
                          n935 = case shown="False" w579 {
                            frame False {
                              n936 = local write "Estagio auto"(5 ("Estagio auto")) -> ()
                            }
                            frame True {
                              n937 = local write "Estagio auto"(4 ("Estagio auto")) -> ()
                            }
                          }
                          "estagio 5" <- w581
                        }
                      }
                    }
                    frame True {
                      n938 = flat-sequence {
                        tunnel: w585 -> [w586]
                        tunnel: [w586] -> w584
                        tunnel: w584 -> [w602]
                        frame #0 {
                          w587 = FALSE ("Boolean 4")
                          w592 = T4 3 items=["no dialog", "OK message", "continue or stop message", "OK message + warnings", "continue/stop + warnings"] ("type of dialog (OK msg:1)")
                          n939 = local write "Entrada gás 2"(w587) -> ()
                          n940 = call-poly <vilib>:"DAQmx Create Virtual Channel.vi"("lines"=tag "Dev1/port0/line1") -> ("task out"=w590:refnum<k21>, "error out"=w591:errorcluster)  [unwired: 13 in]
                          n941 = call <vilib>:"DAQmx Start Task.vi"("task/channels in"=w590, "error in"=w591) -> ("task out"=w593:refnum<k21>, "error out"=w594:errorcluster)  [unwired: 12 in]
                          n942 = call-poly <vilib>:"DAQmx Write.vi"("task/channels in"=w593, "data"=w587, "error in"=w594) -> ("task out"=w598:refnum<k21>, "error out"=w595:errorcluster)  [unwired: 10 in, 1 out]
                          n943 = call <vilib>:"DAQmx Stop Task.vi"("task/channels in"=w598, "error in"=w595) -> ("task out"=w597:refnum<k21>, "error out"=w596:errorcluster)  [unwired: 12 in]
                          n944 = call <vilib>:"DAQmx Clear Task.vi"("task in"=w597, "error in"=w596) -> ("error out"=w589:errorcluster)  [unwired: 13 in]
                          n945 = call <vilib>:"Simple Error Handler.vi"("type of dialog (OK msg:1)"=w592, "error in (no error)"=w589) -> ()  [unwired: 3 in, 5 out]
                        }
                        frame #1 {
                          n946 = property on="estagio 5" class="DigNum (strict)"() -> ("Value"=w600:i32)  [unwired: 2 in, 2 out]
                          n947 = Greater?(x=w600, y=5) -> (0:w603:bool)
                          n948 = And(x=w602, y=w603) -> (x .and. y?=w601:bool)
                          n949 = case shown="True" w601 {
                            frame False {
                              n950 = local write "Estagio auto"(4 ("Estagio auto")) -> ()
                              n951 = Wait (ms)(milliseconds to wait=u32 500) -> ()  [unwired: 1 out]
                            }
                            frame True {
                              n952 = property on="Contador" class="DigNum (strict)"() -> ("Value"=w607:i32)  [unwired: 2 in, 2 out]
                              n953 = local write "String"("Ler Pit" ("String")) -> ()
                              n954 = Increment(x=w607) -> (x+1=w609:i32)
                              n955 = property on="N fit 2" class="DigNum (strict)"() -> ("Value"=w606:i32)  [unwired: 2 in, 2 out]
                              n956 = Equal?(x=w609, y=w606) -> (x = y?=w608:bool)
                              n957 = case shown="True" w608 {
                                frame False {
                                }
                                frame True {
                                n958 = local write "Estagio auto"(6 ("Estagio auto")) -> ()
                                }
                              }
                            }
                          }
                        }
                      }
                    }
                  }
                }
                frame 6 {
                  n959 = property on="Contador" class="DigNum (strict)"() -> ("Value"=w613:i32)  [unwired: 2 in, 2 out]
                  n960 = Increment(x=w613) -> (x+1=w615:i32)
                  n961 = property on="N fit 2" class="DigNum (strict)"() -> ("Value"=w612:i32)  [unwired: 2 in, 2 out]
                  n962 = Equal?(x=w615, y=w612) -> (x = y?=w614:bool)
                  n963 = case shown="True" w614 {
                    tunnel: w616 -> [_ w617]
                    frame False {
                    }
                    frame True {
                      n964 = property on="P fit" class="DigNum (strict)"() -> ("Value"=w618:dbl)  [unwired: 2 in, 2 out]
                      n965 = Number To Fractional String(number=w618, precision (6)=i16 3) -> (F-format string=w622:string)  [unwired: 2 in]
                      n966 = Concatenate Strings(w622, "\t") -> (w620:string)
                      n967 = flat-sequence {
                        tunnel: [w628] -> w624
                        tunnel: [w627] -> w623
                        tunnel: w620 -> [w626]
                        tunnel: w617 -> [w625]
                        tunnel: w624 -> [w644]
                        tunnel: w623 -> [w643]
                        frame #0 {
                          n968 = Open/Create/Replace File(file path (use dialog)=w625, operation (0:open)=T3."open") -> (refnum out=w634:refnum<file>, error out=w635:errorcluster)  [unwired: 2 in, 3 out]
                          n969 = Set File Position(refnum=w634, from (0:start)=enum16{"start", "end", "current"}."end", error in=w635) -> (refnum out=w632:refnum<file>, error out=w631:errorcluster)  [unwired: 1 in]
                          n970 = Write to Text File(file (use dialog)=w632, text=w626, error in=w631) -> (refnum out=w636:refnum<file>, error out=w637:errorcluster)  [unwired: 2 out]
                          n971 = Close File(refnum=w636, error in=w637) -> (path=w628:path, error out=w629:errorcluster)
                          n972 = call <vilib>:"Simple Error Handler.vi"("error in (no error)"=w629) -> ("error out"=w627:errorcluster)  [unwired: 1 in, 7 out]
                        }
                        frame #1 {
                          n973 = local write "Estagio auto"(7 ("Estagio auto")) -> ()
                          n974 = local write "teste slope"(0 ("teste slope")) -> ()
                          n975 = local write "Pit 2"(TRUE ("ZPit")) -> ()
                          n976 = Wait (ms)(milliseconds to wait=u32 500) -> ()  [unwired: 1 out]
                          n977 = Read from Text File(file (use dialog)=w644, count=-1 ("Count  3"), error in=w643) -> (refnum out=w645:refnum<file>, text=w649:string, error out=w646:errorcluster)  [unwired: 1 in, 1 out]
                          n978 = local write "String 3"(w649) -> ()
                          n979 = Close File(refnum=w645, error in=w646) -> (error out=w647:errorcluster)  [unwired: 1 out]
                          n980 = call <vilib>:"Simple Error Handler.vi"("error in (no error)"=w647) -> ()  [unwired: 1 in, 8 out]
                          n981 = local write "String"("abrir valvula entrada camara" ("String")) -> ()
                        }
                      }
                    }
                  }
                }
                frame 7 {
                  n982 = flat-sequence {
                    tunnel: w656 -> [w660]
                    tunnel: w657 -> [w661]
                    tunnel: w658 -> [w662]
                    tunnel: [w662] -> w655
                    tunnel: [w661] -> w653
                    tunnel: [w660] -> w651
                    tunnel: w655 -> [w665]
                    tunnel: [w665] -> w654
                    tunnel: w653 -> [w663]
                    tunnel: [w663] -> w652
                    tunnel: w651 -> [w664]
                    tunnel: [w664] -> w650
                    tunnel: w654 -> [_]
                    tunnel: w652 -> [_]
                    tunnel: w650 -> [_]
                    frame #0 {
                      n983 = local write "N fit"("N fit patamar") -> ()
                    }
                    frame #1 {
                      n984 = flat-sequence {
                        tunnel: w665 -> [w670]
                        tunnel: w663 -> [w669]
                        tunnel: w664 -> [w668]
                        frame #0 {
                          (unwired) i16 6 ("precision (6)")
                          w667 = "\t"
                          w687 = i16 4 ("precision (6)")
                          n985 = Number To Fractional String(number=w669, precision (6)=w687) -> (F-format string=w682:string)  [unwired: 2 in]
                          n986 = Number To Fractional String(number=w668, precision (6)=w687) -> (F-format string=w681:string)  [unwired: 2 in]
                          n987 = Open/Create/Replace File(file path (use dialog)=w670, operation (0:open)=T3."open") -> (refnum out=w678:refnum<file>, error out=w671:errorcluster)  [unwired: 2 in, 3 out]
                          n988 = Get Date/Time String(date format (0)=enum16{"short", "long", "abbreviated"}."short", want seconds? (F)=TRUE) -> (date string=w684:string, time string=w683:string)  [unwired: 1 in]
                          n989 = Set File Position(refnum=w678, from (0:start)=enum16{"start", "end", "current"}."end", error in=w671) -> (refnum out=w676:refnum<file>, error out=w675:errorcluster)  [unwired: 1 in]
                          n990 = Concatenate Strings(w684, w667, w683, w667, w682, w667, w681, w667, w667, "\r\n") -> (w672:string)
                          n991 = Write to Text File(file (use dialog)=w676, text=w672, error in=w675) -> (refnum out=w679:refnum<file>, error out=w680:errorcluster)  [unwired: 2 out]
                          n992 = Close File(refnum=w679, error in=w680) -> (error out=w673:errorcluster)  [unwired: 1 out]
                          n993 = call <vilib>:"Simple Error Handler.vi"("error in (no error)"=w673) -> ()  [unwired: 1 in, 8 out]
                        }
                      }
                    }
                    frame #2 {
                      n994 = property on="Contador" class="DigNum (strict)"() -> ("Value"=w696:i32)  [unwired: 2 in, 2 out]
                      n995 = Increment(x=w696) -> (x+1=w695:i32)
                      n996 = property on="N fit patamar" class="DigNum (strict)"() -> ("Value"=w688:i32)  [unwired: 2 in, 2 out]
                      n997 = Equal?(x=w695, y=w688) -> (x = y?=w697:bool)
                      n998 = case shown="True" w697 {
                        tunnel: [FALSE w702] -> w694
                        tunnel: [_ w701] -> w693
                        frame False {
                        }
                        frame True {
                          n999 = property on="P (bar/s)" class="DigNum (strict)"() -> ("Value"=w704:dbl)  [unwired: 2 in, 2 out]
                          n1000 = Absolute Value(x=w704) -> (abs(x)=w703:dbl)
                          n1001 = Less Or Equal?(x=w703, y="STOP (bar/s)") -> (x <= y?=w702:bool)
                          n1002 = case shown="True" w702 {
                            tunnel: [_ w706] -> w701
                            frame False {
                            }
                            frame True {
                              n1003 = property on="teste slope" class="DigNum (strict)"() -> ("Value"=w707:i32)  [unwired: 2 in, 2 out]
                              n1004 = local write "Estagio auto"(7 ("Estagio auto")) -> ()
                              n1005 = Increment(x=w707) -> (x+1=w706:i32)
                              "teste slope" <- w706
                            }
                          }
                        }
                      }
                      n1006 = Greater Or Equal?(x=w693, y="Ntest") -> (x >= y?=w691:bool)
                      n1007 = And(x=w697, y=w691) -> (x .and. y?=w690:bool)
                      n1008 = case shown="True" w690 {
                        frame False {
                        }
                        frame True {
                          n1009 = flat-sequence {
                            frame #0 {
                              n1010 = property on="N fit 2" class="DigNum (strict)"() -> ("Value"=w741:i32)  [unwired: 2 in, 2 out]
                              n1011 = Wait (ms)(milliseconds to wait=u32 500) -> ()  [unwired: 1 out]
                              n1012 = local write "N fit"(w741) -> ()
                            }
                            frame #1 {
                              n1013 = local write "Estagio auto"(8 ("Estagio auto")) -> ()
                            }
                          }
                        }
                      }
                      n1014 = case shown="True" w690 {
                        tunnel: [TRUE ("Boolean") FALSE ("Boolean")] -> w689
                        frame False {
                        }
                        frame True {
                        }
                      }
                      n1015 = case shown="False" w694 {
                        tunnel: w689 -> [_ w725]
                        frame False {
                          w721 = T4 3 items=["no dialog", "OK message", "continue or stop message", "OK message + warnings", "continue/stop + warnings"] ("type of dialog (OK msg:1)")
                          w709 = TRUE ("Boolean")
                          n1016 = local write "Câmara 2"(w709) -> ()
                          n1017 = case shown="True" w709 {
                            frame False {
                            }
                            frame True {
                              n1018 = property on="Vol Ref 3" class="Slide (strict)"() -> ("Value"=w722:dbl)  [unwired: 2 in, 2 out]
                              n1019 = local write "Camara 2"(w722) -> ()
                            }
                          }
                          n1020 = call-poly <vilib>:"DAQmx Create Virtual Channel.vi"("lines"=tag "Dev1/port0/line3") -> ("task out"=w711:refnum<k21>, "error out"=w712:errorcluster)  [unwired: 13 in]
                          n1021 = Wait (ms)(milliseconds to wait="patamar milliseconds to wait") -> ()  [unwired: 1 out]
                          n1022 = call <vilib>:"DAQmx Start Task.vi"("task/channels in"=w711, "error in"=w712) -> ("task out"=w713:refnum<k21>, "error out"=w714:errorcluster)  [unwired: 12 in]
                          n1023 = call-poly <vilib>:"DAQmx Write.vi"("task/channels in"=w713, "data"=w709, "error in"=w714) -> ("task out"=w718:refnum<k21>, "error out"=w719:errorcluster)  [unwired: 10 in, 1 out]
                          n1024 = call <vilib>:"DAQmx Stop Task.vi"("task/channels in"=w718, "error in"=w719) -> ("task out"=w716:refnum<k21>, "error out"=w715:errorcluster)  [unwired: 12 in]
                          n1025 = call <vilib>:"DAQmx Clear Task.vi"("task in"=w716, "error in"=w715) -> ("error out"=w720:errorcluster)  [unwired: 13 in]
                          n1026 = call <vilib>:"Simple Error Handler.vi"("type of dialog (OK msg:1)"=w721, "error in (no error)"=w720) -> ()  [unwired: 3 in, 5 out]
                        }
                        frame True {
                          n1027 = flat-sequence {
                            tunnel: w725 -> [w726]
                            tunnel: [w726] -> w723
                            tunnel: [w727] -> w724
                            tunnel: w723 -> [w727]
                            tunnel: w724 -> [w728]
                            frame #0 {
                            }
                            frame #1 {
                            }
                            frame #2 {
                              w730 = T4 3 items=["no dialog", "OK message", "continue or stop message", "OK message + warnings", "continue/stop + warnings"] ("type of dialog (OK msg:1)")
                              n1028 = local write "Câmara 2"(w728) -> ()
                              n1029 = call-poly <vilib>:"DAQmx Create Virtual Channel.vi"("lines"=tag "Dev1/port0/line3") -> ("task out"=w739:refnum<k21>, "error out"=w738:errorcluster)  [unwired: 13 in]
                              n1030 = call <vilib>:"DAQmx Start Task.vi"("task/channels in"=w739, "error in"=w738) -> ("task out"=w737:refnum<k21>, "error out"=w736:errorcluster)  [unwired: 12 in]
                              n1031 = call-poly <vilib>:"DAQmx Write.vi"("task/channels in"=w737, "data"=w728, "error in"=w736) -> ("task out"=w732:refnum<k21>, "error out"=w731:errorcluster)  [unwired: 10 in, 1 out]
                              n1032 = call <vilib>:"DAQmx Stop Task.vi"("task/channels in"=w732, "error in"=w731) -> ("task out"=w734:refnum<k21>, "error out"=w735:errorcluster)  [unwired: 12 in]
                              n1033 = call <vilib>:"DAQmx Clear Task.vi"("task in"=w734, "error in"=w735) -> ("error out"=w729:errorcluster)  [unwired: 13 in]
                              n1034 = call <vilib>:"Simple Error Handler.vi"("type of dialog (OK msg:1)"=w730, "error in (no error)"=w729) -> ()  [unwired: 3 in, 5 out]
                            }
                            frame #3 {
                              n1035 = Wait (ms)(milliseconds to wait=u32 2000) -> ()  [unwired: 1 out]
                            }
                          }
                        }
                      }
                    }
                  }
                }
                frame 8 {
                  n1036 = property on="Contador" class="DigNum (strict)"() -> ("Value"=w772:i32)  [unwired: 2 in, 2 out]
                  n1037 = Increment(x=w772) -> (x+1=w773:i32)
                  n1038 = property on="N fit 2" class="DigNum (strict)"() -> ("Value"=w746:i32)  [unwired: 2 in, 2 out]
                  n1039 = Equal?(x=w773, y=w746) -> (x = y?=w771:bool)
                  n1040 = case shown="True" w771 {
                    tunnel: w774 -> [_ w1483]
                    frame False {
                    }
                    frame True {
                      n1041 = property on="P fit" class="DigNum (strict)"() -> ("Value"=w1484:dbl)  [unwired: 2 in, 2 out]
                      n1042 = Number To Fractional String(number=w1484, precision (6)=i16 3) -> (F-format string=w1488:string)  [unwired: 2 in]
                      n1043 = Concatenate Strings(w1488, "\t") -> (w1486:string)
                      n1044 = flat-sequence {
                        tunnel: [w1495] -> w1490
                        tunnel: [w1494] -> w1489
                        tunnel: w1486 -> [w1493]
                        tunnel: w1483 -> [w1492]
                        tunnel: w1490 -> [w1510]
                        tunnel: w1489 -> [w1509]
                        frame #0 {
                          n1045 = Wait (ms)(milliseconds to wait=u32 500) -> ()  [unwired: 1 out]
                          n1046 = Open/Create/Replace File(file path (use dialog)=w1492, operation (0:open)=T3."open") -> (refnum out=w1501:refnum<file>, error out=w1502:errorcluster)  [unwired: 2 in, 3 out]
                          n1047 = Set File Position(refnum=w1501, from (0:start)=enum16{"start", "end", "current"}."end", error in=w1502) -> (refnum out=w1499:refnum<file>, error out=w1498:errorcluster)  [unwired: 1 in]
                          n1048 = Write to Text File(file (use dialog)=w1499, text=w1493, error in=w1498) -> (refnum out=w1503:refnum<file>, error out=w1504:errorcluster)  [unwired: 2 out]
                          n1049 = Close File(refnum=w1503, error in=w1504) -> (path=w1495:path, error out=w1496:errorcluster)
                          n1050 = call <vilib>:"Simple Error Handler.vi"("error in (no error)"=w1496) -> ("error out"=w1494:errorcluster)  [unwired: 1 in, 7 out]
                        }
                        frame #1 {
                          n1051 = local write "Estagio auto"(9 ("Estagio auto")) -> ()
                          n1052 = local write "Pf2 2"(TRUE ("ZPit")) -> ()
                          n1053 = Wait (ms)(milliseconds to wait=u32 500) -> ()  [unwired: 1 out]
                          n1054 = Read from Text File(file (use dialog)=w1510, count=-1 ("Count  3"), error in=w1509) -> (refnum out=w1511:refnum<file>, text=w1515:string, error out=w1512:errorcluster)  [unwired: 1 in, 1 out]
                          n1055 = local write "String 3"(w1515) -> ()
                          n1056 = Close File(refnum=w1511, error in=w1512) -> (error out=w1513:errorcluster)  [unwired: 1 out]
                          n1057 = call <vilib>:"Simple Error Handler.vi"("error in (no error)"=w1513) -> ()  [unwired: 1 in, 8 out]
                          n1058 = local write "String"("abrir valvula vacuo" ("String")) -> ()
                        }
                      }
                    }
                  }
                  n1059 = case shown="False" w770 {
                    tunnel: [FALSE ("Save manual") w1482] -> w750
                    tunnel: w771 -> [_ w1482]
                    frame False {
                    }
                    frame True {
                    }
                  }
                  n1060 = flat-sequence {
                    tunnel: w750 -> [w776]
                    tunnel: w753 -> [w777]
                    tunnel: [w777] -> w748
                    tunnel: [w776] -> w747
                    tunnel: [w781] -> w769
                    tunnel: [w783] -> w768
                    tunnel: [w784] -> w767
                    tunnel: [w785] -> w766
                    tunnel: [w786] -> w765
                    tunnel: [w787] -> w764
                    tunnel: [w788] -> w763
                    tunnel: [w789] -> w762
                    tunnel: [w790] -> w761
                    tunnel: [w791] -> w760
                    tunnel: [w792] -> w759
                    tunnel: [w793] -> w758
                    tunnel: [w794] -> w757
                    tunnel: [w795] -> w756
                    tunnel: [w796] -> w755
                    tunnel: [w782] -> w754
                    tunnel: [w780] -> w751
                    tunnel: w748 -> [w798]
                    tunnel: w747 -> [w797]
                    tunnel: [w779] -> w745
                    tunnel: [w778] -> w744
                    tunnel: w769 -> [w1426]
                    tunnel: w768 -> [w1425]
                    tunnel: w767 -> [w1424]
                    tunnel: w766 -> [w1423]
                    tunnel: w765 -> [w1422]
                    tunnel: w764 -> [w1421]
                    tunnel: w763 -> [w1420]
                    tunnel: w762 -> [w1419]
                    tunnel: w761 -> [w1418]
                    tunnel: w760 -> [w1417]
                    tunnel: w759 -> [w1416]
                    tunnel: w758 -> [w1415]
                    tunnel: w757 -> [w1414]
                    tunnel: w756 -> [w1413]
                    tunnel: w755 -> [w1412]
                    tunnel: w754 -> [w1411]
                    tunnel: [w1409] -> w752
                    tunnel: w751 -> [w1409]
                    tunnel: [TRUE ("graph RLC")] -> w749
                    tunnel: w745 -> [w1408]
                    tunnel: w744 -> [w1407]
                    frame #0 {
                      n1061 = local write "graph RLC"(FALSE) -> ()
                    }
                    frame #1 {
                      n1062 = case shown="True" w797 {
                        tunnel: [FALSE w839] -> w780
                        tunnel: w798 -> [_ w821]
                        tunnel: [_ w819] -> w781
                        tunnel: [_ w818] -> w782
                        tunnel: [_ w817] -> w783
                        tunnel: [_ w816] -> w784
                        tunnel: [_ w815] -> w785
                        tunnel: [_ w814] -> w786
                        tunnel: [_ w813] -> w787
                        tunnel: [_ w812] -> w788
                        tunnel: [_ w811] -> w789
                        tunnel: [_ w810] -> w790
                        tunnel: [_ w809] -> w791
                        tunnel: [_ w808] -> w792
                        tunnel: [_ w807] -> w793
                        tunnel: [_ w806] -> w794
                        tunnel: [_ w805] -> w795
                        tunnel: [_ w804] -> w796
                        tunnel: [_ w802] -> w779
                        tunnel: [_ w801] -> w778
                        frame False {
                        }
                        frame True {
                          n1063 = property on="path RLC_completo" class="Path"() -> ("Value"=w820:path)  [unwired: 2 in, 2 out]
                          n1064 = for {
                            N: 5 -> [_]
                            tunnel: TRUE -> [w864]
                            tunnel: FALSE -> [w863]
                            tunnel: [w862] -> w839
                            tunnel: [w861] -> w837 mode=indexing
                            tunnel: [w860] -> w836 mode=indexing
                            tunnel: [w859] -> w835 mode=indexing
                            tunnel: [w858] -> w834 mode=indexing
                            tunnel: [w857] -> w833 mode=indexing
                            tunnel: [w856] -> w832 mode=indexing
                            tunnel: [w855] -> w831 mode=indexing
                            tunnel: [w854] -> w830 mode=indexing
                            tunnel: [w853] -> w829 mode=indexing
                            tunnel: [w852] -> w828 mode=indexing
                            tunnel: [w851] -> w827 mode=indexing
                            tunnel: [w850] -> w826 mode=indexing
                            tunnel: [w849] -> w825 mode=indexing
                            tunnel: [w848] -> w824 mode=indexing
                            tunnel: [w847] -> w823 mode=indexing
                            tunnel: [w846] -> w822 mode=indexing
                            tunnel: w821 -> [w845]
                            tunnel: w820 -> [w844]
                            tunnel: [w843] -> w803 mode=indexing
                            tunnel: [w842] -> w800 mode=indexing
                            n1065 = stacked-sequence {
                              tunnel: w864 -> [_ w891 w925 w957 w989 w1021 w1054 w1086 w1118 w1150 w1182 w1214 w1246 w1278 w1311 w1344 w1376 _]
                              tunnel: w863 -> [w886 _ _ _ _ _ _ _ _ _ _ _ _ _ _ _ _ w1406]
                              tunnel: [_ _ _ _ _ _ _ _ _ _ _ _ _ _ _ _ _ TRUE] -> w862
                              tunnel: [_ w890 _ _ _ _ _ _ _ _ _ _ _ _ _ _ _ _] -> w861
                              tunnel: [_ _ w924 _ _ _ _ _ _ _ _ _ _ _ _ _ _ _] -> w860
                              tunnel: [_ _ _ w956 _ _ _ _ _ _ _ _ _ _ _ _ _ _] -> w859
                              tunnel: [_ _ _ _ w988 _ _ _ _ _ _ _ _ _ _ _ _ _] -> w858
                              tunnel: [_ _ _ _ _ w1020 _ _ _ _ _ _ _ _ _ _ _ _] -> w857
                              tunnel: [_ _ _ _ _ _ w1053 _ _ _ _ _ _ _ _ _ _ _] -> w856
                              tunnel: [_ _ _ _ _ _ _ w1085 _ _ _ _ _ _ _ _ _ _] -> w855
                              tunnel: [_ _ _ _ _ _ _ _ w1117 _ _ _ _ _ _ _ _ _] -> w854
                              tunnel: [_ _ _ _ _ _ _ _ _ w1149 _ _ _ _ _ _ _ _] -> w853
                              tunnel: [_ _ _ _ _ _ _ _ _ _ w1181 _ _ _ _ _ _ _] -> w852
                              tunnel: [_ _ _ _ _ _ _ _ _ _ _ w1213 _ _ _ _ _ _] -> w851
                              tunnel: [_ _ _ _ _ _ _ _ _ _ _ _ w1245 _ _ _ _ _] -> w850
                              tunnel: [_ _ _ _ _ _ _ _ _ _ _ _ _ w1277 _ _ _ _] -> w849
                              tunnel: [_ _ _ _ _ _ _ _ _ _ _ _ _ _ w1310 _ _ _] -> w848
                              tunnel: [_ _ _ _ _ _ _ _ _ _ _ _ _ _ _ w1343 _ _] -> w847
                              tunnel: [_ _ _ _ _ _ _ _ _ _ _ _ _ _ _ _ w1375 _] -> w846
                              tunnel: w845 -> [_ w889 w923 w955 w987 w1019 w1052 w1084 w1116 w1148 w1180 w1212 w1244 w1276 w1309 w1342 w1374 _]
                              tunnel: w844 -> [w865 w888 w922 w954 w986 w1018 w1051 w1083 w1115 w1147 w1179 w1211 w1243 w1275 w1308 w1341 w1373 _]
                              tunnel: [_ _ _ _ _ _ w1049 _ _ _ _ _ _ _ _ _ _ _] -> w843
                              tunnel: [_ _ _ _ _ _ _ _ _ _ _ _ _ _ w1306 _ _ _] -> w842
                              frame #0 {
                                w866 = "\t"
                                n1066 = local write "C-50-L"(w886) -> ()
                                n1067 = local write "C-50-N"(w886) -> ()
                                n1068 = local write "Z-50-L"(w886) -> ()
                                n1069 = local write "C-1K-N"(w886) -> ()
                                n1070 = local write "C-1K-L"(w886) -> ()
                                n1071 = local write "Z-50-N"(w886) -> ()
                                n1072 = local write "Z-1K-N"(w886) -> ()
                                n1073 = local write "Z-1K-L"(w886) -> ()
                                n1074 = local write "C-10K-L"(w886) -> ()
                                n1075 = local write "C-100-N"(w886) -> ()
                                n1076 = local write "C-10K-N"(w886) -> ()
                                n1077 = local write "Z-100-L"(w886) -> ()
                                n1078 = local write "Z-10K-L"(w886) -> ()
                                n1079 = local write "Z-100-N"(w886) -> ()
                                n1080 = local write "Z-10K-N"(w886) -> ()
                                n1081 = local write "C-100-L"(w886) -> ()
                                n1082 = Open/Create/Replace File(file path (use dialog)=w865, operation (0:open)=T3."open") -> (refnum out=w880:refnum<file>, error out=w879:errorcluster)  [unwired: 2 in, 3 out]
                                n1083 = Get Date/Time String(date format (0)=enum16{"short", "long", "abbreviated"}."short", want seconds? (F)=TRUE) -> (date string=w872:string, time string=w871:string)  [unwired: 1 in]
                                n1084 = feedback #4() -> (w870:dbl)  [unwired: 1 in]
                                "SET 2" <- w870
                                n1085 = Set File Position(refnum=w880, from (0:start)=enum16{"start", "end", "current"}."end", error in=w879) -> (refnum out=w882:refnum<file>, error out=w883:errorcluster)  [unwired: 1 in]
                                n1086 = Number To Fractional String(number=w870, precision (6)=i16 2) -> (F-format string=w869:string)  [unwired: 2 in]
                                n1087 = Add(x=w870, y=0.2) -> (x+y=w876:dbl)
                                n1088 = feedback-in #4(w876) -> ()
                                n1089 = Concatenate Strings(w869, w866, w872, w866, w871, w866) -> (w868:string)
                                n1090 = Write to Text File(file (use dialog)=w882, text=w868, error in=w883) -> (refnum out=w878:refnum<file>, error out=w877:errorcluster)  [unwired: 1 in, 1 out]
                                n1091 = Close File(refnum=w878, error in=w877) -> (error out=w885:errorcluster)  [unwired: 1 out]
                                n1092 = call <vilib>:"Simple Error Handler.vi"("error in (no error)"=w885) -> ()  [unwired: 1 in, 8 out]
                              }
                              frame #1 {
                                n1093 = case shown="False" "C50L" {
                                tunnel: w891 -> [_ w918]
                                tunnel: [0.0 ("MEASURE A") w898] -> w890
                                tunnel: w889 -> [_ w897]
                                tunnel: w888 -> [_ w893]
                                frame False {
                                }
                                frame True {
                                w899 = "\t"
                                w917 = i16 4 ("width (-)")
                                n1094 = Open/Create/Replace File(file path (use dialog)=w893, operation (0:open)=T3."open") -> (refnum out=w908:refnum<file>, error out=w907:errorcluster)  [unwired: 2 in, 3 out]
                                n1095 = Multiply(x="Time RLC", y=u32 1000) -> (x*y=w896:u32)
                                n1096 = Wait (ms)(milliseconds to wait=w896) -> ()  [unwired: 1 out]
                                n1097 = Set File Position(refnum=w908, from (0:start)=enum16{"start", "end", "current"}."end", error in=w907) -> (refnum out=w910:refnum<file>, error out=w911:errorcluster)  [unwired: 1 in]
                                n1098 = call "RLC_read.vi"("Path"=w897, "String"="cmd /c rlc_read_cAL.py") -> ("MEASURE A"=w898:dbl, "MEASURE V [V]"=w915:dbl, "concatenated string"=w919:string, "MEASURE B"=w916:dbl, "MEASURE I [A]"=w914:dbl)  [unwired: 1 out]
                                "MEASURE A" <- w898
                                "MEASURE B" <- w916
                                n1099 = Number To Engineering String(2:w917, 4:w914) -> (0:w900:string)  [unwired: 2 in]
                                n1100 = local write "RLC300 - digimess"(w919) -> ()
                                n1101 = Number To Engineering String(2:w917, 4:w915) -> (0:w901:string)  [unwired: 2 in]
                                n1102 = Number To Engineering String(2:w917, 4:w898) -> (0:w903:string)  [unwired: 2 in]
                                n1103 = Number To Engineering String(2:w917, 4:w916) -> (0:w902:string)  [unwired: 2 in]
                                n1104 = Concatenate Strings(w903, w899, w902, w899, w901, w899, w900, w899) -> (w904:string)
                                n1105 = Write to Text File(file (use dialog)=w910, text=w904, error in=w911) -> (refnum out=w906:refnum<file>, error out=w905:errorcluster)  [unwired: 1 in, 1 out]
                                n1106 = Close File(refnum=w906, error in=w905) -> (error out=w913:errorcluster)  [unwired: 1 out]
                                n1107 = call <vilib>:"Simple Error Handler.vi"("error in (no error)"=w913) -> ()  [unwired: 1 in, 8 out]
                                "C-50-L" <- w918
                                }
                                }
                              }
                              frame #2 {
                                n1108 = case shown="False" "C50N" {
                                tunnel: w925 -> [_ w950]
                                tunnel: [0.0 ("MEASURE A") w930] -> w924
                                tunnel: w923 -> [_ w929]
                                tunnel: w922 -> [_ w927]
                                frame False {
                                }
                                frame True {
                                w934 = "\t"
                                w949 = i16 4 ("width (-)")
                                n1109 = property on="Time RLC" class="DigNum (strict)"() -> ("Value"=w928:u32)  [unwired: 2 in, 2 out]
                                n1110 = Wait (ms)(milliseconds to wait=w928) -> ()  [unwired: 1 out]
                                n1111 = Open/Create/Replace File(file path (use dialog)=w927, operation (0:open)=T3."open") -> (refnum out=w943:refnum<file>, error out=w942:errorcluster)  [unwired: 2 in, 3 out]
                                n1112 = Set File Position(refnum=w943, from (0:start)=enum16{"start", "end", "current"}."end", error in=w942) -> (refnum out=w945:refnum<file>, error out=w946:errorcluster)  [unwired: 1 in]
                                n1113 = call "RLC_read.vi"("Path"=w929, "String"="cmd /c rlc_read_cAN.py") -> ("MEASURE A"=w930:dbl, "MEASURE V [V]"=w932:dbl, "concatenated string"=w952:string, "MEASURE B"=w933:dbl, "MEASURE I [A]"=w931:dbl)  [unwired: 1 out]
                                "MEASURE A 2" <- w930
                                "MEASURE B 2" <- w933
                                n1114 = Number To Engineering String(2:w949, 4:w931) -> (0:w935:string)  [unwired: 2 in]
                                n1115 = local write "RLC300 - digimess"(w952) -> ()
                                n1116 = Number To Engineering String(2:w949, 4:w932) -> (0:w936:string)  [unwired: 2 in]
                                n1117 = Number To Engineering String(2:w949, 4:w930) -> (0:w938:string)  [unwired: 2 in]
                                n1118 = Number To Engineering String(2:w949, 4:w933) -> (0:w937:string)  [unwired: 2 in]
                                n1119 = Concatenate Strings(w938, w934, w937, w934, w936, w934, w935, w934) -> (w939:string)
                                n1120 = Write to Text File(file (use dialog)=w945, text=w939, error in=w946) -> (refnum out=w941:refnum<file>, error out=w940:errorcluster)  [unwired: 1 in, 1 out]
                                n1121 = Close File(refnum=w941, error in=w940) -> (error out=w948:errorcluster)  [unwired: 1 out]
                                n1122 = call <vilib>:"Simple Error Handler.vi"("error in (no error)"=w948) -> ()  [unwired: 1 in, 8 out]
                                "C-50-N" <- w950
                                }
                                }
                              }
                              frame #3 {
                                n1123 = case shown="False" "C100L" {
                                tunnel: w957 -> [_ w983]
                                tunnel: [0.0 ("MEASURE A") w962] -> w956
                                tunnel: w955 -> [_ w961]
                                tunnel: w954 -> [_ w959]
                                frame False {
                                }
                                frame True {
                                w966 = "\t"
                                w981 = i16 4 ("width (-)")
                                n1124 = property on="Time RLC" class="DigNum (strict)"() -> ("Value"=w960:u32)  [unwired: 2 in, 2 out]
                                n1125 = Wait (ms)(milliseconds to wait=w960) -> ()  [unwired: 1 out]
                                n1126 = Open/Create/Replace File(file path (use dialog)=w959, operation (0:open)=T3."open") -> (refnum out=w975:refnum<file>, error out=w974:errorcluster)  [unwired: 2 in, 3 out]
                                n1127 = Set File Position(refnum=w975, from (0:start)=enum16{"start", "end", "current"}."end", error in=w974) -> (refnum out=w977:refnum<file>, error out=w978:errorcluster)  [unwired: 1 in]
                                n1128 = call "RLC_read.vi"("Path"=w961, "String"="cmd /c rlc_read_cBL.py") -> ("MEASURE A"=w962:dbl, "MEASURE V [V]"=w964:dbl, "concatenated string"=w984:string, "MEASURE B"=w965:dbl, "MEASURE I [A]"=w963:dbl)  [unwired: 1 out]
                                "MEASURE A 3" <- w962
                                "MEASURE B 3" <- w965
                                n1129 = Number To Engineering String(2:w981, 4:w963) -> (0:w967:string)  [unwired: 2 in]
                                n1130 = local write "RLC300 - digimess"(w984) -> ()
                                n1131 = Number To Engineering String(2:w981, 4:w964) -> (0:w968:string)  [unwired: 2 in]
                                n1132 = Number To Engineering String(2:w981, 4:w962) -> (0:w970:string)  [unwired: 2 in]
                                n1133 = Number To Engineering String(2:w981, 4:w965) -> (0:w969:string)  [unwired: 2 in]
                                n1134 = Concatenate Strings(w970, w966, w969, w966, w968, w966, w967, w966) -> (w971:string)
                                n1135 = Write to Text File(file (use dialog)=w977, text=w971, error in=w978) -> (refnum out=w973:refnum<file>, error out=w972:errorcluster)  [unwired: 1 in, 1 out]
                                n1136 = Close File(refnum=w973, error in=w972) -> (error out=w980:errorcluster)  [unwired: 1 out]
                                n1137 = call <vilib>:"Simple Error Handler.vi"("error in (no error)"=w980) -> ()  [unwired: 1 in, 8 out]
                                "C-100-L" <- w983
                                }
                                }
                              }
                              frame #4 {
                                n1138 = case shown="False" "C100N" {
                                tunnel: w989 -> [_ w1014]
                                tunnel: [0.0 ("MEASURE A") w994] -> w988
                                tunnel: w987 -> [_ w993]
                                tunnel: w986 -> [_ w991]
                                frame False {
                                }
                                frame True {
                                w998 = "\t"
                                w1013 = i16 4 ("width (-)")
                                n1139 = property on="Time RLC" class="DigNum (strict)"() -> ("Value"=w992:u32)  [unwired: 2 in, 2 out]
                                n1140 = Wait (ms)(milliseconds to wait=w992) -> ()  [unwired: 1 out]
                                n1141 = Open/Create/Replace File(file path (use dialog)=w991, operation (0:open)=T3."open") -> (refnum out=w1007:refnum<file>, error out=w1006:errorcluster)  [unwired: 2 in, 3 out]
                                n1142 = Set File Position(refnum=w1007, from (0:start)=enum16{"start", "end", "current"}."end", error in=w1006) -> (refnum out=w1009:refnum<file>, error out=w1010:errorcluster)  [unwired: 1 in]
                                n1143 = call "RLC_read.vi"("Path"=w993, "String"="cmd /c rlc_read_cBN.py") -> ("MEASURE A"=w994:dbl, "MEASURE V [V]"=w996:dbl, "concatenated string"=w1016:string, "MEASURE B"=w997:dbl, "MEASURE I [A]"=w995:dbl)  [unwired: 1 out]
                                "MEASURE A 4" <- w994
                                "MEASURE B 4" <- w997
                                n1144 = Number To Engineering String(2:w1013, 4:w995) -> (0:w999:string)  [unwired: 2 in]
                                n1145 = local write "RLC300 - digimess"(w1016) -> ()
                                n1146 = Number To Engineering String(2:w1013, 4:w996) -> (0:w1000:string)  [unwired: 2 in]
                                n1147 = Number To Engineering String(2:w1013, 4:w994) -> (0:w1002:string)  [unwired: 2 in]
                                n1148 = Number To Engineering String(2:w1013, 4:w997) -> (0:w1001:string)  [unwired: 2 in]
                                n1149 = Concatenate Strings(w1002, w998, w1001, w998, w1000, w998, w999, w998) -> (w1003:string)
                                n1150 = Write to Text File(file (use dialog)=w1009, text=w1003, error in=w1010) -> (refnum out=w1005:refnum<file>, error out=w1004:errorcluster)  [unwired: 1 in, 1 out]
                                n1151 = Close File(refnum=w1005, error in=w1004) -> (error out=w1012:errorcluster)  [unwired: 1 out]
                                n1152 = call <vilib>:"Simple Error Handler.vi"("error in (no error)"=w1012) -> ()  [unwired: 1 in, 8 out]
                                "C-100-N" <- w1014
                                }
                                }
                              }
                              frame #5 {
                                n1153 = case shown="False" "C1KL" {
                                tunnel: w1021 -> [_ w1047]
                                tunnel: [0.0 ("MEASURE A") w1026] -> w1020
                                tunnel: w1019 -> [_ w1025]
                                tunnel: w1018 -> [_ w1023]
                                frame False {
                                }
                                frame True {
                                w1045 = "\t"
                                w1030 = i16 4 ("width (-)")
                                n1154 = property on="Time RLC" class="DigNum (strict)"() -> ("Value"=w1024:u32)  [unwired: 2 in, 2 out]
                                n1155 = Wait (ms)(milliseconds to wait=w1024) -> ()  [unwired: 1 out]
                                n1156 = Open/Create/Replace File(file path (use dialog)=w1023, operation (0:open)=T3."open") -> (refnum out=w1036:refnum<file>, error out=w1037:errorcluster)  [unwired: 2 in, 3 out]
                                n1157 = Set File Position(refnum=w1036, from (0:start)=enum16{"start", "end", "current"}."end", error in=w1037) -> (refnum out=w1034:refnum<file>, error out=w1033:errorcluster)  [unwired: 1 in]
                                n1158 = call "RLC_read.vi"("Path"=w1025, "String"="cmd /c rlc_read_cCL.py") -> ("MEASURE A"=w1026:dbl, "MEASURE V [V]"=w1028:dbl, "concatenated string"=w1048:string, "MEASURE B"=w1029:dbl, "MEASURE I [A]"=w1027:dbl)  [unwired: 1 out]
                                "MEASURE A 5" <- w1026
                                "MEASURE B 5" <- w1029
                                n1159 = Number To Engineering String(2:w1030, 4:w1027) -> (0:w1044:string)  [unwired: 2 in]
                                n1160 = local write "RLC300 - digimess"(w1048) -> ()
                                n1161 = Number To Engineering String(2:w1030, 4:w1028) -> (0:w1043:string)  [unwired: 2 in]
                                n1162 = Number To Engineering String(2:w1030, 4:w1026) -> (0:w1041:string)  [unwired: 2 in]
                                n1163 = Number To Engineering String(2:w1030, 4:w1029) -> (0:w1042:string)  [unwired: 2 in]
                                n1164 = Concatenate Strings(w1041, w1045, w1042, w1045, w1043, w1045, w1044, w1045) -> (w1040:string)
                                n1165 = Write to Text File(file (use dialog)=w1034, text=w1040, error in=w1033) -> (refnum out=w1038:refnum<file>, error out=w1039:errorcluster)  [unwired: 1 in, 1 out]
                                n1166 = Close File(refnum=w1038, error in=w1039) -> (error out=w1031:errorcluster)  [unwired: 1 out]
                                n1167 = call <vilib>:"Simple Error Handler.vi"("error in (no error)"=w1031) -> ()  [unwired: 1 in, 8 out]
                                "C-1K-L" <- w1047
                                }
                                }
                              }
                              frame #6 {
                                n1168 = case shown="True" "C1KN" {
                                tunnel: w1054 -> [_ w1079]
                                tunnel: [w1055 w1060] -> w1053
                                tunnel: w1052 -> [_ w1059]
                                tunnel: w1051 -> [_ w1057]
                                tunnel: [w1055 w1056] -> w1049
                                frame False {
                                w1055 = 0.0 ("MEASURE A")
                                }
                                frame True {
                                w1078 = "\t"
                                w1063 = i16 6 ("width (-)")
                                n1169 = property on="Time RLC" class="DigNum (strict)"() -> ("Value"=w1058:u32)  [unwired: 2 in, 2 out]
                                n1170 = Wait (ms)(milliseconds to wait=w1058) -> ()  [unwired: 1 out]
                                n1171 = Open/Create/Replace File(file path (use dialog)=w1057, operation (0:open)=T3."open") -> (refnum out=w1069:refnum<file>, error out=w1070:errorcluster)  [unwired: 2 in, 3 out]
                                n1172 = Set File Position(refnum=w1069, from (0:start)=enum16{"start", "end", "current"}."end", error in=w1070) -> (refnum out=w1067:refnum<file>, error out=w1066:errorcluster)  [unwired: 1 in]
                                n1173 = call "RLC_read.vi"("Path"=w1059, "String"="cmd /c rlc_read_cCN.py") -> ("MEASURE A"=w1060:dbl, "MEASURE V [V]"=w1062:dbl, "concatenated string"=w1081:string, "MEASURE B"=w1056:dbl, "MEASURE I [A]"=w1061:dbl)  [unwired: 1 out]
                                "MEASURE A 6" <- w1060
                                "MEASURE B 6" <- w1056
                                n1174 = Number To Engineering String(2:w1063, 4:w1061) -> (0:w1077:string)  [unwired: 2 in]
                                n1175 = local write "RLC300 - digimess"(w1081) -> ()
                                n1176 = Number To Engineering String(2:w1063, 4:w1062) -> (0:w1076:string)  [unwired: 2 in]
                                n1177 = Number To Engineering String(2:w1063, 4:w1060) -> (0:w1074:string)  [unwired: 2 in]
                                n1178 = Number To Engineering String(2:w1063, 4:w1056) -> (0:w1075:string)  [unwired: 2 in]
                                n1179 = Concatenate Strings(w1074, w1078, w1075, w1078, w1076, w1078, w1077, w1078) -> (w1073:string)
                                n1180 = Write to Text File(file (use dialog)=w1067, text=w1073, error in=w1066) -> (refnum out=w1071:refnum<file>, error out=w1072:errorcluster)  [unwired: 1 in, 1 out]
                                n1181 = Close File(refnum=w1071, error in=w1072) -> (error out=w1064:errorcluster)  [unwired: 1 out]
                                n1182 = call <vilib>:"Simple Error Handler.vi"("error in (no error)"=w1064) -> ()  [unwired: 1 in, 8 out]
                                "C-1K-N" <- w1079
                                }
                                }
                              }
                              frame #7 {
                                n1183 = case shown="True" "C10KL" {
                                tunnel: w1086 -> [_ w1112]
                                tunnel: [0.0 ("MEASURE A") w1091] -> w1085
                                tunnel: w1084 -> [_ w1090]
                                tunnel: w1083 -> [_ w1088]
                                frame False {
                                }
                                frame True {
                                w1095 = "\t"
                                w1110 = i16 4 ("width (-)")
                                n1184 = property on="Time RLC" class="DigNum (strict)"() -> ("Value"=w1089:u32)  [unwired: 2 in, 2 out]
                                n1185 = Wait (ms)(milliseconds to wait=w1089) -> ()  [unwired: 1 out]
                                n1186 = Open/Create/Replace File(file path (use dialog)=w1088, operation (0:open)=T3."open") -> (refnum out=w1104:refnum<file>, error out=w1103:errorcluster)  [unwired: 2 in, 3 out]
                                n1187 = Set File Position(refnum=w1104, from (0:start)=enum16{"start", "end", "current"}."end", error in=w1103) -> (refnum out=w1106:refnum<file>, error out=w1107:errorcluster)  [unwired: 1 in]
                                n1188 = call "RLC_read.vi"("Path"=w1090, "String"="cmd /c rlc_read_cDL.py") -> ("MEASURE A"=w1091:dbl, "MEASURE V [V]"=w1093:dbl, "concatenated string"=w1113:string, "MEASURE B"=w1094:dbl, "MEASURE I [A]"=w1092:dbl)  [unwired: 1 out]
                                "MEASURE A 7" <- w1091
                                "MEASURE B 7" <- w1094
                                n1189 = Number To Engineering String(2:w1110, 4:w1092) -> (0:w1096:string)  [unwired: 2 in]
                                n1190 = local write "RLC300 - digimess"(w1113) -> ()
                                n1191 = Number To Engineering String(2:w1110, 4:w1093) -> (0:w1097:string)  [unwired: 2 in]
                                n1192 = Number To Engineering String(2:w1110, 4:w1091) -> (0:w1099:string)  [unwired: 2 in]
                                n1193 = Number To Engineering String(2:w1110, 4:w1094) -> (0:w1098:string)  [unwired: 2 in]
                                n1194 = Concatenate Strings(w1099, w1095, w1098, w1095, w1097, w1095, w1096, w1095) -> (w1100:string)
                                n1195 = Write to Text File(file (use dialog)=w1106, text=w1100, error in=w1107) -> (refnum out=w1102:refnum<file>, error out=w1101:errorcluster)  [unwired: 1 in, 1 out]
                                n1196 = Close File(refnum=w1102, error in=w1101) -> (error out=w1109:errorcluster)  [unwired: 1 out]
                                n1197 = call <vilib>:"Simple Error Handler.vi"("error in (no error)"=w1109) -> ()  [unwired: 1 in, 8 out]
                                "C-10K-L" <- w1112
                                }
                                }
                              }
                              frame #8 {
                                n1198 = case shown="False" "C10KN" {
                                tunnel: w1118 -> [_ w1144]
                                tunnel: [0.0 ("MEASURE A") w1123] -> w1117
                                tunnel: w1116 -> [_ w1122]
                                tunnel: w1115 -> [_ w1120]
                                frame False {
                                }
                                frame True {
                                w1127 = "\t"
                                w1142 = i16 4 ("width (-)")
                                n1199 = property on="Time RLC" class="DigNum (strict)"() -> ("Value"=w1121:u32)  [unwired: 2 in, 2 out]
                                n1200 = Wait (ms)(milliseconds to wait=w1121) -> ()  [unwired: 1 out]
                                n1201 = Open/Create/Replace File(file path (use dialog)=w1120, operation (0:open)=T3."open") -> (refnum out=w1136:refnum<file>, error out=w1135:errorcluster)  [unwired: 2 in, 3 out]
                                n1202 = Set File Position(refnum=w1136, from (0:start)=enum16{"start", "end", "current"}."end", error in=w1135) -> (refnum out=w1138:refnum<file>, error out=w1139:errorcluster)  [unwired: 1 in]
                                n1203 = call "RLC_read.vi"("Path"=w1122, "String"="cmd /c rlc_read_cDN.py") -> ("MEASURE A"=w1123:dbl, "MEASURE V [V]"=w1125:dbl, "concatenated string"=w1145:string, "MEASURE B"=w1126:dbl, "MEASURE I [A]"=w1124:dbl)  [unwired: 1 out]
                                "MEASURE A 8" <- w1123
                                "MEASURE B 8" <- w1126
                                n1204 = Number To Engineering String(2:w1142, 4:w1124) -> (0:w1128:string)  [unwired: 2 in]
                                n1205 = local write "RLC300 - digimess"(w1145) -> ()
                                n1206 = Number To Engineering String(2:w1142, 4:w1125) -> (0:w1129:string)  [unwired: 2 in]
                                n1207 = Number To Engineering String(2:w1142, 4:w1123) -> (0:w1131:string)  [unwired: 2 in]
                                n1208 = Number To Engineering String(2:w1142, 4:w1126) -> (0:w1130:string)  [unwired: 2 in]
                                n1209 = Concatenate Strings(w1131, w1127, w1130, w1127, w1129, w1127, w1128, w1127) -> (w1132:string)
                                n1210 = Write to Text File(file (use dialog)=w1138, text=w1132, error in=w1139) -> (refnum out=w1134:refnum<file>, error out=w1133:errorcluster)  [unwired: 1 in, 1 out]
                                n1211 = Close File(refnum=w1134, error in=w1133) -> (error out=w1141:errorcluster)  [unwired: 1 out]
                                n1212 = call <vilib>:"Simple Error Handler.vi"("error in (no error)"=w1141) -> ()  [unwired: 1 in, 8 out]
                                "C-10K-N" <- w1144
                                }
                                }
                              }
                              frame #9 {
                                n1213 = case shown="False" "Z50L" {
                                tunnel: w1150 -> [_ w1175]
                                tunnel: [0.0 ("MEASURE A") w1155] -> w1149
                                tunnel: w1148 -> [_ w1154]
                                tunnel: w1147 -> [_ w1152]
                                frame False {
                                }
                                frame True {
                                w1159 = "\t"
                                w1174 = i16 4 ("width (-)")
                                n1214 = property on="Time RLC" class="DigNum (strict)"() -> ("Value"=w1153:u32)  [unwired: 2 in, 2 out]
                                n1215 = Wait (ms)(milliseconds to wait=w1153) -> ()  [unwired: 1 out]
                                n1216 = Open/Create/Replace File(file path (use dialog)=w1152, operation (0:open)=T3."open") -> (refnum out=w1168:refnum<file>, error out=w1167:errorcluster)  [unwired: 2 in, 3 out]
                                n1217 = Set File Position(refnum=w1168, from (0:start)=enum16{"start", "end", "current"}."end", error in=w1167) -> (refnum out=w1170:refnum<file>, error out=w1171:errorcluster)  [unwired: 1 in]
                                n1218 = call "RLC_read.vi"("Path"=w1154, "String"="cmd /c rlc_read_ZAL.py") -> ("MEASURE A"=w1155:dbl, "MEASURE V [V]"=w1157:dbl, "concatenated string"=w1176:string, "MEASURE B"=w1158:dbl, "MEASURE I [A]"=w1156:dbl)  [unwired: 1 out]
                                "MEASURE A 9" <- w1155
                                "MEASURE B 9" <- w1158
                                n1219 = Number To Engineering String(2:w1174, 4:w1156) -> (0:w1160:string)  [unwired: 2 in]
                                n1220 = local write "RLC300 - digimess"(w1176) -> ()
                                n1221 = Number To Engineering String(2:w1174, 4:w1157) -> (0:w1161:string)  [unwired: 2 in]
                                n1222 = Number To Engineering String(2:w1174, 4:w1155) -> (0:w1163:string)  [unwired: 2 in]
                                n1223 = Number To Engineering String(2:w1174, 4:w1158) -> (0:w1162:string)  [unwired: 2 in]
                                n1224 = Concatenate Strings(w1163, w1159, w1162, w1159, w1161, w1159, w1160, w1159) -> (w1164:string)
                                n1225 = Write to Text File(file (use dialog)=w1170, text=w1164, error in=w1171) -> (refnum out=w1166:refnum<file>, error out=w1165:errorcluster)  [unwired: 1 in, 1 out]
                                n1226 = Close File(refnum=w1166, error in=w1165) -> (error out=w1173:errorcluster)  [unwired: 1 out]
                                n1227 = call <vilib>:"Simple Error Handler.vi"("error in (no error)"=w1173) -> ()  [unwired: 1 in, 8 out]
                                "Z-50-L" <- w1175
                                }
                                }
                              }
                              frame #10 {
                                n1228 = case shown="False" "Z50N" {
                                tunnel: w1182 -> [_ w1207]
                                tunnel: [0.0 ("MEASURE A") w1187] -> w1181
                                tunnel: w1180 -> [_ w1186]
                                tunnel: w1179 -> [_ w1184]
                                frame False {
                                }
                                frame True {
                                w1191 = "\t"
                                w1206 = i16 4 ("width (-)")
                                n1229 = property on="Time RLC" class="DigNum (strict)"() -> ("Value"=w1185:u32)  [unwired: 2 in, 2 out]
                                n1230 = Wait (ms)(milliseconds to wait=w1185) -> ()  [unwired: 1 out]
                                n1231 = Open/Create/Replace File(file path (use dialog)=w1184, operation (0:open)=T3."open") -> (refnum out=w1200:refnum<file>, error out=w1199:errorcluster)  [unwired: 2 in, 3 out]
                                n1232 = Set File Position(refnum=w1200, from (0:start)=enum16{"start", "end", "current"}."end", error in=w1199) -> (refnum out=w1202:refnum<file>, error out=w1203:errorcluster)  [unwired: 1 in]
                                n1233 = call "RLC_read.vi"("Path"=w1186, "String"="cmd /c rlc_read_ZAN.py") -> ("MEASURE A"=w1187:dbl, "MEASURE V [V]"=w1189:dbl, "concatenated string"=w1208:string, "MEASURE B"=w1190:dbl, "MEASURE I [A]"=w1188:dbl)  [unwired: 1 out]
                                "MEASURE A 10" <- w1187
                                "MEASURE B 10" <- w1190
                                n1234 = Number To Engineering String(2:w1206, 4:w1188) -> (0:w1192:string)  [unwired: 2 in]
                                n1235 = local write "RLC300 - digimess"(w1208) -> ()
                                n1236 = Number To Engineering String(2:w1206, 4:w1189) -> (0:w1193:string)  [unwired: 2 in]
                                n1237 = Number To Engineering String(2:w1206, 4:w1187) -> (0:w1195:string)  [unwired: 2 in]
                                n1238 = Number To Engineering String(2:w1206, 4:w1190) -> (0:w1194:string)  [unwired: 2 in]
                                n1239 = Concatenate Strings(w1195, w1191, w1194, w1191, w1193, w1191, w1192, w1191) -> (w1196:string)
                                n1240 = Write to Text File(file (use dialog)=w1202, text=w1196, error in=w1203) -> (refnum out=w1198:refnum<file>, error out=w1197:errorcluster)  [unwired: 1 in, 1 out]
                                n1241 = Close File(refnum=w1198, error in=w1197) -> (error out=w1205:errorcluster)  [unwired: 1 out]
                                n1242 = call <vilib>:"Simple Error Handler.vi"("error in (no error)"=w1205) -> ()  [unwired: 1 in, 8 out]
                                "Z-50-N" <- w1207
                                }
                                }
                              }
                              frame #11 {
                                n1243 = case shown="False" "Z100L" {
                                tunnel: w1214 -> [_ w1239]
                                tunnel: [0.0 ("MEASURE A") w1219] -> w1213
                                tunnel: w1212 -> [_ w1218]
                                tunnel: w1211 -> [_ w1216]
                                frame False {
                                }
                                frame True {
                                w1223 = "\t"
                                w1238 = i16 4 ("width (-)")
                                n1244 = property on="Time RLC" class="DigNum (strict)"() -> ("Value"=w1217:u32)  [unwired: 2 in, 2 out]
                                n1245 = Wait (ms)(milliseconds to wait=w1217) -> ()  [unwired: 1 out]
                                n1246 = Open/Create/Replace File(file path (use dialog)=w1216, operation (0:open)=T3."open") -> (refnum out=w1232:refnum<file>, error out=w1231:errorcluster)  [unwired: 2 in, 3 out]
                                n1247 = Set File Position(refnum=w1232, from (0:start)=enum16{"start", "end", "current"}."end", error in=w1231) -> (refnum out=w1234:refnum<file>, error out=w1235:errorcluster)  [unwired: 1 in]
                                n1248 = call "RLC_read.vi"("Path"=w1218, "String"="cmd /c rlc_read_ZBL.py") -> ("MEASURE A"=w1219:dbl, "MEASURE V [V]"=w1221:dbl, "concatenated string"=w1240:string, "MEASURE B"=w1222:dbl, "MEASURE I [A]"=w1220:dbl)  [unwired: 1 out]
                                "MEASURE A 11" <- w1219
                                "MEASURE B 11" <- w1222
                                n1249 = Number To Engineering String(2:w1238, 4:w1220) -> (0:w1224:string)  [unwired: 2 in]
                                n1250 = local write "RLC300 - digimess"(w1240) -> ()
                                n1251 = Number To Engineering String(2:w1238, 4:w1221) -> (0:w1225:string)  [unwired: 2 in]
                                n1252 = Number To Engineering String(2:w1238, 4:w1219) -> (0:w1227:string)  [unwired: 2 in]
                                n1253 = Number To Engineering String(2:w1238, 4:w1222) -> (0:w1226:string)  [unwired: 2 in]
                                n1254 = Concatenate Strings(w1227, w1223, w1226, w1223, w1225, w1223, w1224, w1223) -> (w1228:string)
                                n1255 = Write to Text File(file (use dialog)=w1234, text=w1228, error in=w1235) -> (refnum out=w1230:refnum<file>, error out=w1229:errorcluster)  [unwired: 1 in, 1 out]
                                n1256 = Close File(refnum=w1230, error in=w1229) -> (error out=w1237:errorcluster)  [unwired: 1 out]
                                n1257 = call <vilib>:"Simple Error Handler.vi"("error in (no error)"=w1237) -> ()  [unwired: 1 in, 8 out]
                                "Z-100-L" <- w1239
                                }
                                }
                              }
                              frame #12 {
                                n1258 = case shown="False" "Z100N" {
                                tunnel: w1246 -> [_ w1271]
                                tunnel: [0.0 ("MEASURE A") w1251] -> w1245
                                tunnel: w1244 -> [_ w1250]
                                tunnel: w1243 -> [_ w1248]
                                frame False {
                                }
                                frame True {
                                w1255 = "\t"
                                w1270 = i16 4 ("width (-)")
                                n1259 = property on="Time RLC" class="DigNum (strict)"() -> ("Value"=w1249:u32)  [unwired: 2 in, 2 out]
                                n1260 = Wait (ms)(milliseconds to wait=w1249) -> ()  [unwired: 1 out]
                                n1261 = Open/Create/Replace File(file path (use dialog)=w1248, operation (0:open)=T3."open") -> (refnum out=w1264:refnum<file>, error out=w1263:errorcluster)  [unwired: 2 in, 3 out]
                                n1262 = Set File Position(refnum=w1264, from (0:start)=enum16{"start", "end", "current"}."end", error in=w1263) -> (refnum out=w1266:refnum<file>, error out=w1267:errorcluster)  [unwired: 1 in]
                                n1263 = call "RLC_read.vi"("Path"=w1250, "String"="cmd /c rlc_read_ZBN.py") -> ("MEASURE A"=w1251:dbl, "MEASURE V [V]"=w1253:dbl, "concatenated string"=w1272:string, "MEASURE B"=w1254:dbl, "MEASURE I [A]"=w1252:dbl)  [unwired: 1 out]
                                "MEASURE A 12" <- w1251
                                "MEASURE B 12" <- w1254
                                n1264 = Number To Engineering String(2:w1270, 4:w1252) -> (0:w1256:string)  [unwired: 2 in]
                                n1265 = local write "RLC300 - digimess"(w1272) -> ()
                                n1266 = Number To Engineering String(2:w1270, 4:w1253) -> (0:w1257:string)  [unwired: 2 in]
                                n1267 = Number To Engineering String(2:w1270, 4:w1251) -> (0:w1259:string)  [unwired: 2 in]
                                n1268 = Number To Engineering String(2:w1270, 4:w1254) -> (0:w1258:string)  [unwired: 2 in]
                                n1269 = Concatenate Strings(w1259, w1255, w1258, w1255, w1257, w1255, w1256, w1255) -> (w1260:string)
                                n1270 = Write to Text File(file (use dialog)=w1266, text=w1260, error in=w1267) -> (refnum out=w1262:refnum<file>, error out=w1261:errorcluster)  [unwired: 1 in, 1 out]
                                n1271 = Close File(refnum=w1262, error in=w1261) -> (error out=w1269:errorcluster)  [unwired: 1 out]
                                n1272 = call <vilib>:"Simple Error Handler.vi"("error in (no error)"=w1269) -> ()  [unwired: 1 in, 8 out]
                                "Z-100-N" <- w1271
                                }
                                }
                              }
                              frame #13 {
                                n1273 = case shown="False" "Z1KL" {
                                tunnel: w1278 -> [_ w1303]
                                tunnel: [0.0 ("MEASURE A") w1283] -> w1277
                                tunnel: w1276 -> [_ w1282]
                                tunnel: w1275 -> [_ w1280]
                                frame False {
                                }
                                frame True {
                                w1287 = "\t"
                                w1302 = i16 4 ("width (-)")
                                n1274 = property on="Time RLC" class="DigNum (strict)"() -> ("Value"=w1281:u32)  [unwired: 2 in, 2 out]
                                n1275 = Wait (ms)(milliseconds to wait=w1281) -> ()  [unwired: 1 out]
                                n1276 = Open/Create/Replace File(file path (use dialog)=w1280, operation (0:open)=T3."open") -> (refnum out=w1296:refnum<file>, error out=w1295:errorcluster)  [unwired: 2 in, 3 out]
                                n1277 = Set File Position(refnum=w1296, from (0:start)=enum16{"start", "end", "current"}."end", error in=w1295) -> (refnum out=w1298:refnum<file>, error out=w1299:errorcluster)  [unwired: 1 in]
                                n1278 = call "RLC_read.vi"("Path"=w1282, "String"="cmd /c rlc_read_ZCL.py") -> ("MEASURE A"=w1283:dbl, "MEASURE V [V]"=w1285:dbl, "concatenated string"=w1304:string, "MEASURE B"=w1286:dbl, "MEASURE I [A]"=w1284:dbl)  [unwired: 1 out]
                                "MEASURE A 13" <- w1283
                                "MEASURE B 13" <- w1286
                                n1279 = Number To Engineering String(2:w1302, 4:w1284) -> (0:w1288:string)  [unwired: 2 in]
                                n1280 = local write "RLC300 - digimess"(w1304) -> ()
                                n1281 = Number To Engineering String(2:w1302, 4:w1285) -> (0:w1289:string)  [unwired: 2 in]
                                n1282 = Number To Engineering String(2:w1302, 4:w1283) -> (0:w1291:string)  [unwired: 2 in]
                                n1283 = Number To Engineering String(2:w1302, 4:w1286) -> (0:w1290:string)  [unwired: 2 in]
                                n1284 = Concatenate Strings(w1291, w1287, w1290, w1287, w1289, w1287, w1288, w1287) -> (w1292:string)
                                n1285 = Write to Text File(file (use dialog)=w1298, text=w1292, error in=w1299) -> (refnum out=w1294:refnum<file>, error out=w1293:errorcluster)  [unwired: 1 in, 1 out]
                                n1286 = Close File(refnum=w1294, error in=w1293) -> (error out=w1301:errorcluster)  [unwired: 1 out]
                                n1287 = call <vilib>:"Simple Error Handler.vi"("error in (no error)"=w1301) -> ()  [unwired: 1 in, 8 out]
                                "Z-1K-L" <- w1303
                                }
                                }
                              }
                              frame #14 {
                                n1288 = case shown="True" "Z1KN" {
                                tunnel: w1311 -> [_ w1337]
                                tunnel: [0.0 ("MEASURE A") w1318] -> w1310
                                tunnel: w1309 -> [_ w1317]
                                tunnel: w1308 -> [_ w1315]
                                tunnel: [_ w1314] -> w1306
                                frame False {
                                }
                                frame True {
                                w1321 = "\t"
                                w1336 = i16 6 ("width (-)")
                                n1289 = property on="Time RLC" class="DigNum (strict)"() -> ("Value"=w1316:u32)  [unwired: 2 in, 2 out]
                                n1290 = Wait (ms)(milliseconds to wait=w1316) -> ()  [unwired: 1 out]
                                n1291 = Open/Create/Replace File(file path (use dialog)=w1315, operation (0:open)=T3."open") -> (refnum out=w1330:refnum<file>, error out=w1329:errorcluster)  [unwired: 2 in, 3 out]
                                n1292 = Set File Position(refnum=w1330, from (0:start)=enum16{"start", "end", "current"}."end", error in=w1329) -> (refnum out=w1332:refnum<file>, error out=w1333:errorcluster)  [unwired: 1 in]
                                n1293 = call "RLC_read.vi"("Path"=w1317, "String"="cmd /c rlc_read_ZCN.py") -> ("MEASURE A"=w1318:dbl, "MEASURE V [V]"=w1320:dbl, "concatenated string"=w1338:string, "MEASURE B"=w1314:dbl, "MEASURE I [A]"=w1319:dbl)  [unwired: 1 out]
                                "MEASURE A 14" <- w1318
                                "MEASURE B 14" <- w1314
                                n1294 = Number To Engineering String(2:w1336, 4:w1319) -> (0:w1322:string)  [unwired: 2 in]
                                n1295 = local write "RLC300 - digimess"(w1338) -> ()
                                n1296 = Number To Engineering String(2:w1336, 4:w1320) -> (0:w1323:string)  [unwired: 2 in]
                                n1297 = Number To Engineering String(2:w1336, 4:w1318) -> (0:w1325:string)  [unwired: 2 in]
                                n1298 = Number To Engineering String(2:w1336, 4:w1314) -> (0:w1324:string)  [unwired: 2 in]
                                n1299 = Concatenate Strings(w1325, w1321, w1324, w1321, w1323, w1321, w1322, w1321, "\r\n") -> (w1326:string)
                                n1300 = Write to Text File(file (use dialog)=w1332, text=w1326, error in=w1333) -> (refnum out=w1328:refnum<file>, error out=w1327:errorcluster)  [unwired: 1 in, 1 out]
                                n1301 = Close File(refnum=w1328, error in=w1327) -> (error out=w1335:errorcluster)  [unwired: 1 out]
                                n1302 = call <vilib>:"Simple Error Handler.vi"("error in (no error)"=w1335) -> ()  [unwired: 1 in, 8 out]
                                "Z-1K-N" <- w1337
                                }
                                }
                              }
                              frame #15 {
                                n1303 = case shown="False" "Z10KL" {
                                tunnel: w1344 -> [_ w1369]
                                tunnel: [0.0 ("MEASURE A") w1349] -> w1343
                                tunnel: w1342 -> [_ w1348]
                                tunnel: w1341 -> [_ w1346]
                                frame False {
                                }
                                frame True {
                                w1353 = "\t"
                                w1368 = i16 4 ("width (-)")
                                n1304 = property on="Time RLC" class="DigNum (strict)"() -> ("Value"=w1347:u32)  [unwired: 2 in, 2 out]
                                n1305 = Wait (ms)(milliseconds to wait=w1347) -> ()  [unwired: 1 out]
                                n1306 = Open/Create/Replace File(file path (use dialog)=w1346, operation (0:open)=T3."open") -> (refnum out=w1362:refnum<file>, error out=w1361:errorcluster)  [unwired: 2 in, 3 out]
                                n1307 = Set File Position(refnum=w1362, from (0:start)=enum16{"start", "end", "current"}."end", error in=w1361) -> (refnum out=w1364:refnum<file>, error out=w1365:errorcluster)  [unwired: 1 in]
                                n1308 = call "RLC_read.vi"("Path"=w1348, "String"="cmd /c rlc_read_ZDL.py") -> ("MEASURE A"=w1349:dbl, "MEASURE V [V]"=w1351:dbl, "concatenated string"=w1370:string, "MEASURE B"=w1352:dbl, "MEASURE I [A]"=w1350:dbl)  [unwired: 1 out]
                                "MEASURE A 15" <- w1349
                                "MEASURE B 15" <- w1352
                                n1309 = Number To Engineering String(2:w1368, 4:w1350) -> (0:w1354:string)  [unwired: 2 in]
                                n1310 = local write "RLC300 - digimess"(w1370) -> ()
                                n1311 = Number To Engineering String(2:w1368, 4:w1351) -> (0:w1355:string)  [unwired: 2 in]
                                n1312 = Number To Engineering String(2:w1368, 4:w1349) -> (0:w1357:string)  [unwired: 2 in]
                                n1313 = Number To Engineering String(2:w1368, 4:w1352) -> (0:w1356:string)  [unwired: 2 in]
                                n1314 = Concatenate Strings(w1357, w1353, w1356, w1353, w1355, w1353, w1354, w1353) -> (w1358:string)
                                n1315 = Write to Text File(file (use dialog)=w1364, text=w1358, error in=w1365) -> (refnum out=w1360:refnum<file>, error out=w1359:errorcluster)  [unwired: 1 in, 1 out]
                                n1316 = Close File(refnum=w1360, error in=w1359) -> (error out=w1367:errorcluster)  [unwired: 1 out]
                                n1317 = call <vilib>:"Simple Error Handler.vi"("error in (no error)"=w1367) -> ()  [unwired: 1 in, 8 out]
                                "Z-10K-L" <- w1369
                                }
                                }
                              }
                              frame #16 {
                                n1318 = case shown="True" "Z10KN" {
                                tunnel: w1376 -> [_ w1402]
                                tunnel: [0.0 ("MEASURE A") w1381] -> w1375
                                tunnel: w1374 -> [_ w1380]
                                tunnel: w1373 -> [_ w1378]
                                frame False {
                                }
                                frame True {
                                w1386 = "\t"
                                w1401 = i16 4 ("width (-)")
                                n1319 = property on="Time RLC" class="DigNum (strict)"() -> ("Value"=w1379:u32)  [unwired: 2 in, 2 out]
                                n1320 = Wait (ms)(milliseconds to wait=w1379) -> ()  [unwired: 1 out]
                                n1321 = Open/Create/Replace File(file path (use dialog)=w1378, operation (0:open)=T3."open") -> (refnum out=w1395:refnum<file>, error out=w1394:errorcluster)  [unwired: 2 in, 3 out]
                                n1322 = Set File Position(refnum=w1395, from (0:start)=enum16{"start", "end", "current"}."end", error in=w1394) -> (refnum out=w1397:refnum<file>, error out=w1398:errorcluster)  [unwired: 1 in]
                                n1323 = call "RLC_read.vi"("Path"=w1380, "String"="cmd /c rlc_read_ZDN.py") -> ("MEASURE A"=w1381:dbl, "MEASURE V [V]"=w1384:dbl, "concatenated string"=w1403:string, "MEASURE B"=w1385:dbl, "MEASURE I [A]"=w1383:dbl)  [unwired: 1 out]
                                "MEASURE A 16" <- w1381
                                "MEASURE B 16" <- w1385
                                n1324 = Number To Engineering String(2:w1401, 4:w1383) -> (0:w1387:string)  [unwired: 2 in]
                                n1325 = local write "RLC300 - digimess"(w1403) -> ()
                                n1326 = Number To Engineering String(2:w1401, 4:w1384) -> (0:w1388:string)  [unwired: 2 in]
                                n1327 = Number To Engineering String(2:w1401, 4:w1381) -> (0:w1390:string)  [unwired: 2 in]
                                n1328 = Number To Engineering String(2:w1401, 4:w1385) -> (0:w1389:string)  [unwired: 2 in]
                                n1329 = Concatenate Strings(w1390, w1386, w1389, w1386, w1388, w1386, w1387, w1386, "\r\n") -> (w1391:string)
                                n1330 = Write to Text File(file (use dialog)=w1397, text=w1391, error in=w1398) -> (refnum out=w1393:refnum<file>, error out=w1392:errorcluster)  [unwired: 1 in, 1 out]
                                n1331 = Close File(refnum=w1393, error in=w1392) -> (error out=w1400:errorcluster)  [unwired: 1 out]
                                n1332 = call <vilib>:"Simple Error Handler.vi"("error in (no error)"=w1400) -> ()  [unwired: 1 in, 8 out]
                                "Z-10K-N" <- w1402
                                }
                                }
                              }
                              frame #17 {
                                n1333 = local write "Z-50-L"(w1406) -> ()
                                n1334 = local write "Z-1K-L"(w1406) -> ()
                                n1335 = local write "Z-1K-N"(w1406) -> ()
                                n1336 = local write "C-50-N"(w1406) -> ()
                                n1337 = local write "C-50-L"(w1406) -> ()
                                n1338 = local write "Z-50-N"(w1406) -> ()
                                n1339 = local write "C-1K-N"(w1406) -> ()
                                n1340 = local write "C-1K-L"(w1406) -> ()
                                n1341 = local write "Z-100-L"(w1406) -> ()
                                n1342 = local write "Z-100-N"(w1406) -> ()
                                n1343 = local write "Z-10K-L"(w1406) -> ()
                                n1344 = local write "Z-10K-N"(w1406) -> ()
                                n1345 = local write "C-10K-N"(w1406) -> ()
                                n1346 = local write "C-10K-L"(w1406) -> ()
                                n1347 = local write "C-100-N"(w1406) -> ()
                                n1348 = local write "C-100-L"(w1406) -> ()
                              }
                            }
                          }
                          n1349 = call <vilib>:"Mean.vi"("X"=w837) -> ("mean"=w819:dbl)  [unwired: 1 out]
                          "mean" <- w819
                          n1350 = call <vilib>:"Mean.vi"("X"=w836) -> ("mean"=w818:dbl)  [unwired: 1 out]
                          "mean 2" <- w818
                          n1351 = call <vilib>:"Mean.vi"("X"=w835) -> ("mean"=w817:dbl)  [unwired: 1 out]
                          "mean 3" <- w817
                          n1352 = call <vilib>:"Mean.vi"("X"=w834) -> ("mean"=w816:dbl)  [unwired: 1 out]
                          "mean 4" <- w816
                          n1353 = call <vilib>:"Mean.vi"("X"=w833) -> ("mean"=w815:dbl)  [unwired: 1 out]
                          "mean 5" <- w815
                          n1354 = call <vilib>:"Mean.vi"("X"=w832) -> ("mean"=w814:dbl)  [unwired: 1 out]
                          "mean 6" <- w814
                          n1355 = call <vilib>:"Mean.vi"("X"=w831) -> ("mean"=w813:dbl)  [unwired: 1 out]
                          "mean 7" <- w813
                          n1356 = call <vilib>:"Mean.vi"("X"=w830) -> ("mean"=w812:dbl)  [unwired: 1 out]
                          "mean 8" <- w812
                          n1357 = call <vilib>:"Mean.vi"("X"=w829) -> ("mean"=w811:dbl)  [unwired: 1 out]
                          "mean 9" <- w811
                          n1358 = call <vilib>:"Mean.vi"("X"=w828) -> ("mean"=w810:dbl)  [unwired: 1 out]
                          "mean 10" <- w810
                          n1359 = call <vilib>:"Mean.vi"("X"=w827) -> ("mean"=w809:dbl)  [unwired: 1 out]
                          "mean 11" <- w809
                          n1360 = call <vilib>:"Mean.vi"("X"=w826) -> ("mean"=w808:dbl)  [unwired: 1 out]
                          "mean 12" <- w808
                          n1361 = call <vilib>:"Mean.vi"("X"=w825) -> ("mean"=w807:dbl)  [unwired: 1 out]
                          "mean 13" <- w807
                          n1362 = call <vilib>:"Mean.vi"("X"=w824) -> ("mean"=w806:dbl)  [unwired: 1 out]
                          "mean 14" <- w806
                          n1363 = call <vilib>:"Mean.vi"("X"=w823) -> ("mean"=w805:dbl)  [unwired: 1 out]
                          "mean 15" <- w805
                          n1364 = call <vilib>:"Mean.vi"("X"=w822) -> ("mean"=w804:dbl)  [unwired: 1 out]
                          "mean 16" <- w804
                          n1365 = call <vilib>:"Mean.vi"("X"=w803) -> ("mean"=w802:dbl)  [unwired: 1 out]
                          "mean 17" <- w802
                          n1366 = call <vilib>:"Mean.vi"("X"=w800) -> ("mean"=w801:dbl)  [unwired: 1 out]
                          "mean 18" <- w801
                        }
                      }
                    }
                    frame #2 {
                      n1367 = case shown="True" w1409 {
                        tunnel: w1426 -> [_ w1450]
                        tunnel: w1425 -> [_ w1449]
                        tunnel: w1424 -> [_ w1448]
                        tunnel: w1423 -> [_ w1447]
                        tunnel: w1422 -> [_ w1446]
                        tunnel: w1421 -> [_ w1445]
                        tunnel: w1420 -> [_ w1444]
                        tunnel: w1419 -> [_ w1443]
                        tunnel: w1418 -> [_ w1442]
                        tunnel: w1417 -> [_ w1441]
                        tunnel: w1416 -> [_ w1440]
                        tunnel: w1415 -> [_ w1439]
                        tunnel: w1414 -> [_ w1438]
                        tunnel: w1413 -> [_ w1437]
                        tunnel: w1412 -> [_ w1436]
                        tunnel: w1411 -> [_ w1435]
                        tunnel: w1408 -> [_ w1428]
                        tunnel: w1407 -> [_ w1427]
                        frame False {
                        }
                        frame True {
                          w1434 = "\t"
                          w1479 = i16 6 ("precision (6)")
                          n1368 = property on="SET" class="DigNum (strict)"() -> ("Value"=w1480:i32)  [unwired: 2 in, 2 out]
                          n1369 = Number To Engineering String(2:i16 6 ("precision (6)"), 4:w1428) -> (0:w1432:string)  [unwired: 2 in]
                          n1370 = Number To Engineering String(2:i16 6 ("precision (6)"), 4:w1427) -> (0:w1429:string)  [unwired: 2 in]
                          n1371 = Number To Engineering String(2:w1479, 4:w1450) -> (0:w1477:string)  [unwired: 2 in]
                          n1372 = Number To Engineering String(2:w1479, 4:w1435) -> (0:w1476:string)  [unwired: 2 in]
                          n1373 = Number To Engineering String(2:w1479, 4:w1449) -> (0:w1475:string)  [unwired: 2 in]
                          n1374 = Number To Engineering String(2:w1479, 4:w1448) -> (0:w1474:string)  [unwired: 2 in]
                          n1375 = Number To Engineering String(2:w1479, 4:w1447) -> (0:w1473:string)  [unwired: 2 in]
                          n1376 = Number To Engineering String(2:w1479, 4:w1446) -> (0:w1472:string)  [unwired: 2 in]
                          n1377 = Number To Engineering String(2:w1479, 4:w1445) -> (0:w1471:string)  [unwired: 2 in]
                          n1378 = Number To Engineering String(2:w1479, 4:w1444) -> (0:w1470:string)  [unwired: 2 in]
                          n1379 = Number To Engineering String(2:w1479, 4:w1443) -> (0:w1469:string)  [unwired: 2 in]
                          n1380 = Number To Engineering String(2:w1479, 4:w1442) -> (0:w1468:string)  [unwired: 2 in]
                          n1381 = Number To Engineering String(2:w1479, 4:w1441) -> (0:w1467:string)  [unwired: 2 in]
                          n1382 = Number To Engineering String(2:w1479, 4:w1440) -> (0:w1466:string)  [unwired: 2 in]
                          n1383 = Number To Engineering String(2:w1479, 4:w1439) -> (0:w1465:string)  [unwired: 2 in]
                          n1384 = Number To Engineering String(2:w1479, 4:w1438) -> (0:w1464:string)  [unwired: 2 in]
                          n1385 = Number To Engineering String(2:w1479, 4:w1437) -> (0:w1463:string)  [unwired: 2 in]
                          n1386 = Number To Engineering String(2:w1479, 4:w1436) -> (0:w1462:string)  [unwired: 2 in]
                          n1387 = Number To Decimal String(number=w1480) -> (decimal integer string=w1478:string)  [unwired: 1 in]
                          n1388 = property on="path RLC_mean" class="Path"() -> ("Value"=w1451:path)  [unwired: 2 in, 2 out]
                          n1389 = Open/Create/Replace File(file path (use dialog)=w1451, operation (0:open)=T3."open") -> (refnum out=w1456:refnum<file>, error out=w1455:errorcluster)  [unwired: 2 in, 3 out]
                          n1390 = Concatenate Strings(w1478, w1434, w1477, w1434, w1476, w1434, w1475, w1434, w1474, w1434, w1473, w1434, w1472, w1434, w1471, w1434, w1470, w1434, w1469, w1434, w1468, w1434, w1467, w1434, w1466, w1434, w1465, w1434, w1464, w1434, w1463, w1434, w1462, w1434, w1432, w1434, w1429, "\r\n") -> (w1452:string)
                          n1391 = Set File Position(refnum=w1456, from (0:start)=enum16{"start", "end", "current"}."end", error in=w1455) -> (refnum out=w1458:refnum<file>, error out=w1459:errorcluster)  [unwired: 1 in]
                          n1392 = Write to Text File(file (use dialog)=w1458, text=w1452, error in=w1459) -> (refnum out=w1454:refnum<file>, error out=w1453:errorcluster)  [unwired: 1 in, 1 out]
                          n1393 = Close File(refnum=w1454, error in=w1453) -> (error out=w1461:errorcluster)  [unwired: 1 out]
                          n1394 = call <vilib>:"Simple Error Handler.vi"("error in (no error)"=w1461) -> ()  [unwired: 1 in, 8 out]
                        }
                      }
                    }
                  }
                  n1395 = local write "graph RLC"(w749) -> ()
                }
                frame 9 {
                  n1396 = flat-sequence {
                    tunnel: w1519 -> [w1530]
                    tunnel: [w1530] -> w1518
                    tunnel: [w1524] -> w1517
                    tunnel: [w1523] -> w1516
                    tunnel: w1518 -> [w1555]
                    tunnel: w1517 -> [_]
                    tunnel: w1516 -> [w1552]
                    frame #0 {
                      n1397 = property on="SET" class="DigNum (strict)"() -> ("Value"=w1528:i32)  [unwired: 2 in, 2 out]
                      n1398 = Increment(x=w1528) -> (x+1=w1523:i32)
                      n1399 = property on="P_max camara" class="DigNum (strict)"() -> ("Value"=w1521:dbl)  [unwired: 2 in, 2 out]
                      n1400 = local write "SET"(w1523) -> ()
                      n1401 = property on="Camara 2" class="Slide (strict)"() -> ("Value"=w1522:dbl)  [unwired: 2 in, 2 out]
                      n1402 = case shown="False" "Boolean" {
                        selector: "Boolean" -> [w1536 w1541]
                        tunnel: [w1538 w1545] -> w1525
                        tunnel: w1523 -> [w1539 _]
                        frame False {
                          n1403 = local write "Boolean 2"(w1536) -> ()
                          n1404 = Index Array(array="Array", index=w1539) -> (element=w1538:dbl)
                          n1405 = Not(x=w1536) -> (.not. x?=→"Boolean 3":bool)
                        }
                        frame True {
                          n1406 = property on="Set P auto" class="DigNum (strict)"() -> ("Value"=w1543:dbl)  [unwired: 2 in, 2 out]
                          n1407 = Add(x="Step P", y=w1543) -> (x+y=w1545:dbl)
                          n1408 = Not(x=w1541) -> (.not. x?=w1542:bool)
                          n1409 = local write "Boolean 3"(w1542) -> ()
                          "Boolean 2" <- w1541
                        }
                      }
                      n1410 = Greater?(x=w1522, y=w1521) -> (0:w1520:bool)
                      n1411 = case shown="True" w1520 {
                        frame False {
                        }
                        frame True {
                          n1412 = property on="Desc SET" class="DigNum (strict)"() -> ("Value"=w1532:i32)  [unwired: 2 in, 2 out]
                          n1413 = local write "Descarga"(TRUE ("Descarga")) -> ()
                          n1414 = Increment(x=w1532) -> (x+1=w1531:i32)
                          n1415 = local write "Desc SET"(w1531) -> ()
                        }
                      }
                      n1416 = Greater?(x=w1525, y="P_max") -> (0:w1527:bool)
                      n1417 = case shown="True" w1527 {
                        tunnel: [w1534 w1535] -> w1524
                        tunnel: "P_max" -> [_ w1535]
                        tunnel: w1525 -> [w1534 _]
                        frame False {
                        }
                        frame True {
                        }
                      }
                      n1418 = local write "Set P auto"(w1524) -> ()
                    }
                    frame #1 {
                      n1419 = property on="Desc SET" class="DigNum (strict)"() -> ("Value"=w1547:i32)  [unwired: 2 in, 2 out]
                      n1420 = Quotient & Remainder(x=w1552, y="Step ZPit") -> (x-y*floor(x/y)=w1553:dbl)  [unwired: 1 out]
                      n1421 = Greater Than 0?(x=w1547) -> (x > 0?=w1549:bool)
                      n1422 = Equal To 0?(x=w1553) -> (x = 0?=w1551:bool)
                      "Read ZPit" <- w1551
                      n1423 = property on="Descarga" class="Bool (strict)"() -> ("Value"=w1546:bool)  [unwired: 2 in, 2 out]
                      n1424 = And(x=w1549, y=w1546) -> (x .and. y?=w1548:bool)
                      n1425 = case shown="True" w1548 {
                        tunnel: w1551 -> [w1556 _]
                        tunnel: [w1556 w1557] -> w1550
                        frame False {
                        }
                        frame True {
                          w1557 = TRUE
                          n1426 = local write "Read ZPit"(w1557) -> ()
                        }
                      }
                      n1427 = case shown="True" w1550 {
                        tunnel: w1555 -> [_ w1559]
                        frame False {
                          n1428 = local write "Estagio auto"(11 ("Estagio auto")) -> ()
                        }
                        frame True {
                          n1429 = Greater?(x=w1559, y=1.0) -> (0:w1564:bool)
                          n1430 = case shown="True" w1564 {
                            tunnel: [FALSE ("Boolean") TRUE ("Boolean")] -> w1562
                            frame False {
                              w1584 = TRUE ("Boolean")
                              n1431 = local write "Vácuo 2"(w1584) -> ()
                              n1432 = Multiply(x="ZPf2 time", y=0.0741) -> (x*y=w1579:dbl)
                              n1433 = local write "String"("Limpar volume referencia" ("String")) -> ()
                              n1434 = Add(x=w1579, y=1.9801) -> (x+y=w1577:dbl)
                              n1435 = call "Controle_vacuo.vi"("time (s) to wait vacuo"=w1577, "Boolean"=w1584) -> ("Vacuo"=w1585:bool)  [unwired: 9 in]
                              n1436 = local write "Vácuo 2"(w1585) -> ()
                            }
                            frame True {
                              n1437 = property on="ATM wait" class="DigNum (strict)"() -> ("Value"=w1586:u32)  [unwired: 2 in, 2 out]
                              n1438 = call "Controle_ATM.vi"("seconds to wait"=w1586) -> ("String 2"=w1589:string, "Atm"=w1588:bool)  [unwired: 9 in]
                              n1439 = local write "Atm 2"(w1588) -> ()
                              n1440 = local write "String"(w1589) -> ()
                            }
                          }
                          n1441 = for {
                            N: 1 -> [_]
                            tunnel: [w1566] -> w1561
                            tunnel: w1562 -> [w1566]
                            n1442 = Wait (ms)(milliseconds to wait=u32 500 ("x")) -> ()  [unwired: 1 out]
                          }
                          n1443 = case shown="True" w1561 {
                            frame False {
                              n1444 = local write "Estagio auto"(10 ("Estagio auto")) -> ()
                            }
                            frame True {
                              w1575 = TRUE ("Boolean")
                              n1445 = property on="ZPf2 time" class="DigNum (strict)"() -> ("Value"=w1569:dbl)  [unwired: 2 in, 2 out]
                              n1446 = local write "Estagio auto"(10 ("Estagio auto")) -> ()
                              n1447 = local write "Vácuo 2"(w1575) -> ()
                              n1448 = Multiply(x=w1569, y=0.0741) -> (x*y=w1571:dbl)
                              n1449 = local write "String"("Limpar volume referencia" ("String")) -> ()
                              n1450 = Add(x=w1571, y=1.9801) -> (x+y=w1568:dbl)
                              n1451 = call "Controle_vacuo.vi"("time (s) to wait vacuo"=w1568, "Boolean"=w1575) -> ("Vacuo"=w1576:bool)  [unwired: 9 in]
                              n1452 = local write "Vácuo 2"(w1576) -> ()
                            }
                          }
                        }
                      }
                    }
                  }
                }
                frame 10 {
                  n1453 = property on="Contador" class="DigNum (strict)"() -> ("Value"=w1591:i32)  [unwired: 2 in, 2 out]
                  n1454 = Increment(x=w1591) -> (x+1=w1593:i32)
                  n1455 = local write "String"("Ler ZPf2 e T" ("String")) -> ()
                  n1456 = property on="N fit 2" class="DigNum (strict)"() -> ("Value"=w1590:i32)  [unwired: 2 in, 2 out]
                  n1457 = Equal?(x=w1593, y=w1590) -> (x = y?=w1592:bool)
                  n1458 = case shown="True" w1592 {
                    frame False {
                    }
                    frame True {
                      n1459 = local write "Estagio auto"(11 ("Estagio auto")) -> ()
                    }
                  }
                }
                frame 11 {
                  n1460 = property on="Contador" class="DigNum (strict)"() -> ("Value"=w1599:i32)  [unwired: 2 in, 2 out]
                  n1461 = Increment(x=w1599) -> (x+1=w1600:i32)
                  n1462 = property on="N fit 2" class="DigNum (strict)"() -> ("Value"=w1596:i32)  [unwired: 2 in, 2 out]
                  n1463 = Equal?(x=w1600, y=w1596) -> (x = y?=w1598:bool)
                  n1464 = case shown="True" w1598 {
                    tunnel: w1601 -> [_ w1612]
                    tunnel: w1597 -> [_ w1602]
                    frame False {
                    }
                    frame True {
                      w1603 = i16 3 ("precision (6)")
                      w1606 = "\t"
                      n1465 = property on="T fit" class="DigNum (strict)"() -> ("Value"=w1608:dbl)  [unwired: 2 in, 2 out]
                      n1466 = property on="Read ZPit" class="Bool (strict)"() -> ("Value"=w1607:bool)  [unwired: 2 in, 2 out]
                      n1467 = case shown="False" w1607 {
                        tunnel: ["  ==>" w1618] -> w1611
                        tunnel: w1603 -> [_ w1617]
                        frame False {
                        }
                        frame True {
                          n1468 = property on="P fit" class="DigNum (strict)"() -> ("Value"=w1616:dbl)  [unwired: 2 in, 2 out]
                          n1469 = Number To Fractional String(number=w1616, precision (6)=w1617) -> (F-format string=w1618:string)  [unwired: 2 in]
                        }
                      }
                      n1470 = Number To Fractional String(number=w1608, precision (6)=w1603) -> (F-format string=w1610:string)  [unwired: 2 in]
                      n1471 = Number To Fractional String(number=w1602, precision (6)=w1603) -> (F-format string=w1605:string)  [unwired: 2 in]
                      n1472 = Concatenate Strings(w1611, w1606, w1610, w1606, w1605, "\r\n") -> (w1609:string)
                      n1473 = flat-sequence {
                        tunnel: [w1622] -> w1614
                        tunnel: [w1621] -> w1613
                        tunnel: w1609 -> [w1620]
                        tunnel: w1612 -> [w1619]
                        tunnel: w1614 -> [w1636]
                        tunnel: w1613 -> [w1635]
                        frame #0 {
                          n1474 = Open/Create/Replace File(file path (use dialog)=w1619, operation (0:open)=T3."open") -> (refnum out=w1628:refnum<file>, error out=w1629:errorcluster)  [unwired: 2 in, 3 out]
                          n1475 = Set File Position(refnum=w1628, from (0:start)=enum16{"start", "end", "current"}."end", error in=w1629) -> (refnum out=w1626:refnum<file>, error out=w1625:errorcluster)  [unwired: 1 in]
                          n1476 = Write to Text File(file (use dialog)=w1626, text=w1620, error in=w1625) -> (refnum out=w1630:refnum<file>, error out=w1631:errorcluster)  [unwired: 2 out]
                          n1477 = Close File(refnum=w1630, error in=w1631) -> (path=w1622:path, error out=w1623:errorcluster)
                          n1478 = call <vilib>:"Simple Error Handler.vi"("error in (no error)"=w1623) -> ("error out"=w1621:errorcluster)  [unwired: 1 in, 7 out]
                        }
                        frame #1 {
                          w1632 = TRUE ("ZPit")
                          n1479 = Wait (ms)(milliseconds to wait=u32 500) -> ()  [unwired: 1 out]
                          n1480 = local write "T 2"(w1632) -> ()
                          n1481 = local write "ZPf2 2"(w1632) -> ()
                          n1482 = Read from Text File(file (use dialog)=w1636, count=-1 ("Count  3"), error in=w1635) -> (refnum out=w1637:refnum<file>, text=w1641:string, error out=w1638:errorcluster)  [unwired: 1 in, 1 out]
                          n1483 = local write "String 3"(w1641) -> ()
                          n1484 = Close File(refnum=w1637, error in=w1638) -> (error out=w1639:errorcluster)  [unwired: 1 out]
                          n1485 = call <vilib>:"Simple Error Handler.vi"("error in (no error)"=w1639) -> ()  [unwired: 1 in, 8 out]
                          n1486 = local write "String"("abrir valvula entrada gas" ("String")) -> ()
                        }
                        frame #2 {
                          n1487 = property on="Desc SET" class="DigNum (strict)"() -> ("Value"=w1643:i32)  [unwired: 2 in, 2 out]
                          n1488 = Greater Than 0?(x=w1643) -> (x > 0?=w1642:bool)
                          n1489 = property on="Camara 2" class="Slide (strict)"() -> ("Value"=w1650:dbl)  [unwired: 2 in, 2 out]
                          n1490 = Greater?(x=w1650, y="P_max camara") -> (0:w1648:bool)
                          n1491 = property on="Carga" class="Bool (strict)"() -> ("Value"=w1647:bool)  [unwired: 2 in, 2 out]
                          n1492 = And(x=w1648, y=w1647) -> (x .and. y?=w1645:bool)
                          n1493 = case shown="False" w1642 {
                            tunnel: w1645 -> [w1651 _]
                            tunnel: [w1651 TRUE] -> w1644
                            frame False {
                            }
                            frame True {
                            }
                          }
                          n1494 = case shown="True" w1644 {
                            tunnel: [5 ("N fit") w1657] -> w1646
                            frame False {
                              n1495 = local write "Estagio auto"(0 ("Estagio auto")) -> ()
                              "Carga" <- TRUE
                              "Descarga" <- FALSE
                            }
                            frame True {
                              n1496 = local write "teste slope"(0 ("teste slope")) -> ()
                              n1497 = local write "Carga"(FALSE ("Carga")) -> ()
                              n1498 = local write "Descarga"(TRUE ("Descarga")) -> ()
                              n1499 = local write "Estagio auto"(12 ("Estagio auto")) -> ()
                              n1500 = property on="N fit 2" class="DigNum (strict)"() -> ("Value"=w1657:i32)  [unwired: 2 in, 2 out]
                            }
                          }
                          n1501 = local write "N fit"(w1646) -> ()
                        }
                      }
                    }
                  }
                }
                frame 12 {
                  w1667 = "\t"
                  n1502 = property on="SET" class="DigNum (strict)"() -> ("Value"=w1671:i32)  [unwired: 2 in, 2 out]
                  n1503 = Number To Decimal String(number=w1671) -> (decimal integer string=w1674:string)  [unwired: 1 in]
                  n1504 = Number To Fractional String(number=0.0, precision (6)=i16 3) -> (F-format string=w1668:string)  [unwired: 2 in]
                  n1505 = Concatenate Strings(w1674, w1667, w1668, w1667, w1668, w1667) -> (w1673:string)
                  n1506 = flat-sequence {
                    tunnel: w1670 -> [w1679]
                    tunnel: w1673 -> [w1680]
                    tunnel: [w1680] -> w1666
                    tunnel: [w1679] -> w1665
                    tunnel: [w1684] -> w1676
                    tunnel: [w1683] -> w1675
                    tunnel: w1666 -> [w1682]
                    tunnel: w1665 -> [w1681]
                    tunnel: [w1681] -> w1664
                    tunnel: w1676 -> [w1700]
                    tunnel: w1675 -> [w1699]
                    tunnel: w1664 -> [w1694]
                    tunnel: [w1694] -> w1663
                    tunnel: w1663 -> [w1708]
                    tunnel: [w1707] -> w1662
                    tunnel: w1662 -> [w1745]
                    frame #0 {
                      w1678 = FALSE ("ZPit 2")
                      n1507 = Wait (ms)(milliseconds to wait=u32 1000) -> ()  [unwired: 1 out]
                      n1508 = local write "ZPit 2"(w1678) -> ()
                      n1509 = local write "Pit 2"(w1678) -> ()
                      n1510 = local write "Pf2 2"(w1678) -> ()
                      n1511 = local write "ZPf2 2"(w1678) -> ()
                      n1512 = local write "T 2"(w1678) -> ()
                    }
                    frame #1 {
                      n1513 = Open/Create/Replace File(file path (use dialog)=w1681, operation (0:open)=T3."open") -> (refnum out=w1690:refnum<file>, error out=w1691:errorcluster)  [unwired: 2 in, 3 out]
                      n1514 = Set File Position(refnum=w1690, from (0:start)=enum16{"start", "end", "current"}."end", error in=w1691) -> (refnum out=w1688:refnum<file>, error out=w1687:errorcluster)  [unwired: 1 in]
                      n1515 = Write to Text File(file (use dialog)=w1688, text=w1682, error in=w1687) -> (refnum out=w1692:refnum<file>, error out=w1693:errorcluster)  [unwired: 2 out]
                      n1516 = Close File(refnum=w1692, error in=w1693) -> (path=w1684:path, error out=w1685:errorcluster)
                      n1517 = call <vilib>:"Simple Error Handler.vi"("error in (no error)"=w1685) -> ("error out"=w1683:errorcluster)  [unwired: 1 in, 7 out]
                    }
                    frame #2 {
                      w1695 = TRUE ("ZPit")
                      n1518 = local write "Estagio auto"(7 ("Estagio auto")) -> ()
                      n1519 = Wait (ms)(milliseconds to wait=u32 500) -> ()  [unwired: 1 out]
                      n1520 = local write "ZPit 2"(w1695) -> ()
                      n1521 = local write "Pit 2"(w1695) -> ()
                      n1522 = Read from Text File(file (use dialog)=w1700, count=-1 ("Count  3"), error in=w1699) -> (refnum out=w1701:refnum<file>, text=w1705:string, error out=w1702:errorcluster)  [unwired: 1 in, 1 out]
                      n1523 = local write "String 3"(w1705) -> ()
                      n1524 = Close File(refnum=w1701, error in=w1702) -> (error out=w1703:errorcluster)  [unwired: 1 out]
                      n1525 = call <vilib>:"Simple Error Handler.vi"("error in (no error)"=w1703) -> ()  [unwired: 1 in, 8 out]
                      n1526 = local write "String"("abrir valvula camara" ("String")) -> ()
                    }
                    frame #3 {
                      n1527 = property on="Camara 2" class="Slide (strict)"() -> ("Value"=w1711:dbl)  [unwired: 2 in, 2 out]
                      n1528 = Less?(x=w1711, y="P_min descarga") -> (x < y?=w1706:bool)
                      n1529 = property on="Efetuados" class="DigNum (strict)"() -> ("Value"=w1709:dbl)  [unwired: 2 in, 2 out]
                      n1530 = case shown="True" w1706 {
                        tunnel: w1709 -> [_ w1740]
                        tunnel: w1708 -> [_ w1729]
                        tunnel: [TRUE ("data") FALSE ("data")] -> w1707
                        tunnel: w1706 -> [_ w1718]
                        frame False {
                          n1531 = property on="Desc SET" class="DigNum (strict)"() -> ("Value"=w1713:i32)  [unwired: 2 in, 2 out]
                          n1532 = Increment(x=w1713) -> (x+1=→"Desc SET":i32)
                        }
                        frame True {
                          w1727 = "\r\n"
                          n1533 = Increment(x=w1740) -> (x+1=w1715:dbl)
                          "Efetuados" <- w1715
                          n1534 = local write "Estagio auto"(0 ("Estagio auto")) -> ()
                          n1535 = local write "SET"(0 ("SET")) -> ()
                          n1536 = local write "Desc SET"(0 ("Desc SET")) -> ()
                          n1537 = local write "Carga"(TRUE ("Carga")) -> ()
                          n1538 = local write "Descarga"(FALSE ("Descarga")) -> ()
                          n1539 = local write "Set P auto"(0.5 ("Set P auto")) -> ()
                          n1540 = Open/Create/Replace File(file path (use dialog)=w1729, operation (0:open)=T3."open") -> (refnum out=w1735:refnum<file>, error out=w1736:errorcluster)  [unwired: 2 in, 3 out]
                          n1541 = Less Or Equal?(x="Ciclos", y=w1715) -> (x <= y?=w1716:bool)
                          n1542 = And(x=w1718, y=w1716) -> (x .and. y?=w1719:bool)
                          n1543 = Set File Position(refnum=w1735, from (0:start)=enum16{"start", "end", "current"}."end", error in=w1736) -> (refnum out=w1733:refnum<file>, error out=w1732:errorcluster)  [unwired: 1 in]
                          n1544 = case shown="False" w1719 {
                            frame False {
                              n1545 = local write "FIM"(FALSE ("FIM")) -> ()
                            }
                            frame True {
                              w1744 = 1 ("N fit")
                              n1546 = local write "Auto Ctrl"(FALSE ("Auto Ctrl")) -> ()
                              n1547 = local write "N fit"(w1744) -> ()
                              n1548 = local write "N to fit"(w1744) -> ()
                              "FIM" <- TRUE ("stop")
                            }
                          }
                          n1549 = Concatenate Strings(w1727, ">>>>>>>>>>>>>>" ("string"), w1727, w1727) -> (w1726:string)
                          n1550 = Write to Text File(file (use dialog)=w1733, text=w1726, error in=w1732) -> (refnum out=w1737:refnum<file>, error out=w1738:errorcluster)  [unwired: 2 out]
                          n1551 = Close File(refnum=w1737, error in=w1738) -> (error out=w1730:errorcluster)  [unwired: 1 out]
                          n1552 = call <vilib>:"Simple Error Handler.vi"("error in (no error)"=w1730) -> ()  [unwired: 1 in, 8 out]
                        }
                      }
                    }
                    frame #4 {
                      w1747 = T4 3 items=["no dialog", "OK message", "continue or stop message", "OK message + warnings", "continue/stop + warnings"] ("type of dialog (OK msg:1)")
                      n1553 = local write "Câmara 2"(w1745) -> ()
                      n1554 = call-poly <vilib>:"DAQmx Create Virtual Channel.vi"("lines"=tag "Dev1/port0/line3") -> ("task out"=w1756:refnum<k21>, "error out"=w1755:errorcluster)  [unwired: 13 in]
                      n1555 = call <vilib>:"DAQmx Start Task.vi"("task/channels in"=w1756, "error in"=w1755) -> ("task out"=w1754:refnum<k21>, "error out"=w1753:errorcluster)  [unwired: 12 in]
                      n1556 = call-poly <vilib>:"DAQmx Write.vi"("task/channels in"=w1754, "data"=w1745, "error in"=w1753) -> ("task out"=w1749:refnum<k21>, "error out"=w1748:errorcluster)  [unwired: 10 in, 1 out]
                      n1557 = call <vilib>:"DAQmx Stop Task.vi"("task/channels in"=w1749, "error in"=w1748) -> ("task out"=w1751:refnum<k21>, "error out"=w1752:errorcluster)  [unwired: 12 in]
                      n1558 = call <vilib>:"DAQmx Clear Task.vi"("task in"=w1751, "error in"=w1752) -> ("error out"=w1746:errorcluster)  [unwired: 13 in]
                      n1559 = call <vilib>:"Simple Error Handler.vi"("type of dialog (OK msg:1)"=w1747, "error in (no error)"=w1746) -> ()  [unwired: 3 in, 5 out]
                    }
                  }
                }
              }
            }
          }
          n1560 = Index Array(array=w273, index=w271) -> (element=w270:dbl)
          n1561 = Index Array(array=w272, index=w271) -> (element=w269:dbl)
          n1562 = Bundle("Real 2D Array"=w276, "Best Linear Fit"=w288) -> (w287:T9)  [unwired: 1 in]
          n1563 = Bundle("Real 2D Array"=w276, "Best Polynomial Fit"=w277) -> (w274:T10)  [unwired: 1 in]
          n1564 = Bundle("Real 2D Array"=w276, "Best Polynomial Fit"=w278) -> (w275:T10)  [unwired: 1 in]
          n1565 = Build Array(w286, w287, w274) -> (→"Linear T":T11)
          n1566 = Bundle("Real 2D Array"=w276, "Best Linear Fit"=w283) -> (w284:T9)  [unwired: 1 in]
          n1567 = case shown="True" w268 {
            tunnel: w270 -> [_ w1759]
            tunnel: w269 -> [_ w1758]
            tunnel: w263 -> [_ w1757]
            frame False {
            }
            frame True {
              "P fit" <- w1759
              "T fit" <- w1758
              "P (bar/s)" <- w1757
            }
          }
          n1568 = Build Array(w285, w284, w275) -> (→"Linear P":T11)
          n1569 = property on="ON/OFF" class="Bool (strict)"() -> ("Value"=w243:bool)  [unwired: 2 in, 2 out]
          n1570 = case shown="True" w243 {
            frame False {
            }
            frame True {
              n1571 = property on="Auto Ctrl" class="Bool (strict)"() -> ("Value"=w294:bool)  [unwired: 2 in, 2 out]
              n1572 = case shown="False" w294 {
                tunnel: [w299 w303] -> w297
                tunnel: [w300 w302] -> w298
                tunnel: [w301 w304] -> w296
                frame False {
                  n1573 = property on="S#01" class="DigNum (strict)"() -> ("Value"=w301:dbl)  [unwired: 2 in, 2 out]
                  n1574 = property on="termopar K" class="DigNum (strict)"() -> ("Value"=w300:dbl)  [unwired: 2 in, 2 out]
                  n1575 = property on="T fit" class="DigNum (strict)"() -> ("Value"=w299:dbl)  [unwired: 2 in, 2 out]
                }
                frame True {
                  n1576 = property on="T fit" class="DigNum (strict)"() -> ("Value"=w303:dbl)  [unwired: 2 in, 2 out]
                  n1577 = property on="termopar K 2" class="DigNum (strict)"() -> ("Value"=w302:dbl)  [unwired: 2 in, 2 out]
                  n1578 = property on="S#1_auto" class="DigNum (strict)"() -> ("Value"=w304:dbl)  [unwired: 2 in, 2 out]
                }
              }
              n1579 = Merge Signals(w296, w297, w298) -> (w295:dynamicdata)
              n1580 = property on="Waveform Chart 2" class="WFChart (strict)"("Value"=w295) -> ()  [unwired: 2 in, 2 out]
            }
          }
          "Contador" <- w267
        }
        n1581 = local write "P subarray 2"(dbl[] [0.0, 1.0] ("subarray")) -> ()
        n1582 = local write "T subarray 3"(dbl[] [0.0, 1.0] ("subarray")) -> ()
      }
    }
    n1583 = Or(x=w43, y=w42) -> (x .or. y?=w44:bool)
    n1584 = Or(x=w44, y="Refresh Button") -> (x .or. y?=w46:bool)
    n1585 = case shown="True" w46 {
      frame False {
      }
      frame True {
        n1586 = stacked-sequence {
          frame #0 {
            n1587 = property on="Waveform Chart P 2" class="WFChart (strict)"("History Data"=dbl[][] []) -> ()  [unwired: 2 in, 2 out]
          }
          frame #1 {
            n1588 = property on="path RLC_mean" class="Path"() -> ("Value"=w80:path)  [unwired: 2 in, 2 out]
            n1589 = Open/Create/Replace File(file path (use dialog)=w80, operation (0:open)=T3."open", access (0:read/write)=enum16{"read/write", "read-only", "write-only"}."read-only") -> (refnum out=w84:refnum<file>, error out=w83:errorcluster)  [unwired: 3 in, 1 out]
            n1590 = Read from Text File(file (use dialog)=w84, error in=w83) -> (refnum out=w89:refnum<file>, text=w85:string, error out=w88:errorcluster)  [unwired: 2 in, 1 out]
            n1591 = Close File(refnum=w89, error in=w88) -> ()  [unwired: 2 out]
            n1592 = Search/Split String(string=w85, search string/char (-)="SET\tDATE\tTIME\t\tP (BAR)\tT (ºC)\tC-50-L\tC-50-N\tC-100-L\tC-100-N\tC-1K-L\tC-1K-N\tC-10K-L\tC-10K-N\tZ-50-L\tZ-50-N\tZ-100-L\tZ-100-N\tZ-1K-L\tZ-1K-N\tZ-10K-L\tZ-10K-N") -> (match + rest of string=w90:string)  [unwired: 1 in, 2 out]
            n1593 = String Subset(string=w90, offset (0)=150) -> (substring=w97:string)  [unwired: 1 in]
            n1594 = Spreadsheet String To Array(format string="%#g", spreadsheet string=w97) -> (array=w96:dbl[][])  [unwired: 2 in]
            n1595 = Transpose Matrix(1:w96) -> (0:w110:dbl[][])
            n1596 = Index Array(array=w110, index (row)=1 ("index (row) 4")) -> (element=w111:dbl[])  [unwired: 1 in]
            n1597 = Index Array(array=w110, index (row)=2 ("index (row) 5")) -> (element=w112:dbl[])  [unwired: 1 in]
            n1598 = Index Array(array=w110, index (row)=3 ("index (row) 2")) -> (element=w113:dbl[])  [unwired: 1 in]
            n1599 = Index Array(array=w110, index (row)=4 ("index (row) 3")) -> (element=w114:dbl[])  [unwired: 1 in]
            n1600 = Index Array(array=w110, index (row)=5 ("index (row) 4")) -> (element=w115:dbl[])  [unwired: 1 in]
            n1601 = Index Array(array=w110, index (row)=6 ("index (row) 5")) -> (element=w116:dbl[])  [unwired: 1 in]
            n1602 = Index Array(array=w110, index (row)=7 ("index (row) 2")) -> (element=w117:dbl[])  [unwired: 1 in]
            n1603 = Index Array(array=w110, index (row)=8 ("index (row) 3")) -> (element=w118:dbl[])  [unwired: 1 in]
            n1604 = Index Array(array=w110, index (row)=9 ("index (row) 4")) -> (element=w79:dbl[])  [unwired: 1 in]
            n1605 = Index Array(array=w110, index (row)=10 ("index (row) 5")) -> (element=w78:dbl[])  [unwired: 1 in]
            n1606 = Index Array(array=w110, index (row)=11 ("index (row) 2")) -> (element=w77:dbl[])  [unwired: 1 in]
            n1607 = Index Array(array=w110, index (row)=12 ("index (row) 3")) -> (element=w76:dbl[])  [unwired: 1 in]
            n1608 = Index Array(array=w110, index (row)=13 ("index (row) 4")) -> (element=w75:dbl[])  [unwired: 1 in]
            n1609 = Index Array(array=w110, index (row)=14 ("index (row) 5")) -> (element=w74:dbl[])  [unwired: 1 in]
            n1610 = Index Array(array=w110, index (row)=15 ("index (row) 2")) -> (element=w73:dbl[])  [unwired: 1 in]
            n1611 = Index Array(array=w110, index (row)=16 ("index (row) 3")) -> (element=w72:dbl[])  [unwired: 1 in]
            n1612 = Build Array(w111, w112, w113, w114, w115, w116, w117, w118, w79, w78, w77, w76, w75, w74, w73, w72) -> (w71:dbl[][])
            n1613 = Transpose Matrix(1:w71) -> (0:→"Waveform Chart P 2":dbl[][])
          }
        }
      }
    }
  }
  n1614 = local write "path 2_cinetica"(path "C:/H2_Painel/painel_auto/cinetica.txt" ("path")) -> ()
  n1615 = local write "path RLC_completo"(path "C:/H2_Painel/painel_auto/RLC_full.txt" ("path RLC_mean")) -> ()
  n1616 = local write "path RLC_mean"(path "C:/H2_Painel/painel_auto/RLC_mean.txt" ("path RLC_mean")) -> ()
  n1617 = local write "path"(path "C:/H2_Painel/painel_auto/Arquivo_Padrao.txt" ("path")) -> ()
  n1618 = local write "path 2"(path "C:/H2_Painel/painel_auto/Arquivo_PadraoS1.txt" ("path")) -> ()
